vi "Mapper-main.vi"() -> ()   [LabVIEW 2022 SP3]
doc: "Demonstrates the fundamentals of the State Machine design pattern in LabVIEW. A state machine, in its simplest form, is a case structure within a while loop, with a state enum wired to a shift register on the loop to define the execution of different cases (or \"states\") of the case structure on different iterations of the loop."
uses:
  Subsystem modules/Messenger service/MessengerLib.lvlib
  Datatypes/TopStates.ctl
  Subsystem modules/Magnet module/ctl/Magnet Orders.ctl
  Subsystem modules/Magnet module/Magnet module.lvlib
  Subsystem modules/Magnet module/ctl/MSG to magnet.ctl
  Subsystem modules/Servo drive module/ctl/Axis names.ctl
  Subsystem modules/Servo drive module/Servo drive module.lvlib
  Subsystem modules/Servo drive module/ctl/Servo MSG.ctl
  Subsystem modules/Servo drive module/ctl/Servo commands.ctl
  Subsystem modules/Magnet module/ctl/SetField data.ctl
  Subsystem modules/Magnet module/ctl/RampingOutput.ctl
  Subsystem modules/Magnet module/ctl/Magnet mode.ctl
  Subsystem modules/Magnet module/ctl/Overall status.ctl
  Subsystem modules/Magnet module/ctl/TM Revision.ctl
  Subsystem modules/Servo drive module/ctl/Servo constants.ctl
  Subsystem modules/Servo drive module/ctl/Servo variables.ctl
  Subsystem modules/Servo drive module/ctl/Servo state.ctl
  Subsystem modules/Servo drive module/ctl/Status variable change.ctl
  Datatypes/Connected modules.ctl
  Subsystem modules/THz module/ctl/THz Message for module.ctl
  Subsystem modules/THz module/THz source modeule.lvlib
  Subsystem modules/Lock-in module/ctl/MFLI_command enum.ctl
  Subsystem modules/Lock-in module/Lock-in module.lvlib
  Subsystem modules/Lock-in module/ctl/MFLI_message for module.ctl
  Subsystem modules/Sample rotator/ctl/Rotator commands.ctl
  Subsystem modules/Sample rotator/SampleRotator.lvlib
  Subsystem modules/Magnet module/ctl/Magnet mode public.ctl
  Subsystem modules/Magnet module/ctl/Actual magnet state.ctl
  Subsystem modules/Sample rotator/ctl/Rotator controller info.ctl
  Subsystem modules/Sample rotator/ctl/Axis status.ctl
  Subsystem modules/Sample rotator/ctl/Positoin to set.ctl
  Subsystem modules/Sample rotator/ctl/Motion Properties.ctl
  Subsystem modules/Lock-in module/ctl/MFLI parameters.ctl
  <instrlib>/Zurich Instruments LabOne/Public/Data/ziTypeDemodSampleSingle.ctl
  <instrlib>/Zurich Instruments LabOne/Zurich Instruments LabOne.lvlib
  <instrlib>/Zurich Instruments LabOne/Public/ziTypeHandle.ctl
  Subsystem modules/THz module/ctl/THz sweep parameters.ctl
  Subsystem modules/THz module/ctl/Synth configs.ctl
  Subsystem modules/THz module/ctl/VDI config constants.ctl
  Subsystem modules/Sample rotator/ctl/MSG to Rotator.ctl
  Subsystem modules/Temperature control module/ctl/TC sensors.ctl
  Subsystem modules/Temperature control module/Temperature controller.lvlib
  Subsystem modules/Temperature control module/ctl/MSG for VTI.ctl
  Subsystem modules/Magnet module/ctl/Cryostat temperature sensors.ctl
  Datatypes/experiment state.ctl
  Subsystem modules/Temperature control module/ctl/TC commands.ctl
  Subsystem modules/Lock-in module/ctl/ACQ info.ctl
  Datatypes/SampleHolders.ctl
  <userlib>/_OpenG.lib/variantconfig/variantconfig.llb/openg_variant_configuration_file.lvlib
  <vilib>/Utility/config.llb/NI_LVConfig.lvlib
  Datatypes/Instr Info.ctl
  Subsystem modules/Lock-in module/ctl/MFLI_parameter and value.ctl
  Datatypes/Single servo status.ctl
  Datatypes/Measurement info.ctl
  Subsystem modules/Temperature control module/ctl/Set point.ctl
  Datatypes/THz parameters.ctl
  Subsystem modules/Lock-in module/ctl/MFLI_node.ctl
  <vilib>/Utility/sysdir.llb/System Directory Type.ctl
  Datatypes/Map parameters.ctl
  Datatypes/Map graph data.ctl
  Subsystem modules/THz module/ctl/THz commands enum.ctl
  Subsystem modules/Lock-in module/ctl/OSC sampling rate.ctl
  <vilib>/Analysis/NI_AALPro.lvlib
  <vilib>/Analysis/2dsp.llb/Decimate (single shot, DBL).vi
  Subsystem modules/Lock-in module/ctl/ADQ data.ctl
  Subsystem modules/Source meter/ctls/SMU status.ctl
  Subsystem modules/Source meter/Source meter.lvlib
  Subsystem modules/Source meter/ctls/SMU Commands.ctl
  Subsystem modules/Source meter/ctls/MSG to SMU.ctl
  Subsystem modules/Power monitor/PwrM status.ctl
  Subsystem modules/Power monitor/Power monitor.lvlib
  Datatypes/Magnet controls.ctl
  Datatypes/Servo controls.ctl
  Subsystem modules/Temperature control module/ctl/Set temperature.ctl
  Subsystem modules/Source meter/ctls/SMU settings.ctl
panel:
  in  "MW trig low [s]":dbl=0.5 format="%#_13g"
  out "data delay":dbl format="%.4g"
  out "Instr status":T1 caption="Connected \ninstuments"
  in  "Counter":u32
  out "rows":i32
  out "cols":i32
  out "tdms map file out":refnum<k34>
  in  "Line rate":dbl(ring)=1.118481 items=["1,1s"=1.118481, "2,2s"=2.236962, "4,5s"=4.473924, "9s"=8.947848]
  out "Controls referencies":T2
  out "Tmp [K]":T3
  out "Busy":bool
  in  "Stop":bool
  out "Review results":T4[](array[typedef])
  out "Magnetic\nfield state":bool
  out "data time":timestamp
  out "New data":bool
  out "Data":T5
  out "Instr control refs":refnum<vi>[](array[refnum])
  out "Tmp reched time":dbl format="%<%H:%M:%S>T"
  out "VTI tmp reached":bool
  out "Running experiment":bool
  out "Temperature log ref":refnum<file>
  out "1 round\ntime":u32
  out "loggersRef":refnum<file>
  in  "Tab Control":T6(tab)
  out "Drift[K/min]":dbl[](array[numeric])
  in  "Log folder":path=path "C:/HFEPR logs"
  in  "Disconnect":bool
  in  "Select module":T7(ring)
  out "Logger":string[](array[string])
  in  "Re-connect instruments":bool
  in  "System config file path":path=path "M:/Instrument/HFEPR spectrometer/Software developement/Multi-EPR plus ultra/SystemData/config.ini"
  out "Instr info":T8 {"PwrMonitor"."Last update" format="%<%H:%M:%S>T"; "VTI"."Last update" format="%<%H:%M:%S>T"; "PMD"."Last update" format="%<%H:%M:%S>T"; "SMU"."Last update" format="%<%H:%M:%S>T"; "Servo"."Last update" format="%<%H:%M:%S>T"; "Rotator"."Axes"."Actuator" items=["Linear", "Roatator", "Goniometer"]; "Rotator"."Name" items=["ANC350res", "ANC350num", "ANC350fps", "Unknown"]; "Rotator"."Last update" format="%<%H:%M:%S>T"; "THz"."Last update" format="%<%H:%M:%S>T"; "MFLI"."Last update" format="%<%H:%M:%S>T"; "Magnet"."Last update" format="%<%H:%M:%S>T"}
  in  "Use previous settings":bool=TRUE
  out "Temperature monitor":T12(graph)
  in  "Real instruments":bool=TRUE
  in  "Password is admin":string
  in  "Sample holder":T13
  in  "Acquisition controls":T15={"ACQ parameters"={"Filter order"=7.0, "Filter tau [ms]"=10.0, "F_Mod [kHz]"=1.0, "Amp_Mod [mV]"=10.0, "Enable output"=0, "Phase [°]"=0.0}, "ACQ shot btn"=FALSE, "Modulation [A]"=0.0, "In50"=FALSE, "Out50"=FALSE, "DemEn"=FALSE, "Mod_A [G]"=0.0} {"ACQ parameters"."Enable output" items=["Disable", "Enable"]; "ACQ parameters"."Amp_Mod [mV]" min=0.0 max=10000.0 format="%#_5f"; "ACQ parameters"."F_Mod [kHz]" min=0.1 max=500.0 format="%#_5f"; "ACQ parameters"."Filter order" min=1.0 max=10.0 step=1.0; "ACQ parameters"."Filter tau [ms]" min=0.0 max=1000.0 step=1.0 format="%#_4f"}
  in  "VID control":T16={"AMC"=9, "Multip"=1, "Base frequency [GHz]"=0.0, "End frequency [GHz]"=0.0, "Im frequency [MHz]"=1500.0, "Sweep up [ms]"=0.0, "Reset trigger?"=FALSE} {"Multip" items=["1"=1, "2"=2, "3"=3, "4"=4, "6"=6, "8"=8, "9"=9]; "AMC" items=["9"=9, "12"=12]; "End frequency [GHz]" min=0.00018 max=20000.0; "Base frequency [GHz]" min=162.0 max=252.0 format="%_5g"}
  in  "Servo controls":T17={"Y left"=FALSE, "Y right"=FALSE, "X backward"=FALSE, "X forward"=FALSE, "Zdown"=FALSE, "Zup"=FALSE, "Step\n[mm]"=5.0, "QO table"={"ZLdown"=FALSE, "ZLup"=FALSE, "ZRup"=FALSE, "ZRdown"=FALSE, "ZMdown"=FALSE, "ZMup"=FALSE}, "X"=0.0, "Y"=0.0, "ZL"=0.0, "ZR"=0.0, "ZM"=0.0, "Measure Position btn"=FALSE, "Eject position btn"=FALSE, "Stop servo btn"=FALSE, "Save position btn"=FALSE} {"Step\n[mm]" min=0.0 max=600.0 step=5.0}
  in  "Magnet controls":T18 {"Output\n[T]" scale=0.0..16.0; "Field\n[T]" scale=0.0..16.0; "Desired ramp\nrate [mT/s]" max=7.544966; "Set Field [T]" max=16.0}
  out "lookup":cluster{"X (Vrms)":dbl, "Y (Vrms)":dbl}(graph) caption="Waveform Chart - Dark"
  in  "SMU controls":T20={"Apply"=FALSE, "Measurement settings"={"Source Mode "=1, "Source Level"=0.001, "Source Limit"=0.3, "Measure Function"=0, "Remote sense"=TRUE, "Clear buffer?"=FALSE, "Beep"=TRUE, "High Capacity"=TRUE, "Terminals"=0, "PLCs"=1.0, "Fast measurement"=FALSE}, "Value"=0.1006, "Stop"=FALSE, "Record"=FALSE, "B[T]"=0.0, "Refresh"=FALSE} {"Value" format="%#_3e"; "Measurement settings"."Measure Function" items=["Volts", "Current", "Auto Resistance", "Manual Resistance", "Digitize Voltage", "Digitize Current"]; "Measurement settings"."Source Level" max=0.3; "Measurement settings"."Source Mode" items=["Voltage", "Current"]; "Measurement settings"."Terminals" items=["Front", "Rear"]}
  in  "VTI control":T21={"VTI space [K]"=1.0, "Sample [K]"=0.0, "Heater3 [K]"=1.8, "Heater4 [K]"=1.8, "Out 1 [%]"=0.0, "Out 2 [%]"=0.0, "Range out 1"=1} {"Range out 1" items=["Off", "Range 1 (On)", "Range 2", "Range 3", "Range 4", "Range 5"]; "Heater4 [K]" min=1.8 max=300.0; "Heater3 [K]" min=1.8 max=300.0}
  in  "Operator":string="Unknown"
  in  "Map parameters":T22={"B_start[T]"=0.0, "B_End[T]"=0.2, "B_rate [mT/s]"=1.0, "F_start[GHz]"=295.0, "F_end[GHz]"=0.0, "Sampling rate"=13, "Tmp [K]"=295.0, "Wait[min]"=0.0, "Points"=4096, "Display signal"=enum."X", "Signal treat"=enum."None", "Sweep [s]"=2.0} {"Points" min=4096 max=5000000; "Sampling rate" items=["117 ks/S"=9, "58.6 kS/s"=10, "29.3 kS/s"=11, "14.6 kS/s"=12, "7.32 kS/s"=13, "3.66 kS/s"=14, "1.83 kS/s"=15]}
  out "EPR map":sgl[][](graph)
  in  "Folder path":path
  in  "Description":string
  in  "Sample name":string="Unknown"
  in  "Run MAP btn":bool
  in  "Direct stop meas. btn":bool
  out "Infobar":T24 {"Started" format="%<%H:%M:%S>T"; "Remains" format="%<%H:%M:%S>t"}
  out "Spectrum":dbl[](graph)
  in  "File Path Control":path
  out "Cursor Amplitude":dbl
  out "Cursor [T]":dbl
  out "Cursor [GHz]":dbl
  out "Review Header":string[](array[string])
  out "EPR review graph":cluster{"X":dbl, "Y":dbl}[](graph)
  out "FDMR review graph":dbl[](graph)
  out "Map review graph":dbl[][](graph)
  in  "Open measurement":bool
  in  "Data file to show":u16(ring) items=["Empty", "Empty", "Empty"]
  # "Action part"
  # "Status part"
  # "Option 1:\nchoice primary and secondary sweep\n\nOption 2:\nChoice measurement mode, and appropriate cluster will apear. Other clusters wil be hidden.\n\n\nOption 3:\nChoice measurement mode.\nInternal parts of single cluster will (dis)apear if needed.\n\nNote:\nPosibility to do an orientation/temperature deppendency."
  # "Tmp [K]"
  # "Position [mm]"
  # "Z"
  # "X/Y"
  # "This software was developed for HFEPR spectrometer in 2019 (2020) at CEITEC BUT by members of MOTES research group.\n\nQuick guide:\n1) Re-connect to all instruments.\n2) Check if necessary instruments are ready. (At least VTI, VDI, Lock-In, and Magnet has to work)\n3) Go to Adjustment tab and set up Lock-in parameters as well as VDI multipiers.\n4) Go to EPR measurement tab, select folder path, fill the sample description.\n5) Fill at least 1 line of the script and press Run script button.\n\n6) In case of a bug please report this to software developer or make a note into developement diary loaceted at:\n    RG-1-12/Instriments/HFEPR spectrometer/Software developement.\n\nLast update: 07.02. 2020 - Script editor is working, measurement review not yet.\n\nSpecial thanks to: Luke Skywalker, my mom, Tonda's mom, Pilsner, God, Oleksi, Vinicius, Petr from parallel universe.\n\n \nTODO: Invisible controls: referencies for: adjustment controls, meas results, loggerRef,"
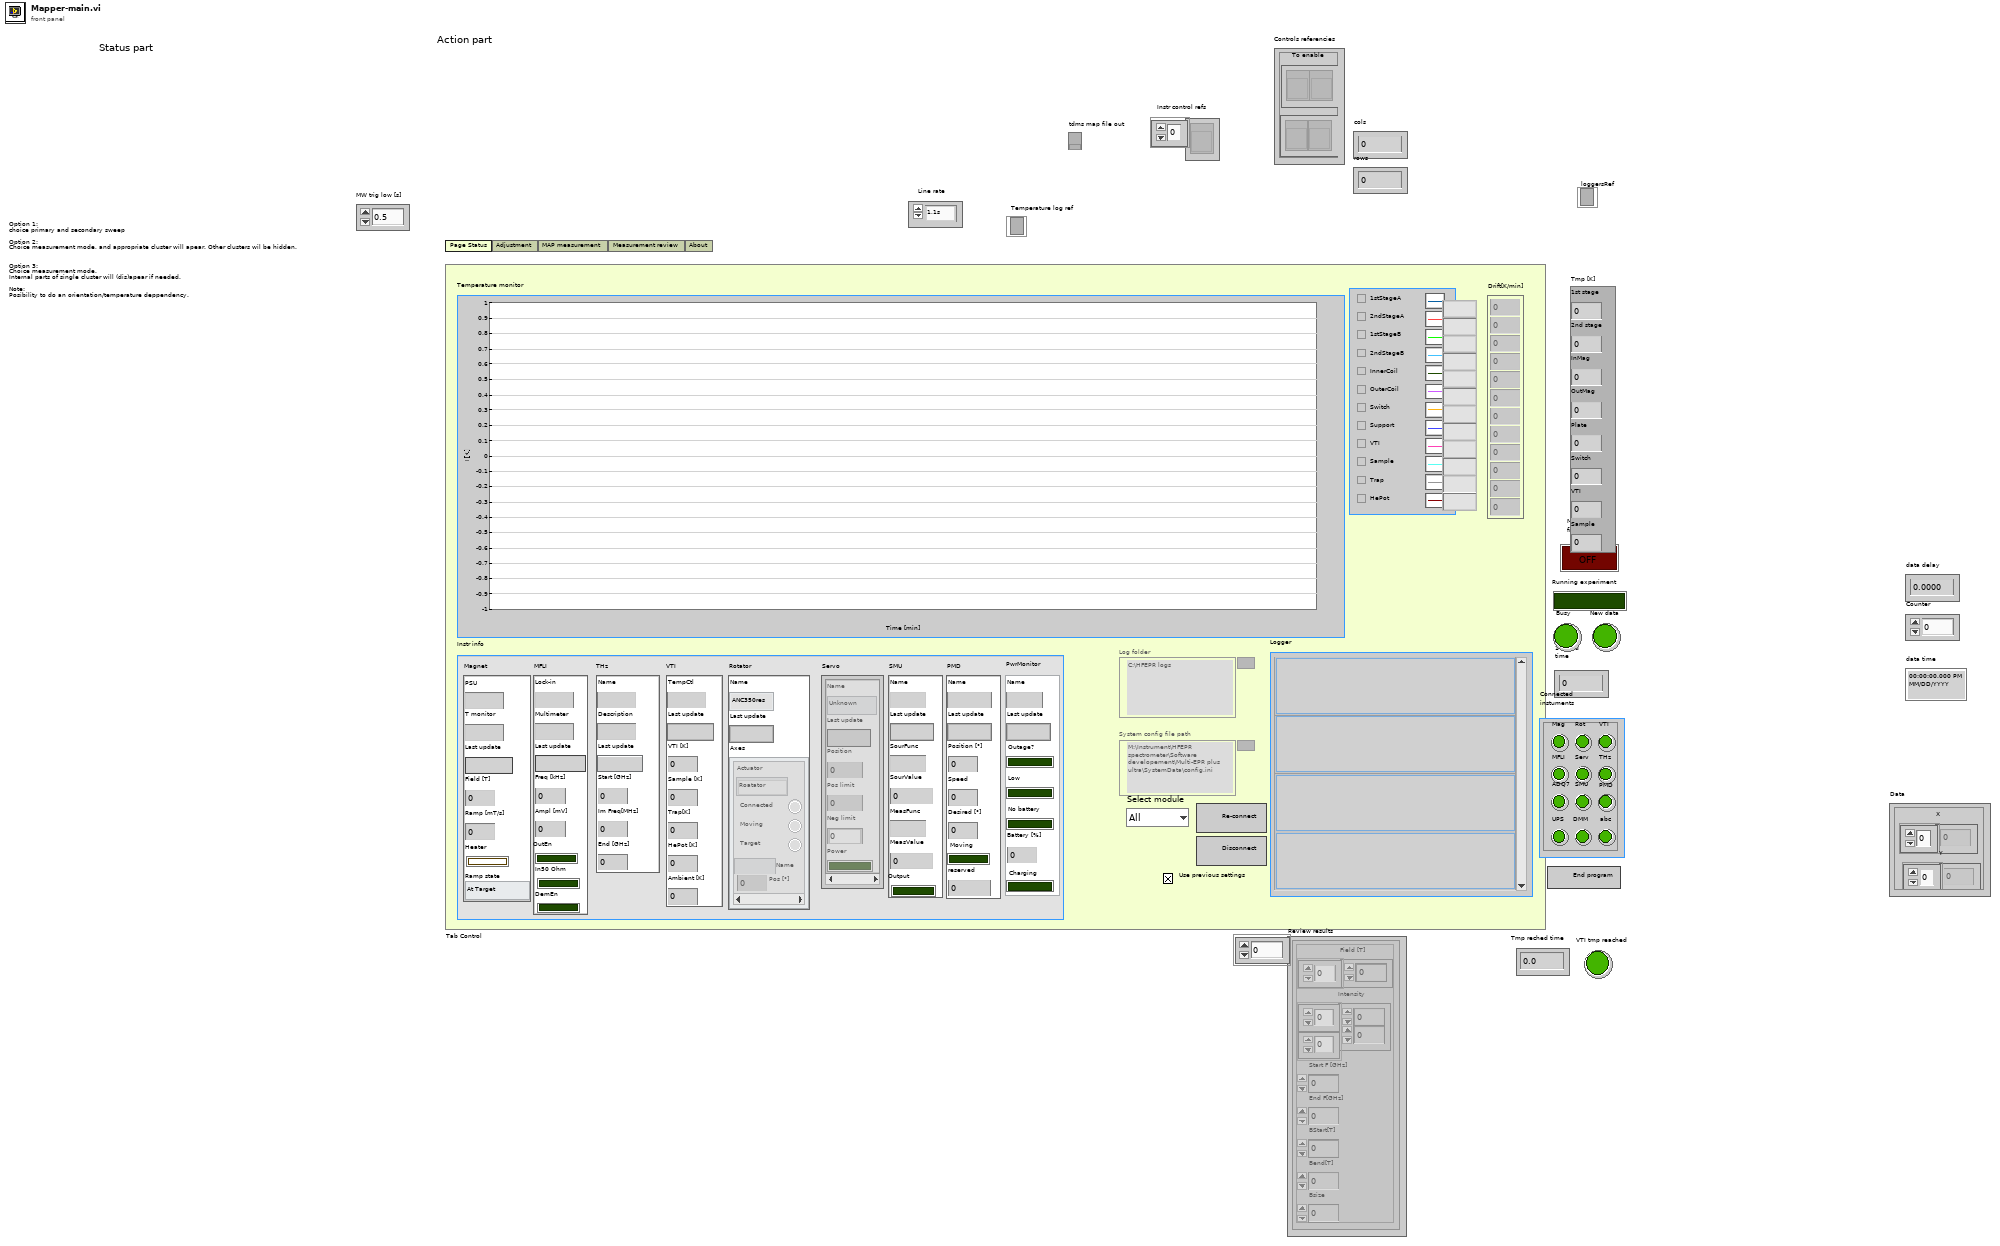
[diagram p1: front panel]
types:
  T1 = typedef "Connected modules.ctl" = cluster{"Mag":bool, "Rot":bool, "VTI":bool, "MFLI":bool, "Serv":bool, "THz":bool, "ADQ7":bool, "SMU":bool, "PMD":bool, "UPS":bool, "DMM":bool, "abc":bool}
  T2 = cluster{"To disable":refnum<vi>[], "To enable":refnum<vi>[]}
  T3 = cluster{"1st stage":dbl, "2nd stage":dbl, "InMag":dbl, "OutMag":dbl, "Plate":dbl, "Switch":dbl, "VTI":dbl, "Sample":dbl}
  T4 = typedef "Map graph data.ctl" = cluster{"Field [T]":dbl[], "Intensity":dbl[][], "Start F [GHz]":dbl, "End F[GHz]":dbl, "BStart[T]":dbl, "Bend[T]":dbl, "Bsize":i32}
  T5 = typedef "Lock-in module.lvlib/ADQ data.ctl" = cluster{"X":sgl[], "Y":sgl[]}
  T6 = enum32{"Page Status", "Adjustment", "MAP measurement", "Measurement review", "About"}
  T7 = enum16{"All", "None", "ACQ", "THz", "MAG", "SERV", "ROT", "VTI", "SMU"}
  T8 = typedef "Instr Info.ctl" = cluster{"Magnet":cluster{"PSU":string, "T monitor":string, "Last update":timestamp, "Field [T]":dbl, "Ramp [mT/s]":dbl, "Heater":bool, "Ramp state":T9}, "MFLI":cluster{"Lock-in":string, "Multimeter":string, "Last update":timestamp, "Freq [kHz]":dbl, "Ampl [mV]":dbl, "OutEn":bool, "In50 Ohm":bool, "DemEn":bool}, "THz":cluster{"Name":string, "Description":string, "Last update":timestamp, "Start [GHz]":dbl, "Im Freq[MHz]":dbl, "End [GHz]":dbl}, "VTI":cluster{"TempCtl":string, "Last update":timestamp, "VTI [K]":dbl, "Sample [K]":dbl, "Trap[K]":dbl, "HePot [K]":dbl, "Ambient [K]":dbl}, "Rotator":cluster{"Name":i32, "Last update":timestamp, "Axes":cluster{"Pos [°]":dbl, "Moving":bool, "Name":string, "Actuator":u16, "Target":bool, "Connected":bool}[]}, "Servo":T10[], "SMU":cluster{"Name":string, "Last update":timestamp, "SourFunc":string, "SourValue":dbl, "MeasFunc":string, "MeasValue":dbl, "Output":bool}, "PMD":cluster{"Name":string, "Last update":timestamp, "Position [°]":dbl, "Speed":dbl, "Desired [°]":dbl, "Moving":bool, "reserved":dbl}, "PwrMonitor":cluster{"Name":string, "Last update":timestamp, "Outage?":bool, "Low":bool, "No battery":bool, "Battery [%]":u8, "Charging":bool}}
  T9 = typedef "Magnet module.lvlib/RampingOutput.ctl" = enum16{"At Target", "Go up", "Go down"}
  T10 = typedef "Single servo status.ctl" = cluster{"Name":T11, "Last update":timestamp, "Position":dbl, "Pos limit":dbl, "Neg limit":dbl, "Power":bool}
  T11 = typedef "Servo drive module.lvlib/Axis names.ctl" = enum16{"Unknown", "AxisX", "AxisY", "AxisZ_left", "AxisZ_middle", "AxisZ_right"}
  T12 = cluster{"[0]":dbl, "[1]":dbl, "[2]":dbl, "[3]":dbl, "[4]":dbl, "[5]":dbl, "[6]":dbl, "[7]":dbl, "[8]":dbl, "[9]":dbl, "[10]":dbl, "[11]":dbl}
  T13 = typedef "SampleHolders.ctl" = enum16{"Simple", "Carousel", "Chip", "Rotator", "Liquid"}
  T14 = typedef "Lock-in module.lvlib/MFLI parameters.ctl" = cluster{"Filter order":dbl, "Filter tau [ms]":dbl, "F_Mod [kHz]":dbl, "Amp_Mod [mV]":dbl, "Enable output":u16, "Phase [°]":dbl}
  T15 = cluster{"ACQ parameters":T14, "ACQ shot btn":bool, "Modulation [A]":dbl, "In50":bool, "Out50":bool, "DemEn":bool, "Mod_A [G]":dbl}
  T16 = typedef "THz parameters.ctl" = cluster{"AMC":u16, "Multip":u16, "Base frequency [GHz]":dbl, "End frequency [GHz]":dbl, "Im frequency [MHz]":dbl, "Sweep up [ms]":dbl, "Reset trigger?":bool}
  T17 = typedef "Servo controls.ctl" = cluster{"Y left":bool, "Y right":bool, "X backward":bool, "X forward":bool, "Zdown":bool, "Zup":bool, "Step\n[mm]":dbl, "QO table":cluster{"ZLdown":bool, "ZLup":bool, "ZRup":bool, "ZRdown":bool, "ZMdown":bool, "ZMup":bool}, "X":dbl, "Y":dbl, "ZL":dbl, "ZR":dbl, "ZM":dbl, "Measure Position btn":bool, "Eject position btn":bool, "Stop servo btn":bool, "Save position btn":bool}
  T18 = typedef "Magnet controls.ctl" = cluster{"Set Field [T]":dbl, "Desired ramp\nrate [mT/s]":dbl, "Custom\nramp":bool, "Mode switch":bool, "Pause ramp":bool, "Field\n[T]":dbl, "Output\n[T]":dbl, "Equalize":bool, "Discharge":bool, "Switch \ntmp [K]":dbl, "Direction":bool}
  T19 = typedef "SMU settings.ctl" = cluster{"Source Mode ":u16, "Source Level":dbl, "Source Limit":dbl, "Measure Function":u16, "Remote sense":bool, "Clear buffer?":bool, "Beep":bool, "High Capacity":bool, "Terminals":u16, "PLCs":dbl, "Fast measurement":bool}
  T20 = cluster{"Apply":bool, "Measurement settings":T19, "Value":dbl, "Stop":bool, "Record":bool, "B[T]":dbl, "Refresh":bool}
  T21 = typedef "Temperature controller.lvlib/Set temperature.ctl" = cluster{"VTI space [K]":dbl, "Sample [K]":dbl, "Heater3 [K]":dbl, "Heater4 [K]":dbl, "Out 1 [%]":dbl, "Out 2 [%]":dbl, "Range out 1":u16}
  T22 = typedef "Map parameters.ctl" = cluster{"B_start[T]":dbl, "B_End[T]":dbl, "B_rate [mT/s]":dbl, "F_start[GHz]":dbl, "F_end[GHz]":dbl, "Sampling rate":T23, "Tmp [K]":dbl, "Wait[min]":dbl, "Points":u32, "Display signal":enum16{"X", "Y", "R", "Phi"}, "Signal treat":enum16{"None", "Unity norm", "Mean norm", "Standardization"}, "Sweep [s]":dbl}
  T23 = typedef "OSC sampling rate.ctl" = u16
  T24 = typedef "Measurement info.ctl" = cluster{"Remains":dbl, "T_sample [K]":dbl, "Last log":string, "Experiment state":T25, "Field [T]":dbl, "Sample holder":T13, "Started":timestamp}
  T25 = typedef "experiment state.ctl" = enum16{"Setup", "Preparation", "Stabilization", "Begin", "Acquisition", "Save"}
  T26 = typedef "Instr Info.ctl" = cluster{"Magnet":cluster{"PSU":string, "T monitor":string, "Last update":timestamp, "Field [T]":dbl, "Ramp [mT/s]":dbl, "Heater":bool, "Ramp state":T9}, "ACQ":cluster{"Lock-in":string, "Multimeter":string, "Last update":timestamp, "Freq [kHz]":dbl, "Ampl [mV]":dbl, "OutEn":bool, "In50 Ohm":bool, "DemEn":bool}, "THz":cluster{"Name":string, "Description":string, "Last update":timestamp, "Start [GHz]":dbl, "Im Freq[MHz]":dbl, "End [GHz]":dbl}, "VTI":cluster{"TC":string, "Last update":timestamp, "VTI [K]":dbl, "Sample [K]":dbl, "Trap[K]":dbl, "HePot [K]":dbl, "Ambient [K]":dbl}, "Rot":cluster{"Name":u16, "Last update":timestamp, "Actuator":u16, "Connected":bool, "Moving":bool, "Target":bool, "Cap [nF]":dbl, "Position [°]":dbl}, "Servo":T10[], "SMU":cluster{"Name":string, "Last update":timestamp, "Source F":string, "Source V":dbl, "Measure F":string, "Measure V":dbl, "Output":bool}, "PMD":cluster{"Name":string, "Last update":timestamp, "Position [°]":dbl, "Speed":dbl, "Desired [°]":dbl, "Moving":bool, "reserved":dbl}, "PwrM":T27}
  T27 = typedef "Power monitor.lvlib/PwrM status.ctl" = cluster{"Name":string, "Last update":timestamp, "Outage?":bool, "Low":bool, "No battery":bool, "Battery [%]":u8, "Charging":bool}
  T28 = typedef "TopStates.ctl" = enum16{"Initialize GUI", "Wait for Event", "Check message", "Check measurement", "Stop", "Restart"}
  T29 = typedef "MessengerLib.lvlib/Messenger referencies.ctl" = cluster{"TOP":refnum<queue>, "Instr_M":refnum<queue>, "Field_C":refnum<queue>, "Tmp_M":refnum<queue>, "Tmp_C":refnum<queue>, "Table_C":refnum<queue>, "MW_C":refnum<queue>, "Data_Aq":refnum<queue>, "Mod_M":refnum<queue>, "Field_M":refnum<queue>, "Pwr_M":refnum<queue>, "Angle_C":refnum<queue>, "Sample_C":refnum<queue>, "Reserved":refnum<queue>}
  T30 = enum16{"fire", "rainbow", "gray", "inverse gray", "ice", "original"}
  T31 = enum16{"All", "None", "ACQ", "THz", "MAG", "SERV", "ROT", "VTI"}
  T32 = enum8{"Enabled", "Disabled", "Disabled and Grayed Out"}
  T33 = typedef "Magnet module.lvlib/Magnet mode public.ctl" = enum16{"Persistant", "Ramping"}
  T34 = typedef "Magnet module.lvlib/SetField data.ctl" = cluster{"Field [T]":dbl, "Ramp [T/s]":dbl, "Custom Ramp?":bool, "Mode":T33}
  T35 = typedef "Magnet module.lvlib/Magnet Orders.ctl" = enum16{"Ignore", "Connect", "Update", "Switch mode", "Set field", "Stop ramping", "Equalize output", "Zero output", "Flip polarity", "Blackout", "Set timer", "Eval temperatures", "Disconnect"}
  T36 = typedef "Magnet module.lvlib/MSG to magnet.ctl" = cluster{"Command":T35, "Data":variant}
  T37 = typedef "Source meter.lvlib/MSG to SMU.ctl" = cluster{"Command":T38, "Data":variant}
  T38 = typedef "Source meter.lvlib/SMU Commands.ctl" = enum16{"Ignore", "Connect", "Update", "Set measurement", "Start measurement", "Get actual results", "Stop measurement", "Disconnect", "End"}
  T39 = typedef "Servo drive module.lvlib/Servo commands.ctl" = enum16{"Initialize", "Update", "Move by", "Move to", "Stop", "Ignore", "Disconnect", "End"}
  T40 = typedef "Servo drive module.lvlib/Servo MSG.ctl" = cluster{"Command":T39, "Data":variant}
  T41 = typedef "THz source modeule.lvlib/THz commands enum.ctl" = enum16{"Ignore", "Connect", "Update", "Set parameters", "Disconnect", "End"}
  T42 = typedef "THz source modeule.lvlib/THz sweep parameters.ctl" = cluster{"Start [GHz]":dbl, "End [GHz] ":dbl, "Sweep up\ntime [ms]":dbl, "Sweep down\ntime [ms]":dbl, "Intermidiate [MHz]":dbl, "Reset trigger":bool}
  T43 = typedef "THz source modeule.lvlib/THz Message for module.ctl" = cluster{"Command":T41, "Data":variant}
  T44 = typedef "Lock-in module.lvlib/MFLI_parameter and value.ctl" = cluster{"parameter":T45, "value":dbl}
  T45 = typedef "Lock-in module.lvlib/MFLI_node.ctl" = enum16{"None", "filter_order [-]", "filter_constant [ms]", "in_diff", "in_autorange", "in_imp50", "in_AC", "osc_freq [kHz]", "out_ampl [V]", "out_autorange", "out_imp50", "enable output", "enamble ampl", "scope_enable", "scope_rate", "scope_len", "scope_trigEn", "AuxOut_amplify", "Phase_deg", "AuxOut_select"}
  T46 = typedef "Lock-in module.lvlib/MFLI_command enum.ctl" = enum16{"Initialize", "Update", "Set parameters", "Set module", "Set individual parameters", "Get point", "Get array", "Disconnect", "End", "Ignore"}
  T47 = typedef "Lock-in module.lvlib/MFLI_message for module.ctl" = cluster{"Command":T46, "Data":variant}
  T48 = typedef "Temperature controller.lvlib/Set point.ctl" = cluster{"Heater":string, "Tmp [K]":dbl}
  T49 = typedef "Temperature controller.lvlib/TC commands.ctl" = enum16{"Initialize", "Update", "Stop tmp change", "Set temperature", "Set point", "Disconnect", "End", "Ignore"}
  T50 = typedef "Temperature controller.lvlib/MSG for VTI.ctl" = cluster{"Command":T49, "Data":variant}
  T51 = typedef "SampleRotator.lvlib/MSG to Rotator.ctl" = cluster{"Command":T52, "Data":variant}
  T52 = typedef "SampleRotator.lvlib/Rotator commands.ctl" = enum16{"Ignore", "Initialize", "Initialize axes", "Update", "Set parameters", "Stop movement", "Set position", "Disconnect", "End"}
  T53 = typedef "THz source modeule.lvlib/VDI config constants.ctl" = cluster{"Master":T54, "Follower":T54}
  T54 = typedef "THz source modeule.lvlib/Synth configs.ctl" = cluster{"Lower limit [GHz]":dbl, "Upper limit [GHz]":dbl, "Name":string, "Handle":string, "Description":string}
  T55 = typedef "THz source modeule.lvlib/THz Message for module.ctl" = cluster{"Command":T56, "Data":variant}
  T56 = typedef "THz source modeule.lvlib/THz commands enum.ctl" = enum16{"Ignore", "Initialize", "Update", "Set parameters", "Disconnect", "End"}
  T57 = typedef "Magnet module.lvlib/TM Revision.ctl" = cluster{"Instr Serial Number":string, "Instr Driver Revision":string, "Instr Firmware Revision":string, "Instr Model Number":string}
  T58 = typedef "Magnet module.lvlib/Overall status.ctl" = cluster{"Desired":T34, "Actual":T59}
  T59 = typedef "Magnet module.lvlib/Actual magnet state.ctl" = cluster{"Mode":T60, "Ramping output":T9, "Ready for change":bool, "Switch heater":bool, "Cooler Overheat":bool, "Coil overheat":bool, "Energized":bool, "Output [T]":dbl, "Field [T]":dbl, "Ramp[T/s]":dbl, "Switch\ntemperature [K]":dbl, "Voltage [V]":dbl, "Current direction":bool}
  T60 = typedef "Magnet module.lvlib/Magnet mode.ctl" = enum16{"Persistant", "Switching", "Ramping", "Quenched"}
  T61 = typedef "Magnet module.lvlib/Cryostat temperature sensors.ctl" = cluster{"First stage A [K]":dbl, "Second stage A [K]":dbl, "Firs stage B [K]":dbl, "Second stage B [K]":dbl, "Inner magnet [K]":dbl, "Outer Magnet [K]":dbl, "Switch [K]":dbl, "Support plate [K]":dbl, "Time stamp":dbl}
  T62 = typedef "Lock-in module.lvlib/ACQ info.ctl" = cluster{"In50":bool, "InAC":bool, "InDiff":bool, "Out50":bool, "OutEN":bool, "OutF[Hz]":dbl, "OutA[V]":dbl, "DemEN":bool, "Const[ms]":dbl, "Order[-]":i32, "Phase [°]":dbl}
  T63 = enum32{"Page Status", "Adjustment", "EPR measurement", "About"}
  T64 = typedef "Zurich Instruments LabOne.lvlib/ziTypeDemodSampleSingle.ctl" = cluster{"Timestamps (ticks)":u64, "X (Vrms)":dbl, "Y (Vrms)":dbl, "Osc Phase (deg)":dbl, "Freq (Hz)":dbl, "DIO":u32, "AuxIn0 (V)":dbl, "AuxIn1 (V)":dbl, "Trigger":u32}
  T65 = typedef "Zurich Instruments LabOne.lvlib/ziTypeHandle.ctl" = cluster{"handleValid":bool, "Conn":u64, "Path Prefix":string, "Handle":u64, "Connected":bool, "Clockbase(s)":dbl}
  T66 = typedef "Source meter.lvlib/SMU status.ctl" = cluster{"VISA name":refnum<visa-resource-name>, "Connected":bool, "Name":string, "Message":string, "Error message":string, "Min voltage":dbl, "Max voltage":dbl, "Min Current":dbl, "Max Current":dbl, "Measurement value":dbl, "Source Voltage":dbl, "Measurement":bool, "Source Current":dbl, "Source Mode":u16, "Measure Function":u16}
  T67 = typedef "Temperature controller.lvlib/TC sensors.ctl" = cluster{"VTI space":dbl, "Sample":dbl, "He pot":dbl, "Trap":dbl, "Ambient":dbl, "SetP_VTI":dbl, "SetP_Smp":dbl, "SetP_Pot":dbl, "SetP_Trap":dbl, "Range out 1":u16, "Out 1 [%]":dbl, "Out 2 [%]":dbl}
  T68 = typedef "Servo drive module.lvlib/Servo state.ctl" = cluster{"Servo variables":T69, "Servo constants":T70, "Connection":variant}
  T69 = typedef "Servo drive module.lvlib/Servo variables.ctl" = cluster{"Terget reached":bool, "Connected":bool, "Power ON":bool, "Operation mode":bool, "Actual position":dbl, "Target position":dbl}
  T70 = typedef "Servo drive module.lvlib/Servo constants.ctl" = cluster{"Name":T11, "Pos position limit [mm]":dbl, "Neg position limit [mm]":dbl, "Pos velocity limit":dbl, "Neg velocity limit":dbl, "Acceleration limit":dbl}
  T71 = typedef "Servo drive module.lvlib/Status variable change.ctl" = cluster{"Property":string, "Value":variant, "Name":T11}
  T72 = typedef "SampleRotator.lvlib/Rotator controller info.ctl" = cluster{"deviceNumber":i32, "DeviceType":i32, "ID":u32, "Serial":string, "Address":string, "connected":bool}
  T73 = typedef "SampleRotator.lvlib/Axis status.ctl" = cluster{"Axis status":cluster{"Connected":bool, "Enabled":bool, "Moving":bool, "Target":bool, "EndForward":bool, "EndBackarwd":bool, "Error":bool}, "Position [°]":dbl, "Frequency [Hz]":dbl, "Voltage [V]":dbl, "Capacitance[uF]":dbl, "Name":string, "ActuatorType":u16, "DC offset [V]":dbl, "Tolerance [m°]":dbl, "Index":u8}
  T74 = typedef "Motion Properties.ctl" = cluster{"Frequency [Hz]":dbl, "MaxErr [µm|m°]":dbl, "DC voltage [V]":dbl, "Amplitude [V]":dbl, "Position [mm|°]":dbl, "EoF":bool, "EoB":bool, "Error":bool, "Target [mm|°]":dbl}
  T75 = typedef "Positoin to set.ctl" = cluster{"Relative?":bool, "Position [°]":dbl, "Safe to move?":bool}
  T76 = typedef "NI_LVConfig.lvlib/Config Data RefNum.ctl" = refnum<k1>
  T77 = typedef "System Directory Type.ctl" = i32
  T78 = cluster{"Field [T]":dbl[], "Intensity":dbl[][], "Start F [GHz]":dbl, "End F[GHz]":dbl, "BStart[T]":dbl, "Bend[T]":dbl, "Bsize":i32}
  T79 = typedef "Mudules status.ctl" = cluster{"Mag":bool, "Rot":bool, "VTI":bool, "MFLI":bool, "Serv":bool, "THz":bool, "ADQ7":bool, "SMU":bool, "PMD":bool, "UPS":bool, "DMM":bool, "abc":bool}
  T80 = typedef "Magnet module.lvlib/Magnet config constants.ctl" = cluster{"Switch resistant [K]":dbl, "Switch superconducting [K]":dbl, "First stage critical temperature [K]":dbl, "Second stage critical temperature [K]":dbl, "Inner magnet critical temperature [K]":dbl, "Outer magnet critical temperature [K]":dbl, "Field Constant [T/A]":dbl, "Maximum Current [A]":dbl, "Maximum field [T]":dbl, "Maximum source ramp [A/s]":dbl, "Source precision [T]":dbl, "Ramp limits [A/s]":dbl[], "Field limits [T]":dbl[], "SMS":refnum<visa-resource-name>, "LSC218":refnum<visa-resource-name>}
  T81 = typedef "MessengerLib.lvlib/MSG to TOP.ctl" = cluster{"Module":T82, "Response":string, "Data":variant, "Time":timestamp}
  T82 = typedef "Module name.ctl" = enum16{"Emty", "Magnet", "VTI", "Excitation", "Servo", "Acquisition", "Rotator", "Digitizer", "SMU2450", "Carousel", "Multimeter", "Tmp monitor", "Power monitor"}
  T83 = cluster{"PSU":string, "T monitor":string, "Last update":timestamp, "Field [T]":dbl, "Ramp [mT/s]":dbl, "Heater":bool, "Ramp state":T9}
  T84 = cluster{"TC":string, "Last update":timestamp, "VTI [K]":dbl, "Sample [K]":dbl, "Trap[K]":dbl, "HePot [K]":dbl, "Ambient [K]":dbl}
  T85 = cluster{"Name":string, "Description":string, "Last update":timestamp, "Start [GHz]":dbl, "Im Freq[MHz]":dbl, "End [GHz]":dbl}
  T86 = cluster{"Lock-in":string, "Multimeter":string, "Last update":timestamp, "Freq [kHz]":dbl, "Ampl [mV]":dbl, "OutEn":bool, "In50 Ohm":bool, "DemEn":bool}
  T87 = cluster{"Name":string, "Last update":timestamp, "Source F":string, "Source V":dbl, "Measure F":string, "Measure V":dbl, "Output":bool}
  T88 = cluster{"Name":u16, "Last update":timestamp, "Actuator":u16, "Connected":bool, "Moving":bool, "Target":bool, "Cap [nF]":dbl, "Position [°]":dbl}
  T89 = enum16{"None", "Unity norm", "Mean norm", "Standardization"}
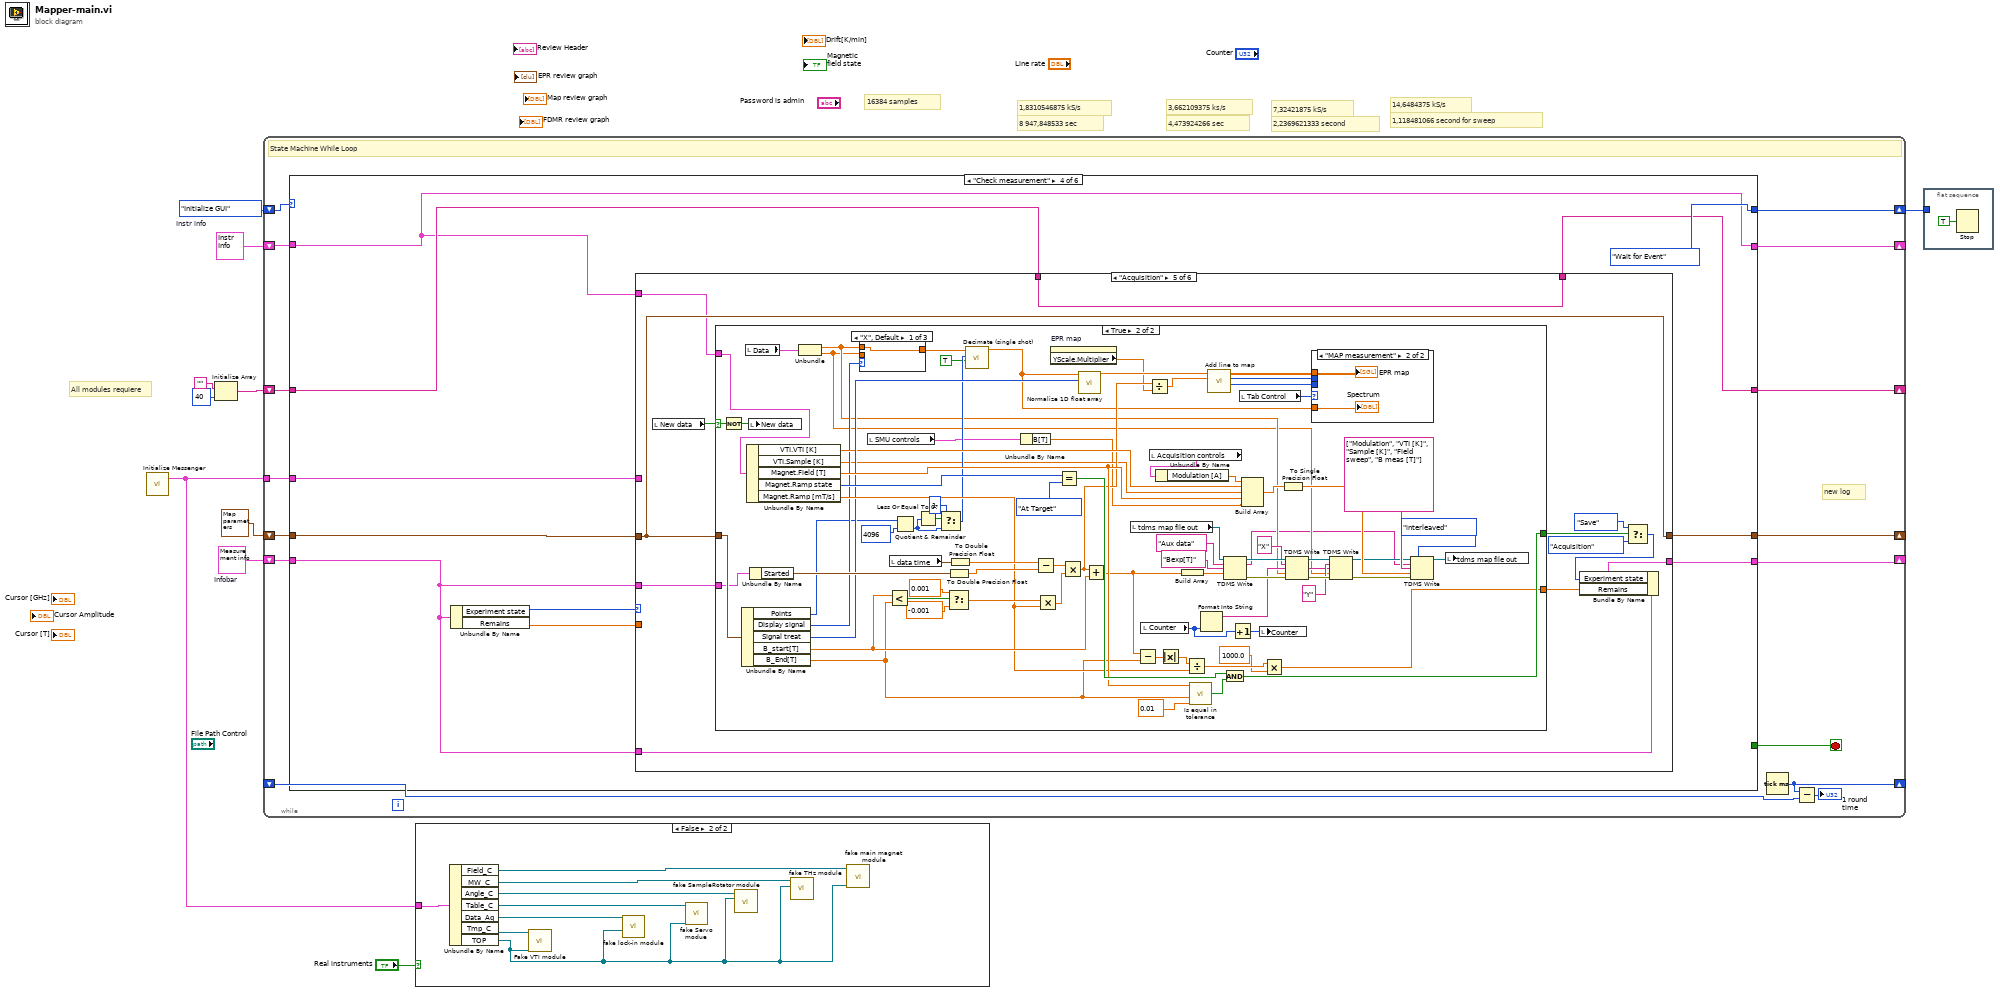
[diagram p0: block diagram]
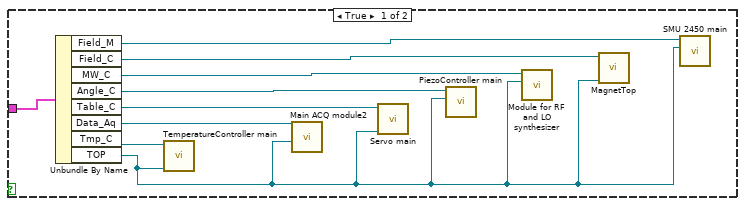
[diagram p2: hidden frame]
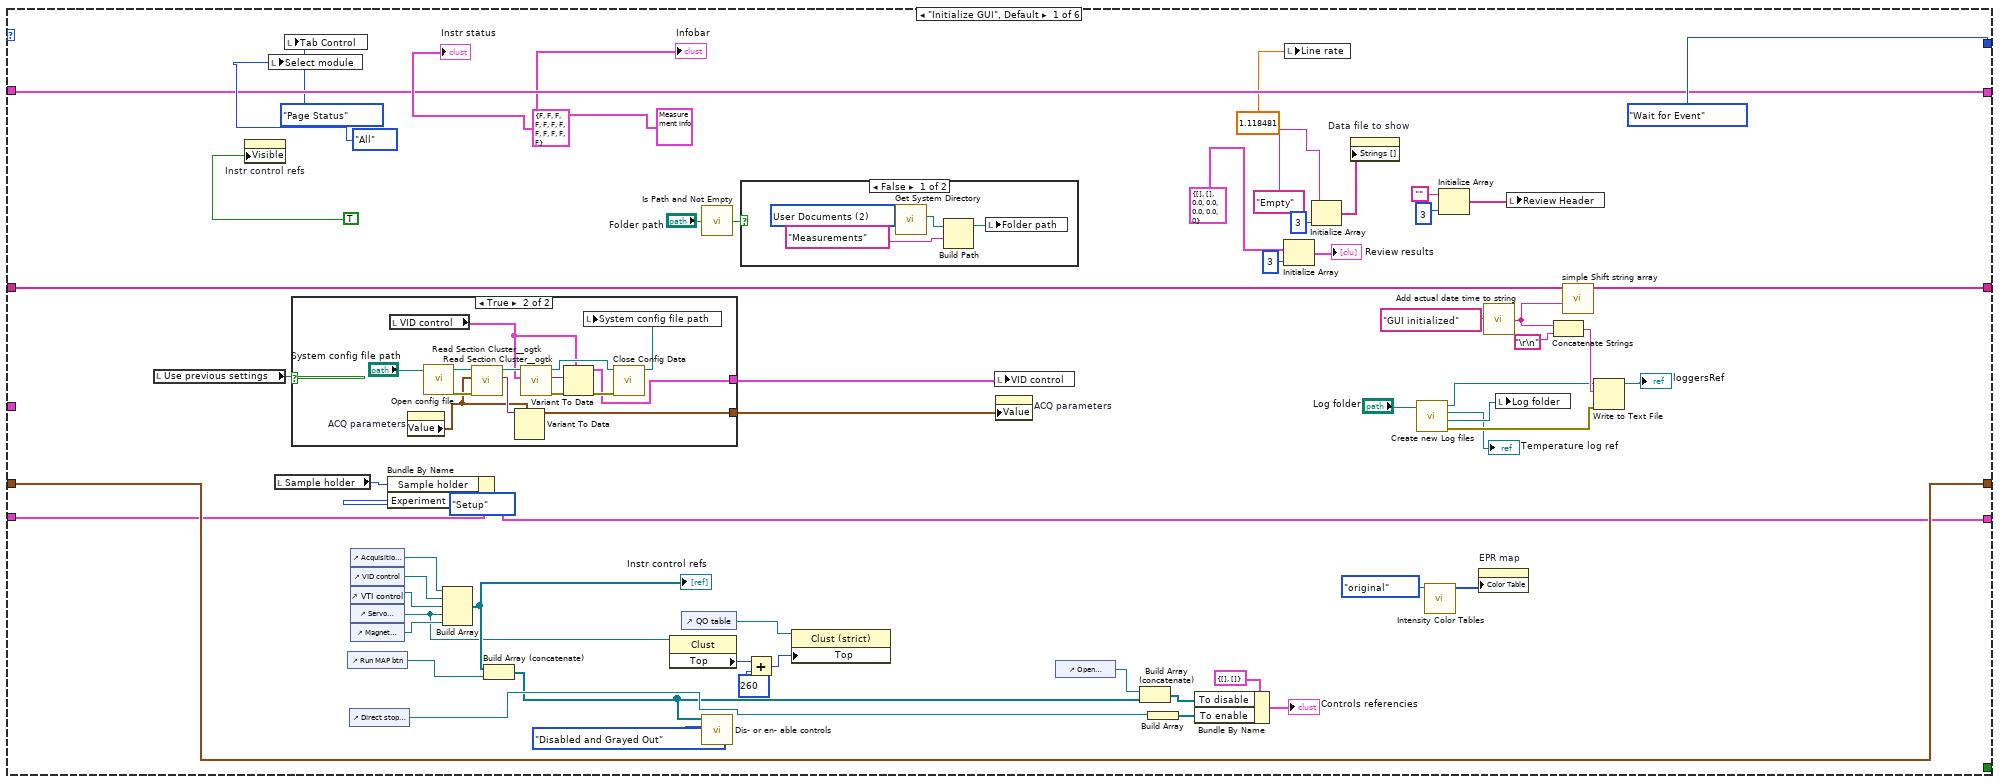
[diagram p3: hidden frame]
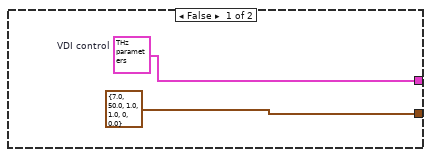
[diagram p5: hidden frame]
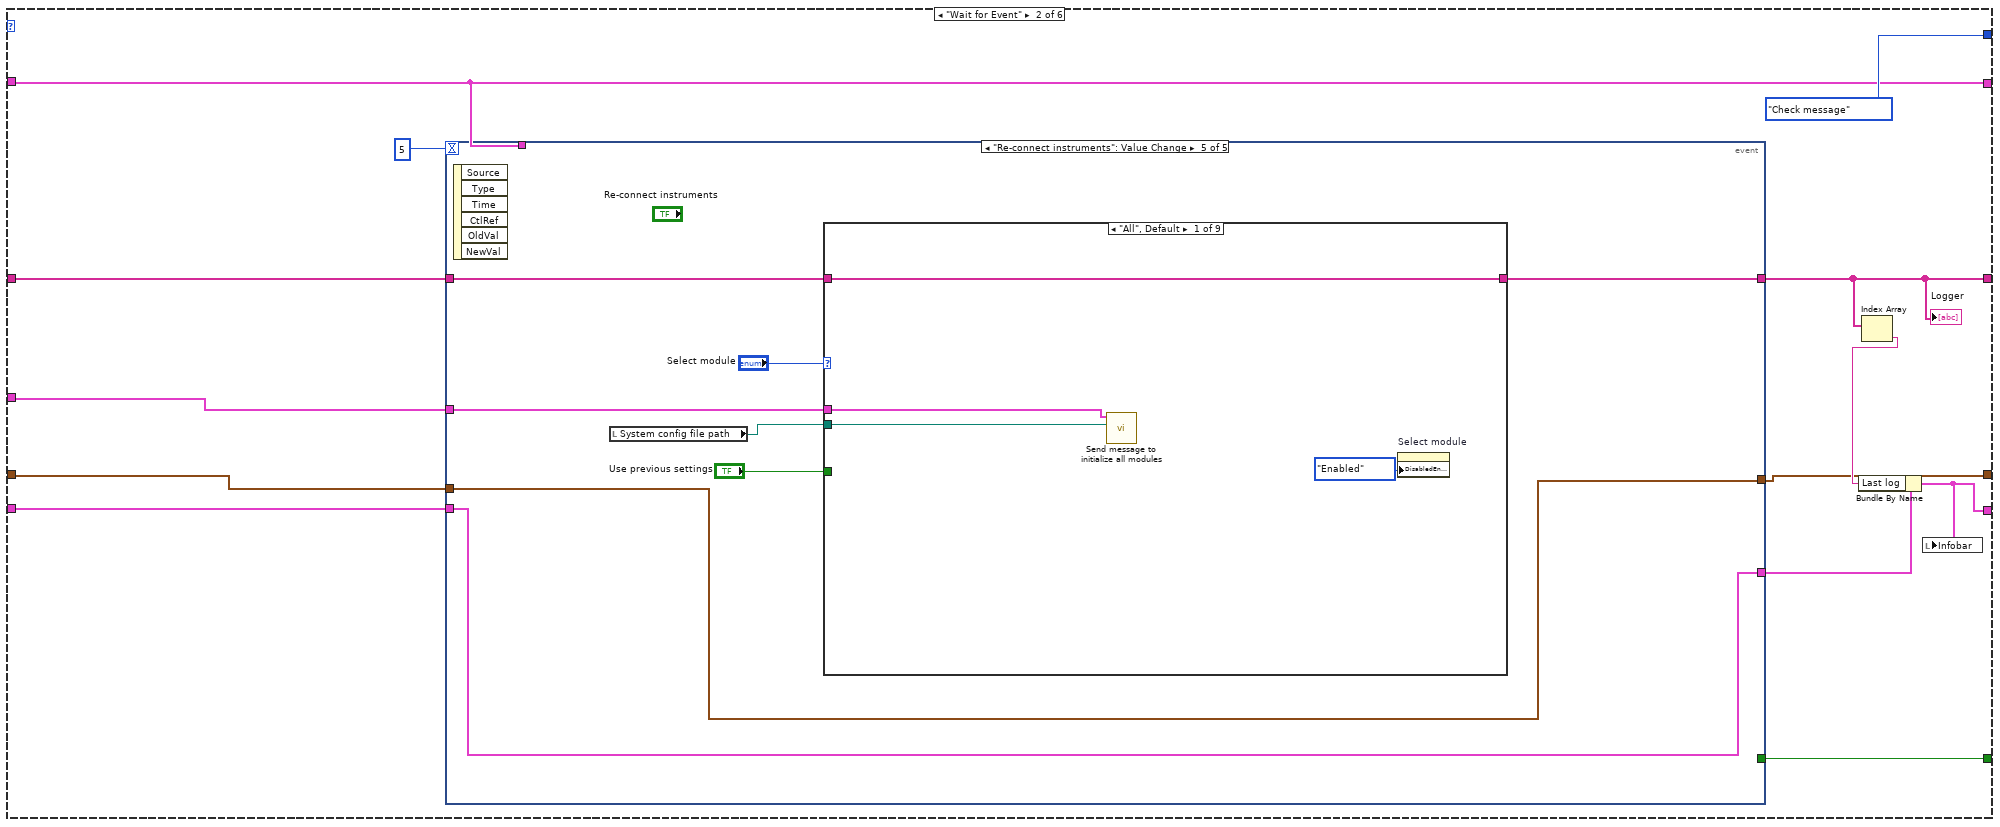
[diagram p6: hidden frame]
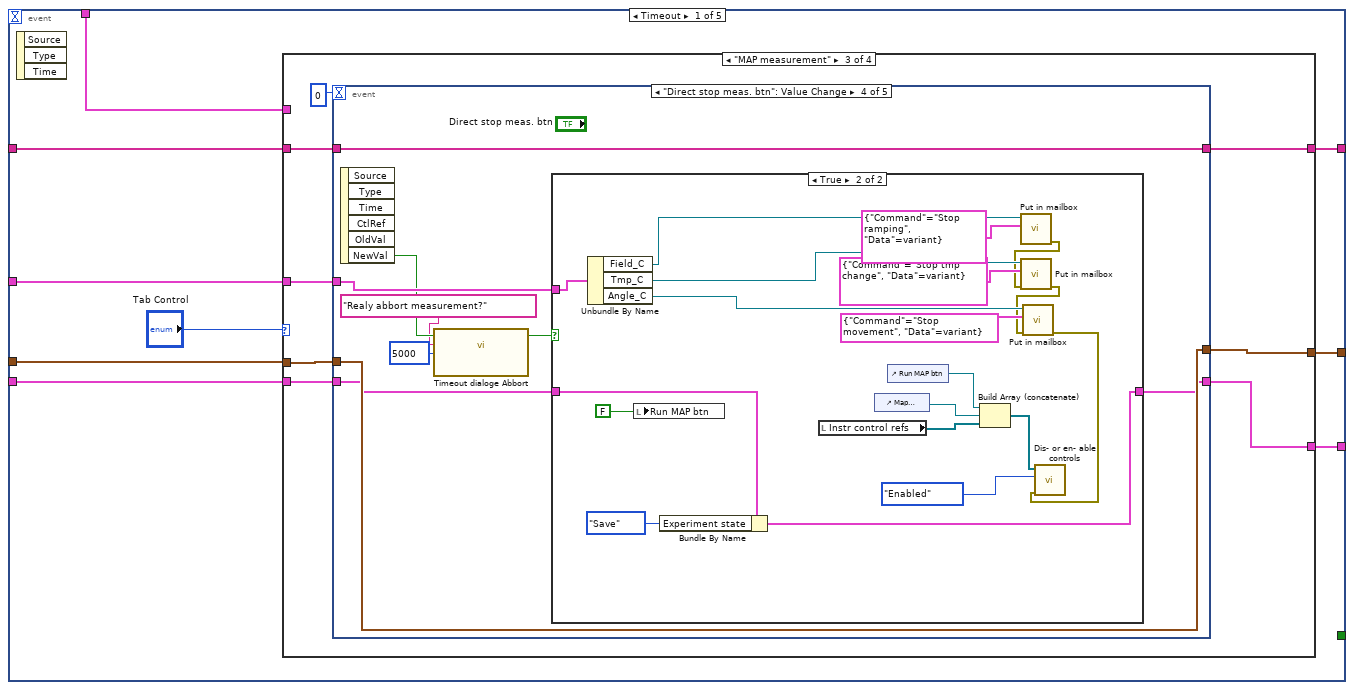
[diagram p7: hidden frame]
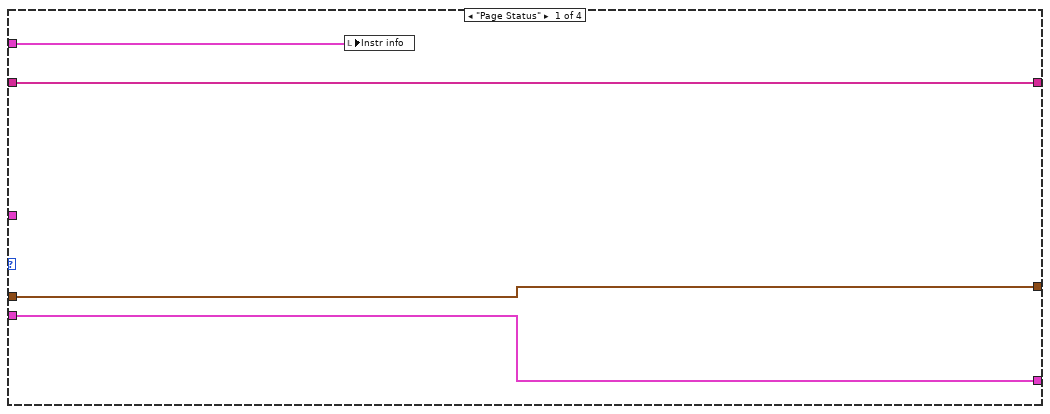
[diagram p8: hidden frame]
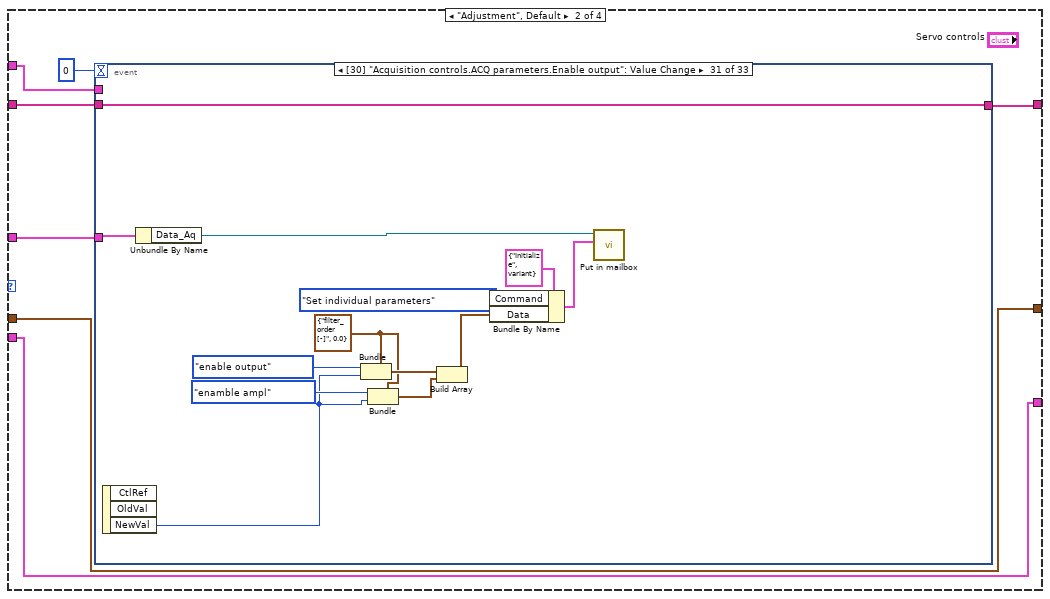
[diagram p9: hidden frame]
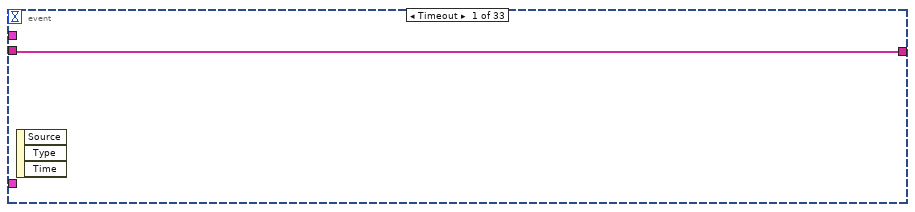
[diagram p10: hidden frame]
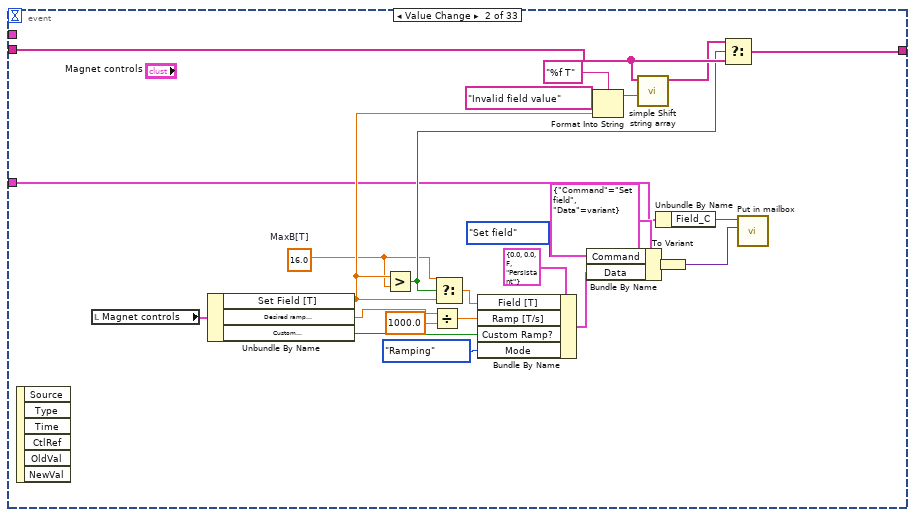
[diagram p11: hidden frame]
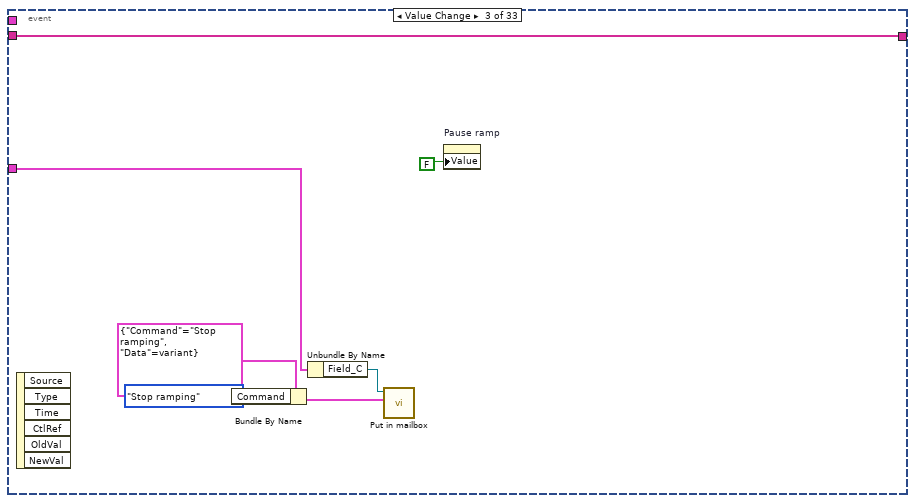
[diagram p12: hidden frame]
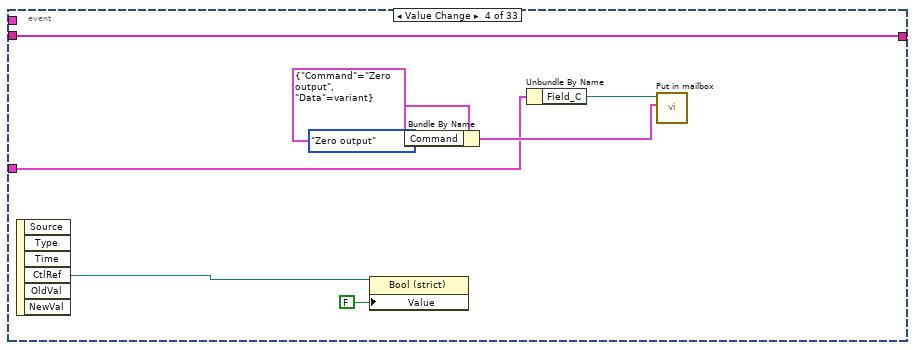
[diagram p13: hidden frame]
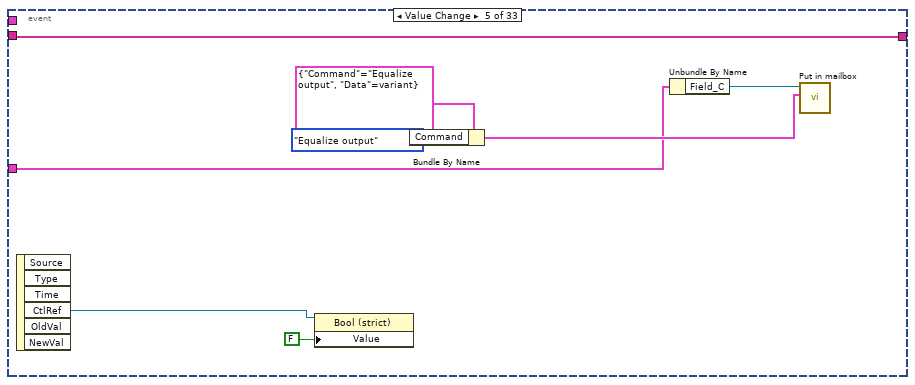
[diagram p14: hidden frame]
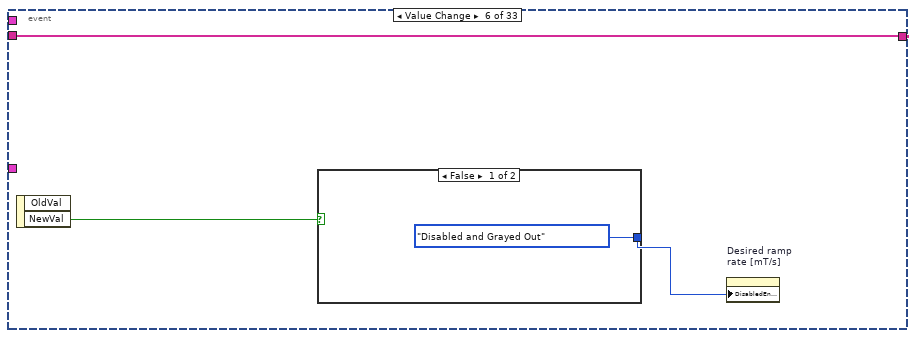
[diagram p15: hidden frame]
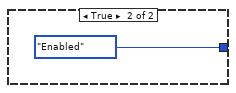
[diagram p16: hidden frame]
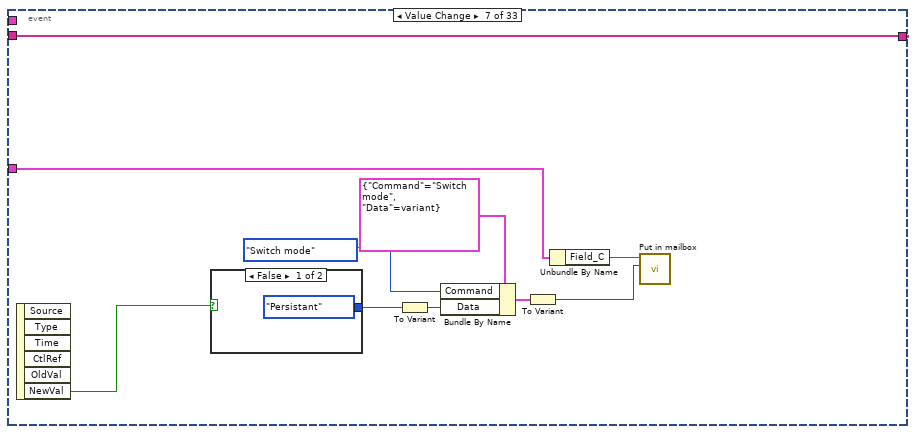
[diagram p17: hidden frame]
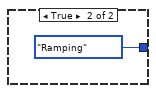
[diagram p18: hidden frame]
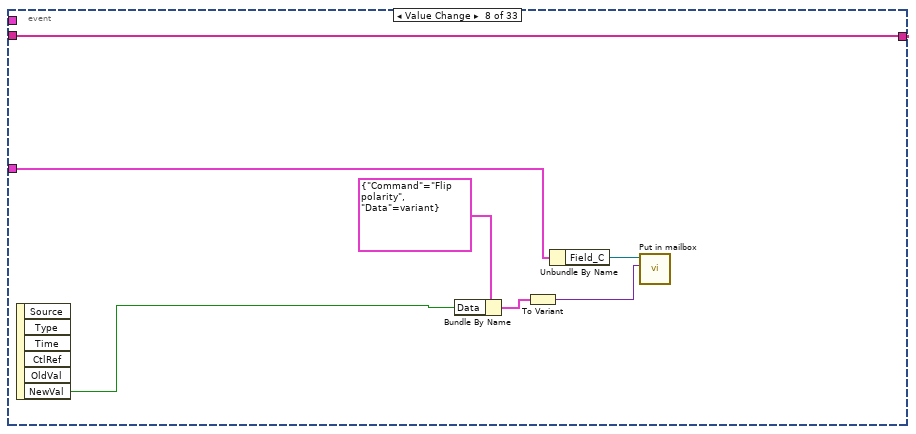
[diagram p19: hidden frame]
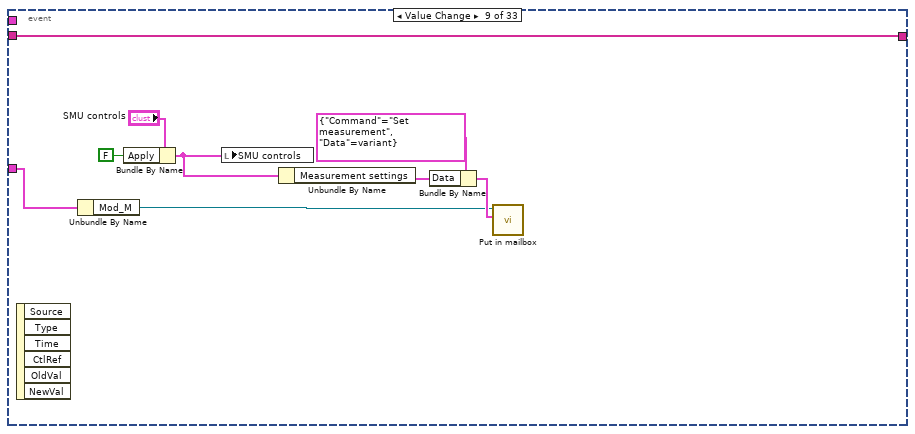
[diagram p20: hidden frame]
diagram:
  w3 = T26 {"Magnet"={"PSU"="None", "T monitor"="None", "Last update"=timestamp(0 s since 1904-01-01), "Field [T]"=0.0, "Ramp [mT/s]"=0.0, "Heater"=FALSE, "Ramp state"=enum."At Target"}, "ACQ"={"Lock-in"="None", "Multimeter"="None", "Last update"=timestamp(0 s since 1904-01-01), "Freq [kHz]"=0.0, "Ampl [mV]"=0.0, "OutEn"=FALSE, "In50 Ohm"=FALSE, "DemEn"=FALSE}, "THz"={"Name"="None", "Description"="None", "Last update"=timestamp(0 s since 1904-01-01), "Start [GHz]"=0.0, "Im Freq[MHz]"=0.0, "End [GHz]"=0.0}, "VTI"={"TC"="None", "Last update"=timestamp(0 s since 1904-01-01), "VTI [K]"=0.0, "Sample [K]"=0.0, "Trap[K]"=0.0, "HePot [K]"=0.0, "Ambient [K]"=0.0}, "Rot"={"Name"=3, "Last update"=timestamp(0 s since 1904-01-01), "Actuator"=1, "Connected"=FALSE, "Moving"=FALSE, "Target"=FALSE, "Cap [nF]"=0.0, "Position [°]"=0.0}, "Servo"=[{"Name"=enum."Unknown", "Last update"=timestamp(0 s since 1904-01-01), "Position"=0.0, "Pos limit"=0.0, "Neg limit"=0.0, "Power"=FALSE}], "SMU"={"Name"="", "Last update"=timestamp(0 s since 1904-01-01), "Source F"="", "Source V"=0.0, "Measure F"="", "Measure V"=0.0, "Output"=FALSE}, "PMD"={"Name"="", "Last update"=timestamp(0 s since 1904-01-01), "Position [°]"=0.0, "Speed"=0.0, "Desired [°]"=0.0, "Moving"=FALSE, "reserved"=0.0}, "PwrM"={"Name"="", "Last update"=timestamp(0 s since 1904-01-01), "Outage?"=FALSE, "Low"=FALSE, "No battery"=FALSE, "Battery [%]"=0, "Charging"=FALSE}}  # Instr info
  w4 = T24 {"Remains"=0.0, "T_sample [K]"=1.6, "Last log"="", "Experiment state"=enum."Setup", "Field [T]"=0.0, "Sample holder"=enum."Simple", "Started"=timestamp(0 s since 1904-01-01)}  # Infobar
  # "8 947,848533 sec"
  # "1,8310546875 kS/s"
  # "3,662109375 ks/s"
  # "4,473924266 sec"
  # "2,2369621333 second"
  # "7,32421875 kS/s"
  # "1,118481066 second for sweep"
  # "16384 samples"
  # "14,6484375 kS/s"
  # "All modules requiere"
  n1 = call "Initialize Messenger.vi"() -> ("Referencies out"=w10:T29)  [unwired: 2 in, 1 out]
  n2 = Initialize Array("", 40 ("dimension size")) -> (w7:string[])
  n3 = while {
    tunnel: w10 -> [w25]
    shift-right: [w14] -> _
    shift-left: w7 -> [w24]
    shift-right: [w22] -> w5
    shift-left: TopStates."Initialize GUI" ("State") -> [w23]
    shift-right: [w20] -> _
    shift-left: _ -> [w19]
    shift-right: [w11] -> _
    shift-left: T22 {"B_start[T]"=0.0, "B_End[T]"=0.2, "B_rate [mT/s]"=1.0, "F_start[GHz]"=295.0, "F_end[GHz]"=0.0, "Sampling rate"=1, "Tmp [K]"=295.0, "Wait[min]"=0.0, "Points"=0, "Display signal"=enum."Phi", "Signal treat"=enum."None", "Sweep [s]"=2.0} ("Map parameters") -> [w17]
    shift-right: [w15] -> _
    shift-left: w4 -> [w16]
    shift-right: [w12] -> _
    shift-left: w3 -> [w13]
    stop <- w21 stop-if-true
    # "new log"
    # "State Machine While Loop"
    n4 = case shown="\"Check measurement\"" w23 {
      tunnel: w25 -> [_ w118 w1173 w2222 _ _]
      tunnel: w24 -> [w84 w117 w1187 w2221 w2486 _]
      tunnel: [w83 w106 w1186 w2220 w2485 w2491] -> w14
      tunnel: [TopStates."Wait for Event" ("State") TopStates."Check message" ("State") w1176 TopStates."Wait for Event" ("State") TopStates."Stop" ("State") TopStates."Initialize GUI" ("State")] -> w22
      tunnel: [_ w115 _ _ _ _] -> w21
      tunnel: [w72 w107 w1174 w2217 w2483 w2490] -> w11
      tunnel: w17 -> [w72 w113 w1174 w2218 w2483 w2490]
      tunnel: [w70 w108 w1175 w2219 w2482 w2489] -> w15
      tunnel: w16 -> [w71 w112 w1170 w2214 w2482 w2489]
      tunnel: w13 -> [w62 w109 w1172 w2215 w2481 w2488]
      tunnel: [w62 w109 w1171 w2215 w2481 w2488] -> w12
      frame "Initialize GUI", Default {
        w32 = 1.118481 items=["1,1s"=1.118481, "2,2s"=2.236962, "4,5s"=4.473924, "9s"=8.947848] ("Line rate")
        n5 = local read "Use previous settings"() -> (w56:bool)
        n6 = property on="Instr control refs" class="Arr (strict)"("Visible"=TRUE) -> ()  [unwired: 2 in, 2 out]
        n7 = local write "Select module"(T31."All" ("Module")) -> ()
        n8 = local read "Sample holder"() -> (w55:T13)
        n9 = local write "Tab Control"(T6."Page Status" ("Tab Control")) -> ()
        n10 = case shown="True" w56 {
          tunnel: [w91 w93] -> w59
          tunnel: [T14 {"Filter order"=7.0, "Filter tau [ms]"=50.0, "F_Mod [kHz]"=1.0, "Amp_Mod [mV]"=1.0, "Enable output"=0, "Phase [°]"=0.0} ("ACQ parameters") w96] -> w54
          frame False {
            w91 = T16 {"AMC"=9, "Multip"=1, "Base frequency [GHz]"=90.0, "End frequency [GHz]"=90.0, "Im frequency [MHz]"=10.0, "Sweep up [ms]"=0.0, "Reset trigger?"=FALSE}  # VDI control
          }
          frame True {
            n11 = local read "VID control"() -> (w95:T16)
            n12 = property on="ACQ parameters" class="Clust (strict)"() -> ("Value"=w94:T14)  [unwired: 2 in, 2 out]
            n13 = call "Open config file.vi"("MAG config file path"="System config file path") -> ("error out"=w104:errorcluster, "Refnum out"=w105:T76)  [unwired: 7 in, 2 out]
            n14 = call <userlib>:"Read Section Cluster__ogtk.vi"("error in (no error)"=w104, "Section Formatted Cluster Type"=w94, "refnum"=w105) -> ("Section Formatted Cluster"=w103:variant, "dup refnum"=w100:T76)  [unwired: 4 in, 3 out]
            n15 = Variant To Data(type=w94, Variant=w103) -> (data=w96:T14)  [unwired: 1 in, 1 out]
            n16 = call <userlib>:"Read Section Cluster__ogtk.vi"("Section Formatted Cluster Type"=w95, "refnum"=w100) -> ("error out"=w102:errorcluster, "Section Formatted Cluster"=w101:variant, "dup refnum"=w99:T76)  [unwired: 5 in, 2 out]
            n17 = Variant To Data(error in=w102, type=w95, Variant=w101) -> (data=w93:T16, error out=w97:errorcluster)
            n18 = call <vilib>:"Close Config Data.vi"("error in (no error)"=w97, "refnum"=w99) -> ("file path"=w92:path)  [unwired: 8 in, 1 out]
            n19 = local write "System config file path"(w92) -> ()
          }
        }
        n20 = control-ref of="Run MAP btn"() -> (w53:refnum<vi>)
        n21 = control-ref of="Direct stop meas. btn"() -> (w42:refnum<vi>)
        n22 = control-ref of="Acquisition controls"() -> (w74:refnum<vi>)
        n23 = control-ref of="VID control"() -> (w57:refnum<vi>)
        n24 = control-ref of="VTI control"() -> (w58:refnum<vi>)
        n25 = control-ref of="Servo controls"() -> (w63:refnum<vi>)
        n26 = control-ref of="Magnet controls"() -> (w73:refnum<vi>)
        n27 = Bundle By Name(cluster=w71, "Sample holder"=w55, "Experiment state"=experiment_state."Setup" ("Value")) -> (w70:T24)
        n28 = Build Array(w74, w57, w58, w63, w73) -> (w64:refnum<vi>[])
        "Instr control refs" <- w64
        n29 = Build Array (concatenate)(w64, w53) -> (w38:refnum<vi>[])
        n30 = property class="Clust"(reference=w63) -> ("Top"=w67:i32)  [unwired: 1 in, 2 out]
        n31 = control-ref of="QO table"() -> (w66:refnum<vi>)
        n32 = call <vilib>:"Is Path and Not Empty.vi"("path"="Folder path") -> ("Is Path and Not Empty?"=w37:bool)  [unwired: 4 in]
        n33 = call "Dis- or en- able controls.vi"("Disabled"=T32."Disabled and Grayed Out", "Control referencies"=w38) -> ()  [unwired: 9 in, 1 out]
        n34 = case shown="False" w37 {
          frame False {
            w87 = T77 2 items=["User Home"=0, "User Desktop"=1, "User Documents"=2, "User Application Data"=3, "User Preferences"=4, "User Temporary"=5, "Public Documents"=6, "Public Application Data"=7, "Public Preferences"=8, "Public Cache"=13, "System Core Libraries"=9, "System Installed Libraries"=10, "Application Files"=11, "Boot Volume Root"=12] ("system directory type")
            n35 = call <vilib>:"Get System Directory.vi"("system directory type"=w87) -> ("system directory"=w89:path)  [unwired: 10 in]
            n36 = Build Path(base path=w89, name or relative path="Measurements") -> (appended path=w88:path)
            n37 = local write "Folder path"(w88) -> ()
          }
          frame True {
          }
        }
        n38 = Add(x=w67, y=260 ("Position:Top")) -> (x+y=w68:i32)
        n39 = property class="Clust (strict)"(reference=w66, "Top"=w68) -> ()  [unwired: 1 in, 2 out]
        n40 = local write "VID control"(w59) -> ()
        n41 = property on="ACQ parameters" class="Clust (strict)"("Value"=w54) -> ()  [unwired: 2 in, 2 out]
        n42 = control-ref of="Open measurement"() -> (w39:refnum<vi>)
        n43 = Build Array (concatenate)(w39, w38) -> (w40:refnum<vi>[])
        n44 = Build Array(w42) -> (w41:refnum<vi>[])
        n45 = Bundle By Name(cluster=T2 {"To disable"=[], "To enable"=[]} ("Controls referencies"), "To disable"=w40, "To enable"=w41) -> (→"Controls referencies":T2)
        n46 = Initialize Array(T4 {"Field [T]"=[], "Intensity"=[], "Start F [GHz]"=0.0, "End F[GHz]"=0.0, "BStart[T]"=0.0, "Bend[T]"=0.0, "Bsize"=0} ("Cluster 2"), 3 ("dimension size")) -> (→"Review results":T4[])
        n47 = local write "Line rate"(w32) -> ()
        n48 = Initialize Array("Empty", 3 ("dimension size")) -> (w46:string[])
        n49 = property on="Data file to show" class="Ring (strict)"("Strings []"=w46) -> ()  [unwired: 2 in, 2 out]
        n50 = call "Create new Log files.vi"("Log folder"="Log folder") -> ("error out"=w27:errorcluster, "dup path"=w30:path, "tmp logfile out"=→"Temperature log ref":refnum<file>, "event logfile out"=w28:refnum<file>)  [unwired: 7 in]
        n51 = call "Intensity Color Tables.vi"("Map Selector"=T30."original") -> ("Color Map Array"=w35:u32[])  [unwired: 10 in]
        n52 = Initialize Array("", 3 ("dimension size")) -> (w51:string[])
        n53 = property on="EPR map" class="IntGraph (strict)"("Color Table"=w35) -> ()  [unwired: 2 in, 2 out]
        n54 = call "Add actual date time to string.vi"("String in"="GUI initialized") -> ("String out"=w79:string)  [unwired: 4 in]
        n55 = local write "Log folder"(w30) -> ()
        n56 = local write "Review Header"(w51) -> ()
        n57 = Concatenate Strings(w79, "\r\n") -> (w78:string)
        n58 = call "simple Shift string array.vi"("Element in"=w79, "Array in"=w84) -> ("Array out"=w83:string[])  [unwired: 8 in, 1 out]
        n59 = Write to Text File(file (use dialog)=w28, text=w78, error in=w27) -> (refnum out=→"loggersRef":refnum<file>)  [unwired: 1 in, 2 out]
        "Instr status" <- T1 {"Mag"=FALSE, "Rot"=FALSE, "VTI"=FALSE, "MFLI"=FALSE, "Serv"=FALSE, "THz"=FALSE, "ADQ7"=FALSE, "SMU"=FALSE, "PMD"=FALSE, "UPS"=FALSE, "DMM"=FALSE, "abc"=FALSE} ("Instruments status 2")
        "Infobar" <- T24 {"Remains"=0.0, "T_sample [K]"=0.0, "Last log"="", "Experiment state"=enum."Setup", "Field [T]"=0.0, "Sample holder"=enum."Simple", "Started"=timestamp(0 s since 1904-01-01)} ("Infobar")
      }
      frame "Wait for Event" {
        n60 = event shown="[4] \"Re-connect instruments\": Value Change" {
          selector: _ -> [_ _ _ _ _]
          dyn-events: _ -> [_ _ _ _ _]
          timeout: 5 -> [_ _ _ _ _]
          tunnel: w117 -> [w126 w911 w921 w989 w1073]
          tunnel: [w127 w911 w921 w989 w1072] -> w106
          tunnel: w118 -> [w121 _ w915 w991 w1074]
          tunnel: [_ _ _ w990 _] -> w115
          tunnel: [w125 w914 w920 w988 w1071] -> w107
          tunnel: w113 -> [w124 w914 w920 w988 w1071]
          tunnel: [w123 w913 w919 w987 w1070] -> w110
          tunnel: w112 -> [w122 w913 w919 w987 w1070]
          tunnel: w109 -> [w120 _ _ _ _]
          event Timeout {
            n61 = event-data() -> ()  [unwired: 1 in, 3 out]
            n62 = case shown="\"MAP measurement\"" "Tab Control" {
              tunnel: [w131 w138 w782 w856] -> w127
              tunnel: w126 -> [w131 w136 w783 w856]
              tunnel: w121 -> [_ w135 w780 _]
              tunnel: [w130 w134 w779 w855] -> w125
              tunnel: w124 -> [w130 w134 w778 w855]
              tunnel: [w129 w133 w776 w854] -> w123
              tunnel: w122 -> [w129 w133 w777 w854]
              tunnel: w120 -> [w128 w132 _ _]
              frame "Page Status" {
                n63 = local write "Instr info"(w128) -> ()
              }
              frame "Adjustment", Default {
                n64 = event shown="[30] \"Acquisition controls.ACQ parameters.Enable output\": Value Change" {
                  selector: _ -> [_ _ _ _ _ _ _ _ _ _ _ _ _ _ _ _ _ _ _ _ _ _ _ _ _ _ _ _ _ _ _ _ _]
                  dyn-events: _ -> [_ _ _ _ _ _ _ _ _ _ _ _ _ _ _ _ _ _ _ _ _ _ _ _ _ _ _ _ _ _ _ _ _]
                  timeout: 0 -> [_ _ _ _ _ _ _ _ _ _ _ _ _ _ _ _ _ _ _ _ _ _ _ _ _ _ _ _ _ _ _ _ _]
                  tunnel: w136 -> [w139 w155 w170 w178 w186 w187 w196 w208 w219 w225 w231 w234 w278 w288 w317 w331 w356 w382 w412 w447 w492 w521 w546 w572 w597 w623 w648 w682 w691 w707 w756 w767 w773]
                  tunnel: [w139 w159 w170 w178 w186 w187 w196 w208 w219 w225 w231 w234 w278 w288 w317 w331 w356 w382 w412 w447 w492 w521 w546 w572 w597 w623 w648 w682 w691 w707 w756 w767 w773] -> w138
                  tunnel: w135 -> [_ w145 w164 w173 w181 _ w192 w205 w211 w220 w228 _ w268 w285 w314 w322 w347 w373 w398 w423 w467 w512 w537 w563 w588 w614 w639 w673 _ w706 w755 w766 _]
                  tunnel: w132 -> [_ _ _ _ _ _ _ _ _ _ _ w233 w255 w280 _ w319 w343 w369 w394 w420 w463 w509 w533 w559 w584 w610 w635 _ _ _ _ _ _]
                  event Timeout {
                    (unwired) TopStates."Check message" ("State")
                    n65 = event-data() -> ()  [unwired: 1 in, 3 out]
                  }
                  event Value Change {
                    w140 = 16.0  # MaxB[T]
                    n66 = event-data() -> ()  [unwired: 1 in, 6 out]
                    n67 = local read "Magnet controls"() -> (w161:T18)
                    n68 = Unbundle By Name(w161) -> ("Set Field [T]"=w152:dbl, "Desired ramp\nrate [mT/s]"=w142:dbl, "Custom\nramp"=w148:bool)
                    n69 = Greater?(x=w152, y=w140) -> (0:w153:bool)
                    n70 = Divide(x=w142, y=1000.0) -> (x/y=w143:dbl)
                    n71 = Select(t=w140, s=w153, f=w152) -> (s? t:f=w150:dbl)
                    n72 = Bundle By Name(cluster=T34 {"Field [T]"=0.0, "Ramp [T/s]"=0.0, "Custom Ramp?"=FALSE, "Mode"=enum."Persistant"} ("Set Field"), "Field [T]"=w150, "Ramp [T/s]"=w143, "Custom Ramp?"=w148, "Mode"=Magnet_mode_public."Ramping") -> (w149:T34)
                    n73 = Bundle By Name(cluster=T36 {"Command"=enum."Set field", "Data"=variant(enum16{"Ramping", "Perzistant"} enum."Ramping")} ("MSG to magnet"), "Command"=Magnet_Orders."Set field" ("Order"), "Data"=w149) -> (w163:T36)
                    n74 = Format Into String(format string="%f T", initial string="Invalid field value" ("Element in"), w152) -> (resulting string=w156:string)  [unwired: 1 in, 1 out]
                    n75 = call "simple Shift string array.vi"("Element in"=w156, "Array in"=w155) -> ("Array out"=w154:string[])  [unwired: 8 in, 1 out]
                    n76 = Unbundle By Name(w145) -> ("Field_C"=w147:refnum<queue>)
                    n77 = To Variant(anything=w163) -> (Variant=w146:variant)
                    n78 = Select(t=w154, s=w153, f=w155) -> (s? t:f=w159:string[])
                    n79 = call "Put in mailbox.vi"("Message"=w146, "Queue in"=w147) -> ()  [unwired: 7 in, 3 out]
                  }
                  event Value Change {
                    n80 = event-data() -> ()  [unwired: 1 in, 6 out]
                    n81 = Bundle By Name(cluster=T36 {"Command"=enum."Stop ramping", "Data"=variant(enum16{"Ramping", "Perzistant"} enum."Ramping")} ("MSG to magnet"), "Command"=Magnet_Orders."Stop ramping" ("Order")) -> (w167:T36)
                    n82 = Unbundle By Name(w164) -> ("Field_C"=w168:refnum<queue>)
                    n83 = call "Put in mailbox.vi"("Message"=w167, "Queue in"=w168) -> ()  [unwired: 7 in, 3 out]
                    n84 = property on="Pause ramp" class="Bool (strict)"("Value"=FALSE) -> ()  [unwired: 2 in, 2 out]
                  }
                  event Value Change {
                    n85 = event-data() -> ("CtlRef"=w172:refnum<vi>)  [unwired: 1 in, 5 out]
                    n86 = property class="Bool (strict)"(reference=w172, "Value"=FALSE) -> ()  [unwired: 1 in, 2 out]
                    n87 = Bundle By Name(cluster=T36 {"Command"=enum."Zero output", "Data"=variant(enum16{"Ramping", "Perzistant"} enum."Ramping")} ("MSG to magnet"), "Command"=Magnet_Orders."Zero output" ("Order")) -> (w174:T36)
                    n88 = Unbundle By Name(w173) -> ("Field_C"=w175:refnum<queue>)
                    n89 = call "Put in mailbox.vi"("Message"=w174, "Queue in"=w175) -> ()  [unwired: 7 in, 3 out]
                  }
                  event Value Change {
                    n90 = event-data() -> ("CtlRef"=w179:refnum<vi>)  [unwired: 1 in, 5 out]
                    n91 = property class="Bool (strict)"(reference=w179, "Value"=FALSE) -> ()  [unwired: 1 in, 2 out]
                    n92 = Bundle By Name(cluster=T36 {"Command"=enum."Equalize output", "Data"=variant(enum16{"Ramping", "Perzistant"} enum."Ramping")} ("MSG to magnet"), "Command"=Magnet_Orders."Equalize output" ("Order")) -> (w182:T36)
                    n93 = Unbundle By Name(w181) -> ("Field_C"=w183:refnum<queue>)
                    n94 = call "Put in mailbox.vi"("Message"=w182, "Queue in"=w183) -> ()  [unwired: 7 in, 3 out]
                  }
                  event Value Change {
                    n95 = event-data() -> ("NewVal"=w189:bool)  [unwired: 1 in, 1 out]
                    n96 = case shown="False" w189 {
                      tunnel: [T32."Disabled and Grayed Out" ("Disabled") T32."Enabled" ("Disabled")] -> w188
                      frame False {
                      }
                      frame True {
                      }
                    }
                    n97 = property on="Desired ramp\nrate [mT/s]" class="DigNum (strict)"("DisabledEnum"=w188) -> ()  [unwired: 2 in, 2 out]
                  }
                  event Value Change {
                    n98 = event-data() -> ("NewVal"=w197:bool)  [unwired: 1 in, 5 out]
                    n99 = case shown="False" w197 {
                      tunnel: [Magnet_mode_public."Persistant" ("Operation mode") Magnet_mode_public."Ramping" ("Operation mode")] -> w198
                      frame False {
                      }
                      frame True {
                      }
                    }
                    n100 = To Variant(anything=w198) -> (Variant=w195:variant)
                    n101 = Bundle By Name(cluster=T36 {"Command"=enum."Switch mode", "Data"=variant(enum16{"Ramping", "Perzistant"} enum."Ramping")} ("MSG to magnet"), "Command"=Magnet_Orders."Switch mode" ("Order"), "Data"=w195) -> (w201:T36)
                    n102 = To Variant(anything=w201) -> (Variant=w193:variant)
                    n103 = Unbundle By Name(w192) -> ("Field_C"=w194:refnum<queue>)
                    n104 = call "Put in mailbox.vi"("Message"=w193, "Queue in"=w194) -> ()  [unwired: 7 in, 3 out]
                  }
                  event Value Change {
                    n105 = event-data() -> ("NewVal"=w204:bool)  [unwired: 1 in, 5 out]
                    n106 = Bundle By Name(cluster=T36 {"Command"=enum."Flip polarity", "Data"=variant(enum16{"Ramping", "Perzistant"} enum."Ramping")} ("MSG to magnet"), "Data"=w204) -> (w210:T36)
                    n107 = To Variant(anything=w210) -> (Variant=w206:variant)
                    n108 = Unbundle By Name(w205) -> ("Field_C"=w207:refnum<queue>)
                    n109 = call "Put in mailbox.vi"("Message"=w206, "Queue in"=w207) -> ()  [unwired: 7 in, 3 out]
                  }
                  event "SMU controls.Apply": Value Change {
                    n110 = event-data() -> ()  [unwired: 1 in, 6 out]
                    n111 = Unbundle By Name(w211) -> ("Mod_M"=w215:refnum<queue>)
                    n112 = Bundle By Name(cluster="SMU controls", "Apply"=FALSE) -> (w212:T20)
                    n113 = local write "SMU controls"(w212) -> ()
                    n114 = Unbundle By Name(w212) -> ("Measurement settings"=w218:T19)
                    n115 = Bundle By Name(cluster=T37 {"Command"=enum."Set measurement", "Data"=variant} ("MSG to Source meter"), "Data"=w218) -> (w217:T37)
                    n116 = call "Put in mailbox.vi"("Message"=w217, "Queue in"=w215) -> ()  [unwired: 7 in, 3 out]
                  }
                  event "SMU controls.Stop": Value Change {
                    n117 = event-data() -> ("CtlRef"=w224:refnum<vi>)  [unwired: 1 in, 5 out]
                    n118 = Unbundle By Name(w220) -> ("Mod_M"=w221:refnum<queue>)
                    n119 = property class="Bool (strict)"(reference=w224, "Value"=FALSE) -> ()  [unwired: 1 in, 2 out]
                    n120 = call "Put in mailbox.vi"("Message"=T37 {"Command"=enum."Stop measurement", "Data"=variant} ("MSG to Source meter"), "Queue in"=w221) -> ()  [unwired: 7 in, 3 out]
                  }
                  event "SMU controls.Record": Value Change {
                    n121 = event-data() -> ("CtlRef"=w227:refnum<vi>)  [unwired: 1 in, 5 out]
                    n122 = property class="Bool (strict)"(reference=w227, "Value"=FALSE) -> ()  [unwired: 1 in, 2 out]
                    n123 = Unbundle By Name(w228) -> ("Mod_M"=w229:refnum<queue>)
                    n124 = call "Put in mailbox.vi"("Message"=T37 {"Command"=enum."Start measurement", "Data"=variant} ("MSG to Source meter"), "Queue in"=w229) -> ()  [unwired: 7 in, 3 out]
                  }
                  event Value Change {
                    # "top+260"
                    # "top+130"
                    n125 = event-data() -> ("NewVal"=w245:dbl)  [unwired: 1 in, 5 out]
                    n126 = Unbundle By Name(w233) -> ("Servo"=w232:T10[])
                    n127 = control-ref of="Servo controls"() -> (w253:refnum<vi>)
                    n128 = property class="Clust"(reference=w253) -> (error out=w244:errorcluster, "Top"=w239:i32)  [unwired: 1 in, 1 out]
                    n129 = call "Extract axis properties.vi"("Name"=Axis_names."AxisX", "All servo status"=w232) -> ("Servo"=w250:T10)  [unwired: 6 in, 2 out]
                    n130 = Unbundle By Name(w250) -> ("Pos limit"=w248:dbl, "Neg limit"=w247:dbl)
                    n131 = control-ref of="QO table"() -> (w249:refnum<vi>)
                    n132 = Add(x=w239, y=130) -> (x+y=w241:i32)
                    n133 = Add(x=w239, y=260) -> (x+y=w238:i32)
                    n134 = Subtract(x=w248, y=w247) -> (x-y=w235:dbl)
                    n135 = Divide(x=130.0 ("y"), y=w235) -> (x/y=w246:dbl)
                    n136 = Multiply(x=w245, y=w246) -> (x*y=w242:dbl)
                    n137 = Subtract(x=w238, y=w242) -> (x-y=w237:dbl)
                    n138 = In Range and Coerce(upper limit=w238, x=w237, lower limit=w241) -> (coerced(x)=w252:dbl)  [unwired: 1 out]
                    n139 = property class="Clust (strict)"(reference=w249, error in=w244, "Top"=w252) -> ()  [unwired: 2 out]
                  }
                  event Value Change {
                    w260 = 300.0 ("x")
                    n140 = event-data() -> ("CtlRef"=w277:refnum<vi>)  [unwired: 1 in, 5 out]
                    n141 = Unbundle By Name(w255) -> ("Servo"=w254:T10[])
                    n142 = property class="Bool (strict)"(reference=w277, "Value"=FALSE) -> ()  [unwired: 1 in, 2 out]
                    n143 = call "Extract axis properties.vi"("Name"=Axis_names."AxisX", "All servo status"=w254) -> ("Servo"=w275:T10, "Index"=w266:i32)  [unwired: 6 in, 1 out]
                    n144 = Unbundle By Name(w275) -> ("Pos limit"=w262:dbl, "Neg limit"=w261:dbl, "Position"=w263:dbl)
                    n145 = Subtract(x=w260, y=w263) -> (x-y=w257:dbl)
                    n146 = In Range and Coerce(upper limit=w262, x=w260, lower limit=w261) -> (In Range?=w259:bool)  [unwired: 1 out]
                    n147 = Select(t=w257, s=w259, f=0.0) -> (s? t:f=w256:dbl)
                    n148 = Initialize Array(0.0 ("element"), 5 ("dimension size")) -> (w264:dbl[])
                    n149 = Replace Array Subset(array=w264, new element=w256, index=w266) -> (w265:dbl[])
                    n150 = Bundle By Name(cluster=T40 {"Command"=enum."Move by", "Data"=variant(dbl[] [])} ("MSG to Servo"), "Command"=Servo_commands."Move by", "Data"=w265) -> (w267:T40)
                    n151 = Unbundle By Name(w268) -> ("Table_C"=w269:refnum<queue>)
                    n152 = call "Put in mailbox.vi"("Message"=w267, "Queue in"=w269) -> ()  [unwired: 7 in, 3 out]
                  }
                  event Value Change {
                    n153 = event-data() -> ("CtlRef"=w287:refnum<vi>, "NewVal"=w284:bool)  [unwired: 1 in, 4 out]
                    n154 = Unbundle By Name(w280) -> ("Servo"=w279:T10[])
                    n155 = property class="Bool (strict)"(reference=w287, "Value"=FALSE) -> ()  [unwired: 1 in, 2 out]
                    n156 = call "Timeout dialoge Abbort.vi"("Enable"=w284, "Message to Display"="Really go to measurement position?", "timeout[ms]"=u32 3000) -> ("Yes"=w281:bool)  [unwired: 15 in, 1 out]
                    n157 = case shown="True" w281 {
                      tunnel: w285 -> [_ w302]
                      tunnel: w279 -> [_ w289]
                      frame False {
                      }
                      frame True {
                        (unwired) 890.58 ("x")
                        w294 = 895.866 ("x")
                        n158 = call "Extract axis properties.vi"("Name"=Axis_names."AxisX", "All servo status"=w289) -> ("Servo"=w309:T10, "Index"=w300:i32)  [unwired: 6 in, 1 out]
                        n159 = Unbundle By Name(w309) -> ("Pos limit"=w296:dbl, "Neg limit"=w295:dbl, "Position"=w297:dbl)
                        n160 = Subtract(x=w294, y=w297) -> (x-y=w291:dbl)
                        n161 = In Range and Coerce(upper limit=w296, x=w294, lower limit=w295) -> (In Range?=w293:bool)  [unwired: 1 out]
                        n162 = Unbundle By Name(w302) -> ("Table_C"=w303:refnum<queue>)
                        n163 = Select(t=w291, s=w293, f=0.0) -> (s? t:f=w290:dbl)
                        n164 = Initialize Array(0.0 ("element"), 5 ("dimension size")) -> (w298:dbl[])
                        n165 = Replace Array Subset(array=w298, new element=w290, index=w300) -> (w299:dbl[])
                        n166 = Bundle By Name(cluster=T40 {"Command"=enum."Move by", "Data"=variant(dbl[] [])} ("MSG to Servo"), "Command"=Servo_commands."Move by", "Data"=w299) -> (w301:T40)
                        n167 = call "Put in mailbox.vi"("Message"=w301, "Queue in"=w303) -> ()  [unwired: 7 in, 3 out]
                      }
                    }
                  }
                  event Value Change {
                    n168 = event-data() -> ("CtlRef"=w316:refnum<vi>)  [unwired: 1 in, 5 out]
                    n169 = property class="Bool"(reference=w316, "Value"=FALSE) -> ()  [unwired: 1 in, 2 out]
                    n170 = Unbundle By Name(w314) -> ("Table_C"=w311:refnum<queue>)
                    n171 = Bundle By Name(cluster=T40 {"Command"=enum."Stop", "Data"=variant(dbl[] [])} ("MSG to Servo"), "Command"=Servo_commands."Stop") -> (w310:T40)
                    n172 = call "Put in mailbox.vi"("Message"=w310, "Queue in"=w311) -> ()  [unwired: 7 in, 3 out]
                  }
                  event Value Change {
                    # "X position limit"
                    n173 = event-data() -> ("CtlRef"=w320:refnum<vi>)  [unwired: 1 in, 5 out]
                    n174 = Unbundle By Name(w319) -> ("Servo"=w318:T10[])
                    n175 = call "Extract axis properties.vi"("Name"=Axis_names."AxisX", "All servo status"=w318) -> ("Servo"=w328:T10, "Index"=w325:i32)  [unwired: 6 in, 1 out]
                    n176 = Unbundle By Name(w328) -> ("Position"=w323:dbl, "Pos limit"=w326:dbl)
                    n177 = property on="Step\n[mm]" class="DigNum (strict)"() -> ("Value"=w324:dbl)  [unwired: 2 in, 2 out]
                    n178 = Subtract(x=w326, y=w324) -> (x-y=w330:dbl)
                    n179 = Less?(x=w323, y=w330) -> (x < y?=w329:bool)
                    n180 = case shown="True" w329 {
                      tunnel: w324 -> [_ w340]
                      tunnel: w325 -> [_ w336]
                      tunnel: w322 -> [_ w333]
                      frame False {
                      }
                      frame True {
                        n181 = Initialize Array(0.0 ("element"), 5 ("dimension size")) -> (w341:dbl[])
                        n182 = Replace Array Subset(array=w341, new element=w340, index=w336) -> (w337:dbl[])
                        n183 = Bundle By Name(cluster=T40 {"Command"=enum."Move by", "Data"=variant(dbl[] [])} ("MSG to Servo"), "Command"=Servo_commands."Move by", "Data"=w337) -> (w334:T40)
                        n184 = Unbundle By Name(w333) -> ("Table_C"=w335:refnum<queue>)
                        n185 = call "Put in mailbox.vi"("Message"=w334, "Queue in"=w335) -> ()  [unwired: 7 in, 3 out]
                      }
                    }
                    n186 = property class="Bool (strict)"(reference=w320, "Value"=FALSE) -> ()  [unwired: 1 in, 2 out]
                  }
                  event Value Change {
                    n187 = event-data() -> ("CtlRef"=w345:refnum<vi>)  [unwired: 1 in, 5 out]
                    n188 = Unbundle By Name(w343) -> ("Servo"=w344:T10[])
                    n189 = call "Extract axis properties.vi"("Name"=Axis_names."AxisX", "All servo status"=w344) -> ("Servo"=w353:T10, "Index"=w350:i32)  [unwired: 6 in, 1 out]
                    n190 = Unbundle By Name(w353) -> ("Position"=w348:dbl, "Neg limit"=w351:dbl)
                    n191 = property class="Bool (strict)"(reference=w345, "Value"=FALSE) -> ()  [unwired: 1 in, 2 out]
                    n192 = property on="Step\n[mm]" class="DigNum (strict)"() -> ("Value"=w349:dbl)  [unwired: 2 in, 2 out]
                    n193 = Add(x=w351, y=w349) -> (x+y=w354:dbl)
                    n194 = Greater?(x=w348, y=w354) -> (0:w355:bool)
                    n195 = case shown="True" w355 {
                      tunnel: w349 -> [_ w365]
                      tunnel: w350 -> [_ w361]
                      tunnel: w347 -> [_ w358]
                      frame False {
                      }
                      frame True {
                        n196 = Negate(x=w365) -> (-x=w367:dbl)
                        n197 = Initialize Array(0.0 ("element"), 5 ("dimension size")) -> (w366:dbl[])
                        n198 = Replace Array Subset(array=w366, new element=w367, index=w361) -> (w362:dbl[])
                        n199 = Unbundle By Name(w358) -> ("Table_C"=w359:refnum<queue>)
                        n200 = Bundle By Name(cluster=T40 {"Command"=enum."Move by", "Data"=variant(dbl[] [])} ("MSG to Servo"), "Command"=Servo_commands."Move by", "Data"=w362) -> (w357:T40)
                        n201 = call "Put in mailbox.vi"("Message"=w357, "Queue in"=w359) -> ()  [unwired: 7 in, 3 out]
                      }
                    }
                  }
                  event Value Change {
                    w379 = 0.5 ("y")
                    n202 = event-data() -> ("CtlRef"=w371:refnum<vi>)  [unwired: 1 in, 5 out]
                    n203 = Unbundle By Name(w369) -> ("Servo"=w370:T10[])
                    n204 = call "Extract axis properties.vi"("Name"=Axis_names."AxisY", "All servo status"=w370) -> ("Servo"=w378:T10, "Index"=w375:i32)  [unwired: 6 in, 1 out]
                    n205 = Unbundle By Name(w378) -> ("Position"=w374:dbl, "Pos limit"=w376:dbl)
                    n206 = Subtract(x=w376, y=w379) -> (x-y=w380:dbl)
                    n207 = Less?(x=w374, y=w380) -> (x < y?=w381:bool)
                    n208 = case shown="True" w381 {
                      tunnel: w379 -> [_ w391]
                      tunnel: w375 -> [_ w387]
                      tunnel: w373 -> [_ w383]
                      frame False {
                      }
                      frame True {
                        n209 = Initialize Array(0.0 ("element"), 5 ("dimension size")) -> (w392:dbl[])
                        n210 = Replace Array Subset(array=w392, new element=w391, index=w387) -> (w388:dbl[])
                        n211 = Bundle By Name(cluster=T40 {"Command"=enum."Move by", "Data"=variant(dbl[] [])} ("MSG to Servo"), "Command"=Servo_commands."Move by", "Data"=w388) -> (w384:T40)
                        n212 = Unbundle By Name(w383) -> ("Table_C"=w385:refnum<queue>)
                        n213 = call "Put in mailbox.vi"("Message"=w384, "Queue in"=w385) -> ()  [unwired: 7 in, 3 out]
                      }
                    }
                    n214 = property class="Bool (strict)"(reference=w371, "Value"=FALSE) -> ()  [unwired: 1 in, 2 out]
                  }
                  event Value Change {
                    w405 = 0.5 ("y")
                    n215 = event-data() -> ("CtlRef"=w396:refnum<vi>)  [unwired: 1 in, 5 out]
                    n216 = Unbundle By Name(w394) -> ("Servo"=w395:T10[])
                    n217 = call "Extract axis properties.vi"("Name"=Axis_names."AxisY", "All servo status"=w395) -> ("Servo"=w403:T10, "Index"=w400:i32)  [unwired: 6 in, 1 out]
                    n218 = Unbundle By Name(w403) -> ("Position"=w399:dbl, "Neg limit"=w402:dbl)
                    n219 = property class="Bool (strict)"(reference=w396, "Value"=FALSE) -> ()  [unwired: 1 in, 2 out]
                    n220 = Add(x=w402, y=w405) -> (x+y=w404:dbl)
                    n221 = Negate(x=w405) -> (-x=w406:dbl)
                    n222 = Initialize Array(0.0 ("element"), 5 ("dimension size")) -> (w410:dbl[])
                    n223 = Greater?(x=w399, y=w404) -> (0:w411:bool)
                    n224 = Replace Array Subset(array=w410, new element=w406, index=w400) -> (w407:dbl[])
                    n225 = case shown="True" w411 {
                      tunnel: w407 -> [_ w417]
                      tunnel: w398 -> [_ w414]
                      frame False {
                      }
                      frame True {
                        n226 = Unbundle By Name(w414) -> ("Table_C"=w415:refnum<queue>)
                        n227 = Bundle By Name(cluster=T40 {"Command"=enum."Move by", "Data"=variant(dbl[] [])} ("MSG to Servo"), "Command"=Servo_commands."Move by", "Data"=w417) -> (w413:T40)
                        n228 = call "Put in mailbox.vi"("Message"=w413, "Queue in"=w415) -> ()  [unwired: 7 in, 3 out]
                      }
                    }
                  }
                  event Value Change {
                    w442 = 0.5 ("y")
                    n229 = event-data() -> ("CtlRef"=w421:refnum<vi>)  [unwired: 1 in, 5 out]
                    n230 = Unbundle By Name(w420) -> ("Servo"=w419:T10[])
                    n231 = call "Extract axis properties.vi"("Name"=Axis_names."AxisZ_right", "All servo status"=w419) -> ("Servo"=w440:T10, "Index"=w431:i32)  [unwired: 6 in, 1 out]
                    n232 = call "Extract axis properties.vi"("Name"=Axis_names."AxisZ_middle", "All servo status"=w419) -> ("Servo"=w439:T10, "Index"=w430:i32)  [unwired: 6 in, 1 out]
                    n233 = call "Extract axis properties.vi"("Name"=Axis_names."AxisZ_left", "All servo status"=w419) -> ("Servo"=w441:T10, "Index"=w432:i32)  [unwired: 6 in, 1 out]
                    n234 = Unbundle By Name(w440) -> ("Position"=w426:dbl, "Pos limit"=w434:dbl)
                    n235 = Unbundle By Name(w439) -> ("Position"=w425:dbl, "Pos limit"=w433:dbl)
                    n236 = Unbundle By Name(w441) -> ("Position"=w424:dbl, "Pos limit"=w435:dbl)
                    n237 = Subtract(x=w434, y=w442) -> (x-y=w445:dbl)
                    n238 = Subtract(x=w433, y=w442) -> (x-y=w444:dbl)
                    n239 = Subtract(x=w435, y=w442) -> (x-y=w446:dbl)
                    n240 = property class="Bool (strict)"(reference=w421, "Value"=FALSE) -> ()  [unwired: 1 in, 2 out]
                    n241 = Less?(x=w425, y=w444) -> (x < y?=w429:bool)
                    n242 = Less?(x=w424, y=w446) -> (x < y?=w427:bool)
                    n243 = Less?(x=w426, y=w445) -> (x < y?=w428:bool)
                    n244 = Compound Arithmetic op=AND(w428, w429, w427) -> (w443:bool)
                    n245 = case shown="True" w443 {
                      tunnel: w442 -> [_ w454]
                      tunnel: w432 -> [_ w455]
                      tunnel: w431 -> [_ w453]
                      tunnel: w430 -> [_ w452]
                      tunnel: w423 -> [_ w449]
                      frame False {
                      }
                      frame True {
                        n246 = Initialize Array(0.0 ("element"), 5 ("dimension size")) -> (w461:dbl[])
                        n247 = Replace Array Subset(array=w461, new element=w454, index=w453) -> (w458:dbl[])
                        n248 = Replace Array Subset(array=w458, new element=w454, index=w452) -> (w457:dbl[])
                        n249 = Replace Array Subset(array=w457, new element=w454, index=w455) -> (w456:dbl[])
                        n250 = Bundle By Name(cluster=T40 {"Command"=enum."Move by", "Data"=variant(dbl[] [])} ("MSG to Servo"), "Command"=Servo_commands."Move by", "Data"=w456) -> (w450:T40)
                        n251 = Unbundle By Name(w449) -> ("Tmp_C"=w451:refnum<queue>)
                        n252 = call "Put in mailbox.vi"("Message"=w450, "Queue in"=w451) -> ()  [unwired: 7 in, 3 out]
                      }
                    }
                  }
                  event Value Change {
                    w484 = 0.5 ("y")
                    n253 = event-data() -> ("CtlRef"=w465:refnum<vi>)  [unwired: 1 in, 5 out]
                    n254 = Unbundle By Name(w463) -> ("Servo"=w464:T10[])
                    n255 = call "Extract axis properties.vi"("Name"=Axis_names."AxisZ_middle", "All servo status"=w464) -> ("Servo"=w480:T10, "Index"=w473:i32)  [unwired: 6 in, 1 out]
                    n256 = call "Extract axis properties.vi"("Name"=Axis_names."AxisZ_left", "All servo status"=w464) -> ("Servo"=w483:T10, "Index"=w472:i32)  [unwired: 6 in, 1 out]
                    n257 = call "Extract axis properties.vi"("Name"=Axis_names."AxisZ_right", "All servo status"=w464) -> ("Servo"=w481:T10, "Index"=w471:i32)  [unwired: 6 in, 1 out]
                    n258 = Unbundle By Name(w481) -> ("Position"=w469:dbl, "Neg limit"=w476:dbl)
                    n259 = Unbundle By Name(w483) -> ("Position"=w470:dbl, "Neg limit"=w477:dbl)
                    n260 = Unbundle By Name(w480) -> ("Position"=w468:dbl, "Neg limit"=w475:dbl)
                    n261 = property class="Bool (strict)"(reference=w465, "Value"=FALSE) -> ()  [unwired: 1 in, 2 out]
                    n262 = Add(x=w477, y=w484) -> (x+y=w491:dbl)
                    n263 = Add(x=w476, y=w484) -> (x+y=w490:dbl)
                    n264 = Add(x=w475, y=w484) -> (x+y=w489:dbl)
                    n265 = Greater?(x=w470, y=w491) -> (0:w488:bool)
                    n266 = Greater?(x=w469, y=w490) -> (0:w487:bool)
                    n267 = Greater?(x=w468, y=w489) -> (0:w485:bool)
                    n268 = Negate(x=w484) -> (-x=w474:dbl)
                    n269 = Compound Arithmetic op=AND(w488, w487, w485) -> (w486:bool)
                    n270 = case shown="True" w486 {
                      tunnel: w474 -> [_ w500]
                      tunnel: w473 -> [_ w499]
                      tunnel: w472 -> [_ w498]
                      tunnel: w471 -> [_ w497]
                      tunnel: w467 -> [_ w493]
                      frame False {
                      }
                      frame True {
                        n271 = Initialize Array(0.0 ("element"), 5 ("dimension size")) -> (w506:dbl[])
                        n272 = Replace Array Subset(array=w506, new element=w500, index=w499) -> (w503:dbl[])
                        n273 = Replace Array Subset(array=w503, new element=w500, index=w498) -> (w502:dbl[])
                        n274 = Replace Array Subset(array=w502, new element=w500, index=w497) -> (w501:dbl[])
                        n275 = Bundle By Name(cluster=T40 {"Command"=enum."Move by", "Data"=variant(dbl[] [])} ("MSG to Servo"), "Command"=Servo_commands."Move by", "Data"=w501) -> (w494:T40)
                        n276 = Unbundle By Name(w493) -> ("Table_C"=w495:refnum<queue>)
                        n277 = call "Put in mailbox.vi"("Message"=w494, "Queue in"=w495) -> ()  [unwired: 7 in, 3 out]
                      }
                    }
                  }
                  event Value Change {
                    w518 = 0.5 ("y")
                    n278 = event-data() -> ("CtlRef"=w510:refnum<vi>)  [unwired: 1 in, 5 out]
                    n279 = Unbundle By Name(w509) -> ("Servo"=w508:T10[])
                    n280 = call "Extract axis properties.vi"("Name"=Axis_names."AxisZ_left", "All servo status"=w508) -> ("Servo"=w517:T10, "Index"=w514:i32)  [unwired: 6 in, 1 out]
                    n281 = Unbundle By Name(w517) -> ("Position"=w513:dbl, "Pos limit"=w515:dbl)
                    n282 = Subtract(x=w515, y=w518) -> (x-y=w519:dbl)
                    n283 = property class="Bool (strict)"(reference=w510, "Value"=FALSE) -> ()  [unwired: 1 in, 2 out]
                    n284 = Less?(x=w513, y=w519) -> (x < y?=w520:bool)
                    n285 = case shown="True" w520 {
                      tunnel: w518 -> [_ w531]
                      tunnel: w514 -> [_ w526]
                      tunnel: w512 -> [_ w522]
                      frame False {
                      }
                      frame True {
                        n286 = Initialize Array(0.0 ("element"), 5 ("dimension size")) -> (w530:dbl[])
                        n287 = Replace Array Subset(array=w530, new element=w531, index=w526) -> (w527:dbl[])
                        n288 = Bundle By Name(cluster=T40 {"Command"=enum."Move by", "Data"=variant(dbl[] [])} ("MSG to Servo"), "Command"=Servo_commands."Move by", "Data"=w527) -> (w523:T40)
                        n289 = Unbundle By Name(w522) -> ("Table_C"=w524:refnum<queue>)
                        n290 = call "Put in mailbox.vi"("Message"=w523, "Queue in"=w524) -> ()  [unwired: 7 in, 3 out]
                      }
                    }
                  }
                  event Value Change {
                    w543 = 0.5 ("y")
                    n291 = event-data() -> ("CtlRef"=w535:refnum<vi>)  [unwired: 1 in, 5 out]
                    n292 = Unbundle By Name(w533) -> ("Servo"=w534:T10[])
                    n293 = call "Extract axis properties.vi"("Name"=Axis_names."AxisZ_left", "All servo status"=w534) -> ("Servo"=w542:T10, "Index"=w539:i32)  [unwired: 6 in, 1 out]
                    n294 = Unbundle By Name(w542) -> ("Position"=w538:dbl, "Neg limit"=w540:dbl)
                    n295 = property class="Bool (strict)"(reference=w535, "Value"=FALSE) -> ()  [unwired: 1 in, 2 out]
                    n296 = Add(x=w540, y=w543) -> (x+y=w544:dbl)
                    n297 = Greater?(x=w538, y=w544) -> (0:w545:bool)
                    n298 = case shown="True" w545 {
                      tunnel: w543 -> [_ w555]
                      tunnel: w539 -> [_ w551]
                      tunnel: w537 -> [_ w548]
                      frame False {
                      }
                      frame True {
                        n299 = Negate(x=w555) -> (-x=w557:dbl)
                        n300 = Initialize Array(0.0 ("element"), 5 ("dimension size")) -> (w556:dbl[])
                        n301 = Replace Array Subset(array=w556, new element=w557, index=w551) -> (w552:dbl[])
                        n302 = Bundle By Name(cluster=T40 {"Command"=enum."Move by", "Data"=variant(dbl[] [])} ("MSG to Servo"), "Command"=Servo_commands."Move by", "Data"=w552) -> (w547:T40)
                        n303 = Unbundle By Name(w548) -> ("Table_C"=w549:refnum<queue>)
                        n304 = call "Put in mailbox.vi"("Message"=w547, "Queue in"=w549) -> ()  [unwired: 7 in, 3 out]
                      }
                    }
                  }
                  event Value Change {
                    w569 = 0.5 ("y")
                    n305 = event-data() -> ("CtlRef"=w561:refnum<vi>)  [unwired: 1 in, 5 out]
                    n306 = Unbundle By Name(w559) -> ("Servo"=w560:T10[])
                    n307 = call "Extract axis properties.vi"("Name"=Axis_names."AxisZ_right", "All servo status"=w560) -> ("Servo"=w568:T10, "Index"=w565:i32)  [unwired: 6 in, 1 out]
                    n308 = property class="Bool (strict)"(reference=w561, "Value"=FALSE) -> ()  [unwired: 1 in, 2 out]
                    n309 = Unbundle By Name(w568) -> ("Position"=w564:dbl, "Pos limit"=w566:dbl)
                    n310 = Subtract(x=w566, y=w569) -> (x-y=w571:dbl)
                    n311 = Less?(x=w564, y=w571) -> (x < y?=w570:bool)
                    n312 = case shown="True" w570 {
                      tunnel: w569 -> [_ w581]
                      tunnel: w565 -> [_ w577]
                      tunnel: w563 -> [_ w573]
                      frame False {
                      }
                      frame True {
                        n313 = Initialize Array(0.0 ("element"), 5 ("dimension size")) -> (w582:dbl[])
                        n314 = Replace Array Subset(array=w582, new element=w581, index=w577) -> (w578:dbl[])
                        n315 = Bundle By Name(cluster=T40 {"Command"=enum."Move by", "Data"=variant(dbl[] [])} ("MSG to Servo"), "Command"=Servo_commands."Move by", "Data"=w578) -> (w574:T40)
                        n316 = Unbundle By Name(w573) -> ("Table_C"=w575:refnum<queue>)
                        n317 = call "Put in mailbox.vi"("Message"=w574, "Queue in"=w575) -> ()  [unwired: 7 in, 3 out]
                      }
                    }
                  }
                  event Value Change {
                    w593 = 0.5 ("y")
                    n318 = event-data() -> ("CtlRef"=w586:refnum<vi>)  [unwired: 1 in, 5 out]
                    n319 = Unbundle By Name(w584) -> ("Servo"=w585:T10[])
                    n320 = call "Extract axis properties.vi"("Name"=Axis_names."AxisZ_right", "All servo status"=w585) -> ("Servo"=w592:T10, "Index"=w590:i32)  [unwired: 6 in, 1 out]
                    n321 = property class="Bool (strict)"(reference=w586, "Value"=FALSE) -> ()  [unwired: 1 in, 2 out]
                    n322 = Unbundle By Name(w592) -> ("Position"=w589:dbl, "Neg limit"=w595:dbl)
                    n323 = Add(x=w595, y=w593) -> (x+y=w594:dbl)
                    n324 = Greater?(x=w589, y=w594) -> (0:w596:bool)
                    n325 = case shown="True" w596 {
                      tunnel: w593 -> [_ w606]
                      tunnel: w590 -> [_ w602]
                      tunnel: w588 -> [_ w598]
                      frame False {
                      }
                      frame True {
                        n326 = Negate(x=w606) -> (-x=w608:dbl)
                        n327 = Initialize Array(0.0 ("element"), 5 ("dimension size")) -> (w607:dbl[])
                        n328 = Replace Array Subset(array=w607, new element=w608, index=w602) -> (w603:dbl[])
                        n329 = Bundle By Name(cluster=T40 {"Command"=enum."Move by", "Data"=variant(dbl[] [])} ("MSG to Servo"), "Command"=Servo_commands."Move by", "Data"=w603) -> (w599:T40)
                        n330 = Unbundle By Name(w598) -> ("Table_C"=w600:refnum<queue>)
                        n331 = call "Put in mailbox.vi"("Message"=w599, "Queue in"=w600) -> ()  [unwired: 7 in, 3 out]
                      }
                    }
                  }
                  event Value Change {
                    w620 = 0.5 ("y")
                    n332 = event-data() -> ("CtlRef"=w612:refnum<vi>)  [unwired: 1 in, 5 out]
                    n333 = Unbundle By Name(w610) -> ("Servo"=w611:T10[])
                    n334 = call "Extract axis properties.vi"("Name"=Axis_names."AxisZ_middle", "All servo status"=w611) -> ("Servo"=w619:T10, "Index"=w616:i32)  [unwired: 6 in, 1 out]
                    n335 = Unbundle By Name(w619) -> ("Position"=w615:dbl, "Pos limit"=w617:dbl)
                    n336 = property class="Bool (strict)"(reference=w612, "Value"=FALSE) -> ()  [unwired: 1 in, 2 out]
                    n337 = Subtract(x=w617, y=w620) -> (x-y=w621:dbl)
                    n338 = Less?(x=w615, y=w621) -> (x < y?=w622:bool)
                    n339 = case shown="True" w622 {
                      tunnel: w620 -> [_ w632]
                      tunnel: w616 -> [_ w628]
                      tunnel: w614 -> [_ w624]
                      frame False {
                      }
                      frame True {
                        n340 = Initialize Array(0.0 ("element"), 5 ("dimension size")) -> (w633:dbl[])
                        n341 = Replace Array Subset(array=w633, new element=w632, index=w628) -> (w629:dbl[])
                        n342 = Bundle By Name(cluster=T40 {"Command"=enum."Move by", "Data"=variant(dbl[] [])} ("MSG to Servo"), "Command"=Servo_commands."Move by", "Data"=w629) -> (w625:T40)
                        n343 = Unbundle By Name(w624) -> ("Table_C"=w626:refnum<queue>)
                        n344 = call "Put in mailbox.vi"("Message"=w625, "Queue in"=w626) -> ()  [unwired: 7 in, 3 out]
                      }
                    }
                  }
                  event Value Change {
                    w645 = 0.5 ("y")
                    n345 = event-data() -> ("CtlRef"=w637:refnum<vi>)  [unwired: 1 in, 5 out]
                    n346 = Unbundle By Name(w635) -> ("Servo"=w636:T10[])
                    n347 = call "Extract axis properties.vi"("Name"=Axis_names."AxisZ_middle", "All servo status"=w636) -> ("Servo"=w643:T10, "Index"=w641:i32)  [unwired: 6 in, 1 out]
                    n348 = property class="Bool (strict)"(reference=w637, "Value"=FALSE) -> ()  [unwired: 1 in, 2 out]
                    n349 = Unbundle By Name(w643) -> ("Position"=w640:dbl, "Neg limit"=w642:dbl)
                    n350 = Add(x=w642, y=w645) -> (x+y=w646:dbl)
                    n351 = Greater?(x=w640, y=w646) -> (0:w647:bool)
                    n352 = case shown="True" w647 {
                      tunnel: w645 -> [_ w657]
                      tunnel: w641 -> [_ w653]
                      tunnel: w639 -> [_ w650]
                      frame False {
                      }
                      frame True {
                        n353 = Negate(x=w657) -> (-x=w659:dbl)
                        n354 = Initialize Array(0.0 ("element"), 5 ("dimension size")) -> (w658:dbl[])
                        n355 = Replace Array Subset(array=w658, new element=w659, index=w653) -> (w654:dbl[])
                        n356 = Bundle By Name(cluster=T40 {"Command"=enum."Move by", "Data"=variant(dbl[] [])} ("MSG to Servo"), "Command"=Servo_commands."Move by", "Data"=w654) -> (w649:T40)
                        n357 = Unbundle By Name(w650) -> ("Table_C"=w651:refnum<queue>)
                        n358 = call "Put in mailbox.vi"("Message"=w649, "Queue in"=w651) -> ()  [unwired: 7 in, 3 out]
                      }
                    }
                  }
                  event Value Change {
                    n359 = event-data() -> ()  [unwired: 1 in, 6 out]
                    n360 = Unbundle By Name(w673) -> ("MW_C"=w672:refnum<queue>)
                    n361 = Unbundle By Name("VID control") -> ("AMC"=w671:u16, "Multip"=w670:u16, "Base frequency [GHz]"=w678:dbl, "End frequency [GHz]"=w679:dbl, "Im frequency [MHz]"=w680:dbl, "Sweep up [ms]"=w661:dbl, "Reset trigger?"=w663:bool)
                    n362 = Multiply(x=w671, y=w670) -> (x*y=w665:u16)
                    n363 = Divide(x=w678, y=w665) -> (x/y=w669:dbl)
                    n364 = Divide(x=w661, y=2.0) -> (x/y=w666:dbl)
                    n365 = Divide(x=w679, y=w665) -> (x/y=w668:dbl)
                    n366 = Divide(x=w680, y=w665) -> (x/y=w667:dbl)
                    n367 = Bundle By Name(cluster=T42 {"Start [GHz]"=8.0, "End [GHz] "=8.0, "Sweep up\ntime [ms]"=0.0, "Sweep down\ntime [ms]"=0.0, "Intermidiate [MHz]"=0.0, "Reset trigger"=FALSE} ("Sweep parameters"), "Start [GHz]"=w669, "End [GHz]"=w668, "Intermidiate [MHz]"=w667, "Sweep down\ntime [ms]"=w666, "Sweep up\ntime [ms]"=w661, "Reset trigger"=w663) -> (w675:T42)
                    n368 = Bundle By Name(cluster=T43 {"Command"=enum."Set parameters", "Data"=variant} ("Incoming msg"), "Command"=THz_commands_enum."Set parameters", "Data"=w675) -> (w676:T43)
                    n369 = call "Put in mailbox.vi"("Message"=w676, "Queue in"=w672) -> ()  [unwired: 7 in, 3 out]
                  }
                  event Value Change {
                    n370 = event-data() -> ()  [unwired: 1 in, 6 out]
                    n371 = local read "VID control"() -> (w690:T16)
                    n372 = Unbundle By Name(w690) -> ("AMC"=w687:u16, "Multip"=w686:u16)
                    n373 = Multiply(x=w687, y=w686) -> (x*y=w685:u16)
                    n374 = Multiply(x=14.0, y=w685) -> (x*y=w684:dbl)
                    n375 = Multiply(x=9.0, y=w685) -> (x*y=w683:dbl)
                    n376 = property on="AMC" class="Ring (strict)"("Minimum"=w683, "Maximum"=w684) -> ()  [unwired: 2 in, 2 out]
                    n377 = property on="Base frequency [GHz]" class="DigNum (strict)"("Minimum"=w683, "Maximum"=w684) -> ()  [unwired: 2 in, 2 out]
                  }
                  event Value Change {
                    n378 = event-data() -> ("CtlRef"=w699:refnum<vi>, "NewVal"=w696:dbl)  [unwired: 1 in]
                    n379 = property class="DigNum (strict)"(reference=w699) -> ("Label.Text"=w698:string)  [unwired: 1 in, 2 out]
                    n380 = Unbundle By Name(w706) -> ("Data_Aq"=w705:refnum<queue>)
                    n381 = local read "Sample holder"() -> (w693:T13)
                    n382 = case shown="\"Time constant [ms]\"" w698 {
                      tunnel: [MFLI_node."None" ("parameter") MFLI_node."filter_constant [ms]" ("parameter") MFLI_node."filter_order [-]" ("parameter") MFLI_node."osc_freq [kHz]" ("parameter") MFLI_node."out_ampl [V]" ("parameter")] -> w694
                      tunnel: w696 -> [_ w710 w712 w714 w717]
                      tunnel: [_ w710 w712 w714 w730] -> w697
                      tunnel: w693 -> [_ _ _ _ w728]
                      tunnel: "Acquisition controls" -> [_ _ _ _ w727]
                      tunnel: [_ _ _ _ w715] -> _
                      frame "Unknown", Default {
                      }
                      frame "Time constant [ms]" {
                      }
                      frame "Filter order" {
                      }
                      frame "F_Mod [kHz]" {
                      }
                      frame "Amp_Mod [mV]" {
                        n383 = case shown="\"Rotator\"" w728 {
                          tunnel: [w734 w737 w740 w743] -> w726
                          tunnel: [w733 w736 w739 w742] -> w722
                          tunnel: [w732 w735 w738 w741] -> w716
                          frame "Simple", Default {
                            w732 = 0.0  # G/A
                            w733 = 8.9  # R
                            w734 = 0.0017  # L
                          }
                          frame "Carousel" {
                            w735 = 0.0  # G/A
                            w736 = 8.9  # R
                            w737 = 0.0017  # L
                          }
                          frame "Chip" {
                            w738 = 0.0  # G/A
                            w739 = 8.9  # R
                            w740 = 0.0017  # L
                          }
                          frame "Rotator" {
                            w741 = 0.0  # G/A
                            w742 = 8.9  # R
                            w743 = 0.0017  # L
                          }
                        }
                        n384 = Unbundle By Name(w727) -> ("ACQ parameters.F_Mod [kHz]"=w724:dbl)
                        n385 = Square(x=w722) -> (x^2=w720:dbl)
                        n386 = Divide(x=w717, y=1000.0) -> (x/y=w730:dbl)
                        n387 = Compound Arithmetic op=MULTIPLY(w724, 6.283185307179586, w726) -> (w723:dbl)
                        n388 = Square(x=w723) -> (x^2=w721:dbl)
                        n389 = Add(x=w721, y=w720) -> (x+y=w719:dbl)
                        n390 = Square Root(x=w719) -> (sqrt(x)=w718:dbl)
                        n391 = Compound Arithmetic op=MULTIPLY(w716, w718) -> (w715:dbl)
                      }
                    }
                    n392 = Bundle(cluster=T44 {"parameter"=enum."filter_order [-]", "value"=0.0} ("Parameter to set"), "parameter"=w694, "value"=w697) -> (w700:T44)
                    n393 = Build Array(w700) -> (w695:T44[])
                    n394 = Bundle By Name(cluster=T47 {"Command"=enum."Initialize", "Data"=variant} ("MSG for  ACQ"), "Command"=MFLI_command_enum."Set individual parameters", "Data"=w695) -> (w702:T47)
                    n395 = call "Put in mailbox.vi"("Message"=w702, "Queue in"=w705) -> ()  [unwired: 7 in, 3 out]
                  }
                  event Value Change {
                    w747 = T44 {"parameter"=enum."filter_order [-]", "value"=0.0} ("Parameter to set")
                    n396 = event-data() -> ("NewVal"=w745:u16)  [unwired: 1 in, 2 out]
                    n397 = Unbundle By Name(w755) -> ("Data_Aq"=w754:refnum<queue>)
                    n398 = Bundle(cluster=w747, "parameter"=MFLI_node."enable output", "value"=w745) -> (w750:T44)
                    n399 = Bundle(cluster=w747, "parameter"=MFLI_node."enamble ampl", "value"=w745) -> (w744:T44)
                    n400 = Build Array(w750, w744) -> (w749:T44[])
                    n401 = Bundle By Name(cluster=T47 {"Command"=enum."Initialize", "Data"=variant} ("MSG for  ACQ"), "Command"=MFLI_command_enum."Set individual parameters", "Data"=w749) -> (w751:T47)
                    n402 = call "Put in mailbox.vi"("Message"=w751, "Queue in"=w754) -> ()  [unwired: 7 in, 3 out]
                  }
                  event Value Change {
                    n403 = event-data() -> ("CtlRef"=w762:refnum<vi>, "NewVal"=w760:dbl)  [unwired: 1 in]
                    n404 = property class="DigNum (strict)"(reference=w762) -> ("Label.Text"=w761:string)  [unwired: 1 in, 2 out]
                    n405 = Unbundle By Name(w766) -> ("Tmp_C"=w763:refnum<queue>)
                    n406 = Bundle(cluster=T48 {"Heater"="None", "Tmp [K]"=0.0} ("Set point"), "Heater"=w761, "Tmp [K]"=w760) -> (w757:T48)
                    n407 = Bundle By Name(cluster=T50 {"Command"=enum."Initialize", "Data"=variant}, "Command"=TC_commands."Set point", "Data"=w757) -> (w764:T50)
                    n408 = call "Put in mailbox.vi"("Message"=w764, "Queue in"=w763) -> ()  [unwired: 7 in, 3 out]
                  }
                  event "Password is admin": Value Change {
                    n409 = event-data() -> ("NewVal"=w772:string)  [unwired: 1 in, 1 out]
                    n410 = Equal?(x="admin", y=w772) -> (x = y?=w768:bool)
                    n411 = case shown="True" w768 {
                      tunnel: [T32."Disabled and Grayed Out" ("Disabled") T32."Enabled" ("Disabled")] -> w769
                      frame False {
                      }
                      frame True {
                      }
                    }
                    n412 = local read "Instr control refs"() -> (w770:refnum<vi>[])
                    n413 = call "Dis- or en- able controls.vi"("Disabled"=w769, "Control referencies"=w770) -> ()  [unwired: 9 in, 1 out]
                  }
                }
              }
              frame "MAP measurement" {
                n414 = event shown="[3] \"Direct stop meas. btn\": Value Change" {
                  selector: _ -> [_ _ _ _ _]
                  dyn-events: _ -> [_ _ _ _ _]
                  timeout: 0 -> [_ _ _ _ _]
                  tunnel: w783 -> [w786 w802 w814 w823 w850]
                  tunnel: [w786 w801 w814 w823 w850] -> w782
                  tunnel: w780 -> [_ _ _ w822 _]
                  tunnel: [w784 "Map parameters" w813 w819 w847] -> w779
                  tunnel: w778 -> [w784 _ w813 w819 w847]
                  tunnel: [w785 w799 w812 w818 w846] -> w776
                  tunnel: w777 -> [w785 w800 w812 w817 w846]
                  event Timeout {
                    n415 = event-data() -> ()  [unwired: 1 in, 3 out]
                  }
                  event "Run MAP btn": Value Change {
                    n416 = event-data() -> ()  [unwired: 1 in, 6 out]
                    n417 = control-ref of="Run MAP btn"() -> (w792:refnum<vi>)
                    n418 = control-ref of="Open measurement"() -> (w794:refnum<vi>)
                    n419 = control-ref of="Map parameters"() -> (w793:refnum<vi>)
                    n420 = local read "Instr control refs"() -> (w797:refnum<vi>[])
                    n421 = Build Array (concatenate)(w797, w792, w794, w793) -> (w796:refnum<vi>[])
                    n422 = call "Dis- or en- able controls.vi"("Disabled"=T32."Disabled and Grayed Out", "Control referencies"=w796) -> ()  [unwired: 9 in, 1 out]
                    n423 = control-ref of="Direct stop meas. btn"() -> (w788:refnum<vi>)
                    n424 = Build Array(w788) -> (w790:refnum<vi>[])
                    n425 = call "Dis- or en- able controls.vi"("Disabled"=T32."Enabled", "Control referencies"=w790) -> ()  [unwired: 9 in, 1 out]
                    n426 = Bundle By Name(cluster=w800, "Experiment state"=experiment_state."Preparation" ("Value")) -> (w799:T24)
                    n427 = call "simple Shift string array.vi"("Element in"="Preparing for measurement.", "Array in"=w802) -> ("Array out"=w801:string[])  [unwired: 8 in, 1 out]
                  }
                  event Value Change {
                    n428 = event-data() -> ()  [unwired: 1 in, 6 out]
                    n429 = local read "Map parameters"() -> (w810:T22)
                    n430 = Unbundle By Name(w810) -> ("Points"=w811:u32, "Sampling rate"=w808:T23)
                    n431 = Scale By Power Of 2(n=w808, x=ext 1.0) -> (x*2^n=w807:ext)
                    n432 = Divide(x=ext 60000000.0, y=w807) -> (x/y=w806:ext)
                    n433 = Divide(x=w811, y=w806) -> (x/y=w809:ext)
                    n434 = Bundle By Name(cluster=w810, "Sweep [s]"=w809) -> (w803:T22)
                    n435 = local write "Map parameters"(w803) -> ()
                  }
                  event "Direct stop meas. btn": Value Change {
                    n436 = event-data() -> ("NewVal"=w821:bool)  [unwired: 1 in, 5 out]
                    n437 = call "Timeout dialoge Abbort.vi"("Enable"=w821, "Message to Display"="Realy abbort measurement?", "timeout[ms]"=u32 5000) -> ("Yes"=w820:bool)  [unwired: 15 in, 1 out]
                    n438 = case shown="True" w820 {
                      tunnel: w822 -> [_ w843]
                      tunnel: w817 -> [w824 w829]
                      tunnel: [w824 w828] -> w818
                      frame False {
                      }
                      frame True {
                        n439 = Unbundle By Name(w843) -> ("Field_C"=w837:refnum<queue>, "Tmp_C"=w838:refnum<queue>, "Angle_C"=w839:refnum<queue>)
                        n440 = local write "Run MAP btn"(FALSE ("Direct stop meas. btn")) -> ()
                        n441 = Bundle By Name(cluster=w829, "Experiment state"=experiment_state."Save" ("Value")) -> (w828:T24)
                        n442 = local read "Instr control refs"() -> (w832:refnum<vi>[])
                        n443 = control-ref of="Map parameters"() -> (w825:refnum<vi>)
                        n444 = control-ref of="Run MAP btn"() -> (w830:refnum<vi>)
                        n445 = Build Array (concatenate)(w830, w825, w832) -> (w833:refnum<vi>[])
                        n446 = call "Put in mailbox.vi"("Message"=T36 {"Command"=enum."Stop ramping", "Data"=variant} ("MSG to magnet"), "Queue in"=w837) -> ("error out"=w836:errorcluster)  [unwired: 7 in, 2 out]
                        n447 = call "Put in mailbox.vi"("error in (no error)"=w836, "Message"=T50 {"Command"=enum."Stop tmp change", "Data"=variant} ("MSG for VTI"), "Queue in"=w838) -> ("error out"=w835:errorcluster)  [unwired: 6 in, 2 out]
                        n448 = call "Put in mailbox.vi"("error in (no error)"=w835, "Message"=T51 {"Command"=enum."Stop movement", "Data"=variant} ("MSG to rotator"), "Queue in"=w839) -> ("error out"=w826:errorcluster)  [unwired: 6 in, 2 out]
                        n449 = call "Dis- or en- able controls.vi"("error in"=w826, "Disabled"=T32."Enabled", "Control referencies"=w833) -> ()  [unwired: 8 in, 1 out]
                      }
                    }
                  }
                  event "Sample name", "Description": Value Change {
                    n450 = event-data() -> ("CtlRef"=w845:refnum<vi>, "NewVal"=w849:string)  [unwired: 1 in, 4 out]
                    n451 = Search and Replace String(replace all?=TRUE ("replace all? (F)"), input string=w849, search string="[<>:\"/\\|?*%]" ("regular expression"), replace string="-" ("replace string (\"\")")) -> (result string=w844:string)  [unwired: 4 in, 3 out]
                    n452 = property class="Str"(reference=w845, "Value"=w844) -> ()  [unwired: 1 in, 2 out]
                  }
                }
              }
              frame "Measurement review" {
                n453 = event shown="[2] \"Open measurement\": Value Change" {
                  selector: _ -> [_ _ _]
                  dyn-events: _ -> [_ _ _]
                  timeout: 0 -> [_ _ _]
                  event Timeout {
                    n454 = event-data() -> ()  [unwired: 1 in, 3 out]
                  }
                  event "Data file to show": Value Change {
                    n455 = event-data() -> ()  [unwired: 1 in, 6 out]
                    n456 = local read "Review results"() -> (w877:T4[])
                    n457 = Index Array(array=w877, index="Data file to show") -> (element=w875:T4)
                    n458 = Build Array("Data file to show") -> ()  [unwired: 1 out]
                    n459 = Unbundle By Name(w875) -> ("Start F [GHz]"=w860:dbl, "End F[GHz]"=w863:dbl, "BStart[T]"=w857:dbl, "Bend[T]"=w861:dbl, "Intensity"=w864:dbl[][])
                    n460 = Index Array(array=w864, index (row) #1=0 ("index (row)"), index (col) #2=0 ("disabled index (col)")) -> (element #1=w872:dbl[], element #2=w871:dbl[])  [unwired: 2 in]
                    n461 = Array Size(array=w872) -> (size(s)=w869:i32)
                    n462 = Array Size(array=w871) -> (size(s)=w866:i32)
                    n463 = Subtract(x=w861, y=w857) -> (x-y=w867:dbl)
                    n464 = Subtract(x=w863, y=w860) -> (x-y=w870:dbl)
                    n465 = Divide(x=w867, y=w866) -> (x/y=w858:dbl)
                    n466 = Divide(x=w870, y=w869) -> (x/y=w868:dbl)
                    n467 = Transpose 2D Array(2D array=w864) -> (transposed array=w862:dbl[][])
                    n468 = control-ref of="Map review graph"() -> (w859:refnum<vi>)
                    n469 = property on="Property Node" class="IntGraph (strict)"(reference=w859, "Value"=w862, "XScale.Multiplier"=w868, "XScale.Offset"=w860, "YScale.Multiplier"=w858, "YScale.Offset"=w857, "YScale.ScaleFit"=u8 1 ("Y Scale.Scale Fit")) -> ()  [unwired: 1 in, 2 out]
                  }
                  event "Open measurement": Value Change {
                    n470 = event-data() -> ()  [unwired: 1 in, 1 out]
                    n471 = local read "Folder path"() -> (w880:path)
                    n472 = call "Read MAP data file.vi"("Data folder"=w880) -> ("File name"=w878:string, "Map data ref"=w879:refnum<data-value>, "Error Out"=w881:errorcluster)  [unwired: 8 in]
                    n473 = case shown="No Error" w881 {
                      selector: w881 -> [w901 w908]
                      tunnel: w879 -> [w902 w910]
                      tunnel: w878 -> [w900 _]
                      frame No Error {
                        n474 = local read "Data file to show"() -> (w903:u16)
                        n475 = Delete Data Value Reference(data value reference=w902, error in=w901) -> (data value=w899:T78)  [unwired: 1 out]
                        n476 = local read "Review results"() -> (w905:T4[])
                        n477 = Replace Array Subset(array=w905, new element=w899, index=w903) -> (w904:T4[])
                        n478 = property on="Data file to show" class="Ring (strict)"() -> ("Strings []"=w907:string[])  [unwired: 2 in, 2 out]
                        n479 = local write "Review results"(w904) -> ()
                        n480 = Replace Array Subset(array=w907, new element=w900, index=w903) -> (w906:string[])
                        n481 = property on="Data file to show" class="Ring (strict)"("Strings []"=w906) -> ()  [unwired: 2 in, 2 out]
                        n482 = Unbundle By Name(w899) -> ("Start F [GHz]"=w889:dbl, "End F[GHz]"=w890:dbl, "BStart[T]"=w883:dbl, "Bend[T]"=w885:dbl, "Intensity"=w897:dbl[][])
                        n483 = Index Array(array=w897, index (row) #1=0 ("index (row)"), index (col) #2=0 ("disabled index (col)")) -> (element #1=w894:dbl[], element #2=w893:dbl[])  [unwired: 2 in]
                        n484 = Array Size(array=w894) -> (size(s)=w891:i32)
                        n485 = Array Size(array=w893) -> (size(s)=w886:i32)
                        n486 = Transpose 2D Array(2D array=w897) -> (transposed array=w898:dbl[][])
                        n487 = Subtract(x=w885, y=w883) -> (x-y=w887:dbl)
                        n488 = Subtract(x=w890, y=w889) -> (x-y=w892:dbl)
                        n489 = Divide(x=w887, y=w886) -> (x/y=w884:dbl)
                        n490 = Divide(x=w892, y=w891) -> (x/y=w888:dbl)
                        n491 = property on="Map review graph" class="IntGraph (strict)"("Value"=w898, "XScale.Multiplier"=w888, "XScale.Offset"=w889, "YScale.Multiplier"=w884, "YScale.Offset"=w883, "YScale.ScaleFit"=u8 1 ("Y Scale.Scale Fit")) -> ()  [unwired: 2 in, 2 out]
                      }
                      frame Error {
                        n492 = Delete Data Value Reference(data value reference=w910, error in=w908) -> (error out=w909:errorcluster)  [unwired: 1 out]
                        n493 = call <vilib>:"Clear Errors.vi"("error in (no error)"=w909) -> ()  [unwired: 5 in, 2 out]
                      }
                    }
                  }
                }
              }
            }
          }
          event "Tab Control": Value Change {
            n494 = event-data() -> ("NewVal"=w912:T6)  [unwired: 1 in, 5 out]
            n495 = case shown="\"Adjustment\"" w912 {
              frame "Page Status", Default {
              }
              frame "Adjustment" {
              }
            }
          }
          event "Disconnect": Value Change {
            n496 = event-data() -> ()  [unwired: 1 in, 6 out]
            n497 = local read "Select module"() -> (w916:T7)
            n498 = Equal?(x=w916, y=T31."All") -> (x = y?=w917:bool)
            n499 = case shown="True" w917 {
              tunnel: w915 -> [w922 w948]
              tunnel: w916 -> [w923 _]
              frame False {
                n500 = case shown="\"MAG\"" w923 {
                  tunnel: w922 -> [w927 w931 w935 w936 w943 w947 _]
                  frame "MAG" {
                    n501 = Unbundle By Name(w927) -> ("Field_C"=w925:refnum<queue>)
                    n502 = call "Put in mailbox.vi"("Priority? (F)"=TRUE ("Priority?"), "Message"=T36 {"Command"=enum."Eval temperatures", "Data"=variant} ("MSG to magnet"), "Queue in"=w925) -> ()  [unwired: 6 in, 3 out]
                  }
                  frame "VTI" {
                    n503 = Unbundle By Name(w931) -> ("Tmp_C"=w929:refnum<queue>)
                    n504 = call "Put in mailbox.vi"("Priority? (F)"=TRUE ("Priority?"), "Message"=T50 {"Command"=enum."End", "Data"=variant} ("MSG for VTI"), "Queue in"=w929) -> ()  [unwired: 6 in, 3 out]
                  }
                  frame "THz" {
                    n505 = Unbundle By Name(w935) -> ("MW_C"=w933:refnum<queue>)
                    n506 = call "Put in mailbox.vi"("Priority? (F)"=TRUE ("Priority?"), "Message"=T43 {"Command"=enum."End", "Data"=variant} ("Incoming msg"), "Queue in"=w933) -> ()  [unwired: 6 in, 3 out]
                  }
                  frame "ACQ" {
                    n507 = Unbundle By Name(w936) -> ("Data_Aq"=w938:refnum<queue>)
                    n508 = call "Put in mailbox.vi"("Priority? (F)"=TRUE ("Priority?"), "Message"=T47 {"Command"=enum."End", "Data"=variant} ("MSG for  ACQ"), "Queue in"=w938) -> ()  [unwired: 6 in, 3 out]
                  }
                  frame "SERV" {
                    n509 = Unbundle By Name(w943) -> ("Table_C"=w941:refnum<queue>)
                    n510 = call "Put in mailbox.vi"("Priority? (F)"=TRUE ("Priority?"), "Message"=T40 {"Command"=enum."End", "Data"=variant(dbl[] [])} ("MSG to Servo"), "Queue in"=w941) -> ()  [unwired: 6 in, 3 out]
                  }
                  frame "ROT" {
                    n511 = Unbundle By Name(w947) -> ("Angle_C"=w945:refnum<queue>)
                    n512 = call "Put in mailbox.vi"("Priority? (F)"=TRUE ("Priority?"), "Message"=cluster{"Command":T52, "Data":variant} {"Command"=enum."End", "Data"=variant} ("MSG to rotator"), "Queue in"=w945) -> ()  [unwired: 6 in, 3 out]
                  }
                  frame "None", Default {
                  }
                }
              }
              frame True {
                n513 = control-ref of="Instr status"() -> (w949:refnum<vi>)
                n514 = property class="Clust (strict)"(reference=w949) -> ("Controls[]"=w950:refnum<vi>[])  [unwired: 1 in, 2 out]
                n515 = for {
                  tunnel: w950 -> [w956] mode=indexing
                  tunnel: w948 -> [w954]
                  n516 = property class="Ctl"(reference=w956) -> ("Label.Text"=w955:string, "Value"=w953:variant)  [unwired: 1 in, 2 out]
                  n517 = Variant To Data(type=FALSE, Variant=w953) -> (data=w951:bool)  [unwired: 1 in, 1 out]
                  n518 = case shown="True" w951 {
                    tunnel: w955 -> [_ w958]
                    tunnel: w954 -> [_ w957]
                    frame False {
                    }
                    frame True {
                      n519 = case shown="\"Mag\"" w958 {
                        tunnel: w957 -> [w962 w963 w970 w974 w978 w982 w986 _]
                        frame "Mag" {
                          n520 = Unbundle By Name(w962) -> ("Field_C"=w960:refnum<queue>)
                          n521 = call "Put in mailbox.vi"("Priority? (F)"=TRUE ("Priority?"), "Message"=T36 {"Command"=enum."Eval temperatures", "Data"=variant} ("MSG to magnet"), "Queue in"=w960) -> ()  [unwired: 6 in, 3 out]
                        }
                        frame "SMU" {
                          n522 = Unbundle By Name(w963) -> ("Mod_M"=w965:refnum<queue>)
                          n523 = call "Put in mailbox.vi"("Priority? (F)"=TRUE ("Priority?"), "Message"=T37 {"Command"=enum."Disconnect", "Data"=variant} ("MSG to Source meter"), "Queue in"=w965) -> ()  [unwired: 6 in, 3 out]
                        }
                        frame "VTI" {
                          n524 = Unbundle By Name(w970) -> ("Tmp_C"=w968:refnum<queue>)
                          n525 = call "Put in mailbox.vi"("Priority? (F)"=TRUE ("Priority?"), "Message"=T50 {"Command"=enum."End", "Data"=variant} ("MSG for VTI"), "Queue in"=w968) -> ()  [unwired: 6 in, 3 out]
                        }
                        frame "THz" {
                          n526 = Unbundle By Name(w974) -> ("MW_C"=w972:refnum<queue>)
                          n527 = call "Put in mailbox.vi"("Priority? (F)"=TRUE ("Priority?"), "Message"=T43 {"Command"=enum."End", "Data"=variant} ("Incoming msg"), "Queue in"=w972) -> ()  [unwired: 6 in, 3 out]
                        }
                        frame "ACQ" {
                          n528 = Unbundle By Name(w978) -> ("Data_Aq"=w976:refnum<queue>)
                          n529 = call "Put in mailbox.vi"("Priority? (F)"=TRUE ("Priority?"), "Message"=T47 {"Command"=enum."End", "Data"=variant} ("MSG for  ACQ"), "Queue in"=w976) -> ()  [unwired: 6 in, 3 out]
                        }
                        frame "Serv" {
                          n530 = Unbundle By Name(w982) -> ("Table_C"=w980:refnum<queue>)
                          n531 = call "Put in mailbox.vi"("Priority? (F)"=TRUE ("Priority?"), "Message"=T40 {"Command"=enum."End", "Data"=variant(dbl[] [])} ("MSG to Servo"), "Queue in"=w980) -> ()  [unwired: 6 in, 3 out]
                        }
                        frame "Rot" {
                          n532 = Unbundle By Name(w986) -> ("Angle_C"=w984:refnum<queue>)
                          n533 = call "Put in mailbox.vi"("Priority? (F)"=TRUE ("Priority?"), "Message"=cluster{"Command":T52, "Data":variant} {"Command"=enum."End", "Data"=variant} ("MSG to rotator"), "Queue in"=w984) -> ()  [unwired: 6 in, 3 out]
                        }
                        frame "Ignore", Default {
                        }
                      }
                    }
                  }
                }
              }
            }
          }
          event "Stop": Value Change {
            n534 = event-data() -> ("NewVal"=w992:bool)  [unwired: 1 in, 5 out]
            n535 = case shown="True" w992 {
              tunnel: w991 -> [_ w996]
              tunnel: [_ w995] -> w990
              frame False {
              }
              frame True {
                # "Can not stop application just like that,\nAll modules must respond first, that they are done."
                n536 = control-ref of="Instr status"() -> (w998:refnum<vi>)
                n537 = property class="Clust (strict)"(reference=w998) -> ("Value"=w993:T79)  [unwired: 1 in, 2 out]
                n538 = property class="Clust (strict)"(reference=w998) -> ("Controls[]"=w999:refnum<vi>[])  [unwired: 1 in, 2 out]
                n539 = Cluster To Array(cluster=w993) -> (array=w997:bool[])
                n540 = Or Array Elements(Boolean array=w997) -> (logical OR=w994:bool)
                n541 = case shown="False" w994 {
                  tunnel: w993 -> [_ _]
                  tunnel: w996 -> [w1058 _]
                  tunnel: [TRUE _] -> w995
                  frame False {
                    n542 = Cluster To Array(cluster=w1058) -> (array=w1059:refnum<queue>[])
                    n543 = local read "loggersRef"() -> (w1050:refnum<file>)
                    n544 = for {
                      tunnel: w1059 -> [w1067] mode=indexing
                      tunnel: [w1060] -> w1055
                      n545 = Wait (ms)(milliseconds to wait=u32 100) -> ()  [unwired: 1 out]
                      n546 = Get Queue Status(queue=w1067) -> (queue out=w1066:refnum<queue>, error out=w1061:errorcluster, # elements in queue=w1064:i32)  [unwired: 2 in, 5 out]
                      n547 = Less Or Equal?(x=w1064, y=0) -> (x <= y?=w1062:bool)
                      n548 = Release Queue(queue=w1066, force destroy? (F)=w1062, error in (no error)=w1061) -> (error out=w1060:errorcluster)  [unwired: 2 out]
                    }
                    n549 = Wait (ms)(milliseconds to wait=u32 2000) -> ()  [unwired: 1 out]
                    n550 = local read "Temperature log ref"() -> (w1054:refnum<file>)
                    n551 = call "Add actual date time to string.vi"("String in"="Program ended") -> ("String out"=w1051:string)  [unwired: 4 in]
                    n552 = call "Write in logger.vi"("String in"=w1051, "logger refnum"=w1050) -> ("refnum out"=w1049:refnum<file>)  [unwired: 2 in, 1 out]
                    n553 = local read "System config file path"() -> (w1048:path)
                    n554 = local read "Acquisition controls"() -> (w1045:T15)
                    n555 = local read "VID control"() -> (w1044:T16)
                    n556 = Close File(refnum=w1049, error in=w1055) -> (error out=w1053:errorcluster)  [unwired: 1 out]
                    n557 = Close File(refnum=w1054, error in=w1053) -> ()  [unwired: 2 out]
                    n558 = call "Open config file.vi"("MAG config file path"=w1048) -> ("error out"=w1046:errorcluster, "Refnum out"=w1047:T76)  [unwired: 7 in, 2 out]
                    n559 = Unbundle By Name(w1045) -> ("ACQ parameters"=w1041:T14)
                    n560 = call <userlib>:"Write Section Cluster__ogtk.vi"("error in (no error)"=w1046, "Section Formatted Cluster"=w1044, "refnum"=w1047) -> ("error out"=w1043:errorcluster, "dup refnum"=w1042:T76)  [unwired: 7 in]
                    n561 = local read "Instr info"() -> (w1036:T8)
                    n562 = call <userlib>:"Write Section Cluster__ogtk.vi"("error in (no error)"=w1043, "Section Formatted Cluster"=w1041, "refnum"=w1042) -> ("error out"=w1038:errorcluster, "dup refnum"=w1040:T76)  [unwired: 7 in]
                    n563 = call <userlib>:"Write Section Cluster__ogtk.vi"("error in (no error)"=w1038, "Section Formatted Cluster"=w1036, "refnum"=w1040) -> ("error out"=w1037:errorcluster, "dup refnum"=w1039:T76)  [unwired: 7 in]
                    n564 = call <vilib>:"Close Config Data.vi"("error in (no error)"=w1037, "refnum"=w1039) -> ()  [unwired: 8 in, 2 out]
                  }
                  frame True {
                  }
                }
                n565 = for {
                  tunnel: w999 -> [w1005] mode=indexing
                  tunnel: w996 -> [w1003]
                  n566 = property class="Ctl"(reference=w1005) -> ("Label.Text"=w1004:string, "Value"=w1002:variant)  [unwired: 1 in, 2 out]
                  n567 = Variant To Data(type=FALSE, Variant=w1002) -> (data=w1000:bool)  [unwired: 1 in, 1 out]
                  n568 = case shown="True" w1000 {
                    tunnel: w1004 -> [_ w1007]
                    tunnel: w1003 -> [_ w1006]
                    frame False {
                    }
                    frame True {
                      n569 = case shown="\"Mag\"" w1007 {
                        tunnel: w1006 -> [w1011 w1012 w1019 w1023 w1027 w1031 w1035 _]
                        frame "Mag" {
                          n570 = Unbundle By Name(w1011) -> ("Field_C"=w1009:refnum<queue>)
                          n571 = call "Put in mailbox.vi"("Priority? (F)"=TRUE ("Priority?"), "Message"=T36 {"Command"=enum."Eval temperatures", "Data"=variant} ("MSG to magnet"), "Queue in"=w1009) -> ()  [unwired: 6 in, 3 out]
                        }
                        frame "SMU" {
                          n572 = Unbundle By Name(w1012) -> ("Mod_M"=w1014:refnum<queue>)
                          n573 = call "Put in mailbox.vi"("Priority? (F)"=TRUE ("Priority?"), "Message"=T37 {"Command"=enum."End", "Data"=variant} ("MSG to Source meter"), "Queue in"=w1014) -> ()  [unwired: 6 in, 3 out]
                        }
                        frame "VTI" {
                          n574 = Unbundle By Name(w1019) -> ("Tmp_C"=w1017:refnum<queue>)
                          n575 = call "Put in mailbox.vi"("Priority? (F)"=TRUE ("Priority?"), "Message"=T50 {"Command"=enum."End", "Data"=variant} ("MSG for VTI"), "Queue in"=w1017) -> ()  [unwired: 6 in, 3 out]
                        }
                        frame "THz" {
                          n576 = Unbundle By Name(w1023) -> ("MW_C"=w1021:refnum<queue>)
                          n577 = call "Put in mailbox.vi"("Priority? (F)"=TRUE ("Priority?"), "Message"=T43 {"Command"=enum."End", "Data"=variant} ("Incoming msg"), "Queue in"=w1021) -> ()  [unwired: 6 in, 3 out]
                        }
                        frame "ACQ" {
                          n578 = Unbundle By Name(w1027) -> ("Data_Aq"=w1025:refnum<queue>)
                          n579 = call "Put in mailbox.vi"("Priority? (F)"=TRUE ("Priority?"), "Message"=T47 {"Command"=enum."End", "Data"=variant} ("MSG for  ACQ"), "Queue in"=w1025) -> ()  [unwired: 6 in, 3 out]
                        }
                        frame "Serv" {
                          n580 = Unbundle By Name(w1031) -> ("Table_C"=w1029:refnum<queue>)
                          n581 = call "Put in mailbox.vi"("Priority? (F)"=TRUE ("Priority?"), "Message"=T40 {"Command"=enum."End", "Data"=variant(dbl[] [])} ("MSG to Servo"), "Queue in"=w1029) -> ()  [unwired: 6 in, 3 out]
                        }
                        frame "Rot" {
                          n582 = Unbundle By Name(w1035) -> ("Angle_C"=w1033:refnum<queue>)
                          n583 = call "Put in mailbox.vi"("Priority? (F)"=TRUE ("Priority?"), "Message"=cluster{"Command":T52, "Data":variant} {"Command"=enum."End", "Data"=variant} ("MSG to rotator"), "Queue in"=w1033) -> ()  [unwired: 6 in, 3 out]
                        }
                        frame "Ignore", Default {
                        }
                      }
                    }
                  }
                }
              }
            }
          }
          event "Re-connect instruments": Value Change {
            n584 = event-data() -> ()  [unwired: 1 in, 6 out]
            n585 = local read "System config file path"() -> (w1069:path)
            n586 = case shown="\"All\", Default" "Select module" {
              tunnel: w1074 -> [w1079 _ w1089 w1118 w1126 w1135 w1137 w1157 w1167]
              tunnel: w1069 -> [w1078 _ _ _ _ _ _ w1151 w1159]
              tunnel: w1073 -> [w1077 w1080 w1090 w1119 w1123 w1136 w1142 w1158 w1168]
              tunnel: [w1077 w1080 w1090 w1119 w1123 w1136 w1142 w1158 w1168] -> w1072
              tunnel: "Use previous settings" -> [_ _ w1081 _ _ _ _ _ _]
              frame "All", Default {
                n587 = call "Send message to initialize all modules.vi"("System config file path"=w1078, "Messenger referencies"=w1079) -> ()  [unwired: 10 in]
                n588 = property on="Select module" class="Enum (strict)"("DisabledEnum"=T32."Enabled" ("Disabled")) -> ()  [unwired: 2 in, 2 out]
              }
              frame "None" {
              }
              frame "ACQ" {
                w1082 = T47 {"Command"=enum."Initialize", "Data"=variant} ("MSG for  ACQ")
                n589 = Unbundle By Name(w1089) -> ("Data_Aq"=w1086:refnum<queue>)
                n590 = Bundle By Name(cluster=w1082, "Command"=MFLI_command_enum."Initialize", "Data"="MF-DEV4029") -> (w1087:T47)
                n591 = call "Put in mailbox.vi"("Priority? (F)"=TRUE, "Message"=w1087, "Queue in"=w1086) -> ("Queue out"=w1083:refnum<queue>)  [unwired: 6 in, 2 out]
                n592 = case shown="True" w1081 {
                  tunnel: w1083 -> [_ w1112]
                  tunnel: w1082 -> [_ w1110]
                  frame False {
                  }
                  frame True {
                    w1099 = T44 {"parameter"=enum."filter_order [-]", "value"=0.0} ("Parameter to set")
                    n593 = local read "Acquisition controls"() -> (w1108:T15)
                    n594 = Unbundle By Name(w1108) -> ("ACQ parameters"=w1095:T14)
                    n595 = Unbundle By Name(w1095) -> ("Filter order"=w1107:dbl, "Filter tau [ms]"=w1106:dbl, "F_Mod [kHz]"=w1105:dbl, "Amp_Mod [mV]"=w1104:dbl)
                    n596 = Divide(x=w1104, y=1000.0) -> (x/y=w1103:dbl)
                    n597 = Bundle(cluster=w1099, "parameter"=MFLI_node."osc_freq [kHz]", "value"=w1105) -> (w1097:T44)
                    n598 = Bundle(cluster=w1099, "parameter"=MFLI_node."filter_constant [ms]", "value"=w1106) -> (w1098:T44)
                    n599 = Bundle(cluster=w1099, "parameter"=MFLI_node."out_ampl [V]", "value"=w1103) -> (w1101:T44)
                    n600 = Bundle(cluster=w1099, "parameter"=MFLI_node."filter_order [-]", "value"=w1107) -> (w1100:T44)
                    n601 = Build Array(w1100, w1098, w1097, w1101) -> (w1096:T44[])
                    n602 = Bundle By Name(cluster=w1110, "Command"=MFLI_command_enum."Set individual parameters", "Data"=w1096) -> (w1111:T47)
                    n603 = call "Put in mailbox.vi"("Message"=w1111, "Queue in"=w1112) -> ()  [unwired: 7 in, 3 out]
                  }
                }
              }
              frame "ROT" {
                n604 = Unbundle By Name(w1118) -> ("Angle_C"=w1114:refnum<queue>)
                n605 = Bundle By Name(cluster=T51 {"Command"=enum."Initialize", "Data"=variant} ("MSG to rotator"), "Command"=Rotator_commands."Initialize", "Data"=path "M:/Instrument/HFEPR spectrometer/Software developement/Separate libraries/Sampe rotator/ANC350/Win64/anc350v4.dll" ("File Path Control")) -> (w1116:T51)
                n606 = disable-structure shown="Disabled" {
                  disable-tunnel: w1116 -> [w1121 _]
                  disable-tunnel: w1114 -> [w1120 _]
                  frame Disabled {
                    n607 = call "Put in mailbox.vi"("Message"=w1121, "Queue in"=w1120) -> ()  [unwired: 7 in, 3 out]
                  }
                  frame Enabled {
                  }
                }
              }
              frame "VTI" {
                n608 = Unbundle By Name(w1126) -> ("Tmp_M"=w1125:refnum<queue>)
                n609 = Bundle By Name(cluster=T50 {"Command"=enum."Initialize", "Data"=variant} ("MSG for VTI"), "Command"=TC_commands."Initialize", "Data"="COM4") -> (w1124:T50)
                n610 = call "Put in mailbox.vi"("Message"=w1124, "Queue in"=w1125) -> ()  [unwired: 7 in, 3 out]
              }
              frame "THz" {
                n611 = Unbundle By Name(w1135) -> ("MW_C"=w1130:refnum<queue>)
                n612 = Bundle By Name(cluster=T55 {"Command"=enum."Initialize", "Data"=variant} ("Incoming msg"), "Command"=THz_commands_enum."Connect", "Data"=T53 {"Master"={"Lower limit [GHz]"=8.0, "Upper limit [GHz]"=20.0, "Name"="VDIS0122", "Handle"="", "Description"="VDI Synth"}, "Follower"={"Lower limit [GHz]"=8.0, "Upper limit [GHz]"=20.0, "Name"="VDIYT7", "Handle"="", "Description"="VDI Tracking"}} ("VDI config constants")) -> (w1133:T55)
                n613 = call "Put in mailbox.vi"("Priority? (F)"=TRUE, "Message"=w1133, "Queue in"=w1130) -> ()  [unwired: 6 in, 3 out]
              }
              frame "SMU" {
                n614 = Unbundle By Name(w1137) -> ("Field_M"=w1138:refnum<queue>)
                n615 = Bundle By Name(cluster=T37 {"Command"=enum."Connect", "Data"=variant} ("MSG to Source meter"), "Data"="USB0::0x05E6::0x2450::04405250::INSTR") -> (w1140:T37)
                n616 = call "Put in mailbox.vi"("Message"=w1140, "Queue in"=w1138) -> ()  [unwired: 7 in, 3 out]
              }
              frame "MAG" {
                n617 = call "Read magnet system configuration.vi"("MAG config file path"=w1151) -> ("error out"=w1153:errorcluster, "Magnet Constantsout"=w1149:T80)  [unwired: 8 in, 1 out]
                n618 = Unbundle By Name(w1157) -> ("Field_C"=w1152:refnum<queue>)
                n619 = Unbundle By Name(w1149) -> ("Maximum field [T]"=w1148:dbl, "Field Constant [T/A]"=w1146:dbl, "Ramp limits [A/s]"=w1147:dbl[])
                n620 = Bundle By Name(cluster=T36 {"Command"=enum."Connect", "Data"=variant(enum16{"Ramping", "Perzistant"} enum."Ramping")} ("MSG to magnet"), "Command"=Magnet_Orders."Connect" ("Order"), "Data"=w1149) -> (w1155:T36)
                n621 = Index Array(array=w1147) -> (element=w1145:dbl)  [unwired: 1 in]
                n622 = call "Put in mailbox.vi"("Priority? (F)"=TRUE, "error in (no error)"=w1153, "Message"=w1155, "Queue in"=w1152) -> ()  [unwired: 5 in, 3 out]
                n623 = Compound Arithmetic op=MULTIPLY(w1146, w1145, 1000.0 ("value")) -> (w1143:dbl)
                n624 = property on="Set Field [T]" class="DigNum (strict)"("Maximum"=w1148) -> ()  [unwired: 2 in, 2 out]
                n625 = property on="Desired ramp\nrate [mT/s]" class="DigNum (strict)"("Maximum"=w1143) -> ()  [unwired: 2 in, 2 out]
              }
              frame "SERV" {
                n626 = Unbundle By Name(w1167) -> ("Table_C"=w1160:refnum<queue>)
                n627 = call "Servo Read system configuration.vi"("MAG config file path"=w1159) -> ("error out"=w1164:errorcluster, "IP addresses"=w1165:string[])  [unwired: 8 in, 1 out]
                n628 = Bundle By Name(cluster=T40 {"Command"=enum."Initialize", "Data"=variant(dbl[] [])} ("MSG to Servo"), "Command"=Servo_commands."Initialize", "Data"=w1165) -> (w1166:T40)
                n629 = call "Put in mailbox.vi"("Priority? (F)"=TRUE, "error in (no error)"=w1164, "Message"=w1166, "Queue in"=w1160) -> ()  [unwired: 5 in, 3 out]
              }
            }
          }
        }
        "Logger" <- w106
        n630 = Index Array(array=w106) -> (element=w111:string)  [unwired: 1 in]
        n631 = Bundle By Name(cluster=w110, "Last log"=w111) -> (w108:T24)
        n632 = local write "Infobar"(w108) -> ()
      }
      frame "Check message" {
        # "actual measurement"
        n633 = Unbundle By Name(w1173) -> ("TOP"=w1190:refnum<queue>)
        n634 = call "Receive message by TOP.vi"("timeout (100)"=10 ("timeout in ms (-1)"), "Mailbox in"=w1190) -> ("error out"=w1183:errorcluster, "timed out?"=w1185:bool, "Unread"=w1182:i32, "MSG packet"=w1189:T81)  [unwired: 6 in]
        n635 = Or(x=w1185, y=w1183) -> (x .or. y?=w1184:bool)
        n636 = case shown="False" w1184 {
          tunnel: w1189 -> [w1212 _]
          tunnel: w1187 -> [w1209 w2212]
          tunnel: [w1208 w2212] -> w1186
          tunnel: w1170 -> [w1203 w2211]
          tunnel: [w1202 w2211] -> w1175
          tunnel: w1174 -> [w1205 _]
          tunnel: w1173 -> [w1204 _]
          tunnel: w1172 -> [w1201 w2210]
          tunnel: [w1200 w2210] -> w1171
          frame False {
            n637 = Unbundle By Name(w1212) -> ("Time"=w1207:timestamp, "Module"=w1211:T82, "Response"=w1210:string, "Data"=w1206:variant)
            n638 = case "Message from module:" shown="\"Magnet\"" w1211 {
              selector: w1211 -> [_ _ _ _ _ _ w2136 w2206]
              tunnel: w1210 -> [w1224 w1480 w1571 w1688 w1832 w1931 w2140 w2204]
              tunnel: w1206 -> [w1223 w1477 w1570 w1689 w1831 w1934 w2139 _]
              tunnel: w1209 -> [w1222 w1479 w1567 w1693 w1830 w1933 w2138 w2209]
              tunnel: [w1221 w1478 w1566 w1692 w1829 w1932 w2137 w2208] -> w1208
              tunnel: w1207 -> [w1220 w1476 w1569 w1694 w1824 w1925 w2129 _]
              tunnel: w1203 -> [w1219 w1474 w1568 w1690 w1822 w1930 w2135 w2202]
              tunnel: [w1218 w1475 w1568 w1691 w1828 w1930 w2135 w2202] -> w1202
              tunnel: w1205 -> [_ w1473 _ _ _ _ _ _]
              tunnel: w1204 -> [w1213 _ _ _ _ _ _ _]
              tunnel: w1201 -> [w1217 w1472 w1562 w1698 w1827 w1929 w2133 w2201]
              tunnel: [w1215 w1470 w1563 w1697 w1826 w1928 w2131 w2201] -> w1200
              frame "Magnet" {
                # "list of responses:"
                n639 = Unbundle By Name(w1217) -> ("Magnet"=w1216:T83)
                n640 = case shown="\"Set field\"" w1224 {
                  selector: w1224 -> [w1231 _ _ _ _ _ _ _ w1385 _ _ _]
                  tunnel: w1223 -> [w1227 w1274 w1288 w1299 w1309 w1331 w1360 w1370 w1389 w1424 w1455 _]
                  tunnel: w1222 -> [w1229 w1271 w1281 w1295 w1306 w1315 w1352 w1365 w1382 w1407 w1456 w1459]
                  tunnel: [w1230 w1254 w1282 w1294 w1305 w1314 w1351 w1366 w1381 w1408 w1456 w1458] -> w1221
                  tunnel: w1220 -> [_ _ _ _ _ w1318 _ _ _ w1399 w1451 _]
                  tunnel: w1219 -> [w1226 w1259 w1280 w1291 w1302 w1321 w1348 w1364 w1380 w1393 w1452 w1461]
                  tunnel: [w1226 w1259 w1280 w1291 w1302 w1320 w1348 w1364 w1380 w1405 w1452 w1461] -> w1218
                  tunnel: w1216 -> [w1225 w1258 w1279 w1289 w1300 w1319 w1347 w1363 w1379 w1403 w1440 w1457]
                  tunnel: [w1225 w1253 w1278 w1289 w1300 w1317 w1347 w1363 w1378 w1398 w1440 w1457] -> w1214
                  tunnel: w1213 -> [_ _ _ _ _ _ _ _ _ w1391 _ _]
                  frame "ignore", Default {
                    n641 = Match Pattern(string=w1231, regular expression="Error") -> (after substring=w1228:string, offset past match=w1233:i32)  [unwired: 1 in, 2 out]
                    n642 = Greater Or Equal To 0?(x=w1233) -> (x >= 0?=w1232:bool)
                    n643 = case shown="True" w1232 {
                      tunnel: w1229 -> [w1237 w1246]
                      tunnel: w1231 -> [w1236 w1245]
                      tunnel: [w1235 w1247] -> w1230
                      tunnel: w1228 -> [_ _]
                      tunnel: w1227 -> [_ w1243]
                      frame False {
                        n644 = call "simple Shift string array.vi"("Element in"=w1236, "Array in"=w1237) -> ("Array out"=w1235:string[])  [unwired: 8 in, 1 out]
                      }
                      frame True {
                        n645 = Variant To Data(type=errorcluster {"status"=FALSE, "code"=0, "source"=""} ("error constant"), Variant=w1243) -> (data=w1241:errorcluster)  [unwired: 1 in, 1 out]
                        n646 = Unbundle By Name(w1241) -> ("source"=w1240:string)
                        n647 = call <vilib>:"Space Constant.vi"() -> ("String"=w1244:string)
                        n648 = Concatenate Strings(w1245, w1244, w1240) -> (w1238:string)
                        n649 = local read "loggersRef"() -> (w1239:refnum<file>)
                        n650 = call "Write in logger.vi"("String in"=w1238, "logger refnum"=w1239) -> ()  [unwired: 2 in, 2 out]
                        n651 = call "simple Shift string array.vi"("Element in"=w1238, "Array in"=w1246) -> ("Array out"=w1247:string[])  [unwired: 8 in, 1 out]
                      }
                    }
                  }
                  frame "Initialize" {
                    w1266 = TRUE ("PSU")
                    w1265 = T32."Enabled" ("Disabled")
                    n652 = Variant To Data(type="", Variant=w1274) -> (data=w1248:string)  [unwired: 1 in, 1 out]
                    n653 = local read "Instr status"() -> (w1269:T1)
                    n654 = Bundle By Name(cluster=w1269, "Mag"=w1266) -> (w1273:T1)
                    n655 = Match Pattern(string=w1248, regular expression="SMS120") -> (match substring=w1251:string)  [unwired: 1 in, 3 out]
                    n656 = Unbundle By Name(w1269) -> ("THz"=w1268:bool, "MFLI"=w1267:bool)
                    n657 = local write "Instr status"(w1273) -> ()
                    n658 = control-ref of="Magnet controls"() -> (w1270:refnum<vi>)
                    n659 = Compound Arithmetic op=AND(w1268, w1267, w1266) -> (w1264:bool)
                    n660 = call "Add actual date time to string.vi"("String in"="Magnet module initialized") -> ("String out"=w1262:string)  [unwired: 4 in]
                    n661 = Select(t=w1265, s=w1264, f=T32."Disabled and Grayed Out" ("Disabled")) -> (s? t:f=w1260:T32)
                    n662 = local read "loggersRef"() -> (w1261:refnum<file>)
                    n663 = property class="Clust (strict)"(reference=w1270, "DisabledEnum"=w1265) -> ()  [unwired: 1 in, 2 out]
                    n664 = Concatenate Strings(w1262, "\r\n", w1248) -> (w1250:string)
                    n665 = call "simple Shift string array.vi"("Element in"=w1262, "Array in"=w1271) -> ("Array out"=w1255:string[])  [unwired: 8 in, 1 out]
                    n666 = call "Write in logger.vi"("String in"=w1250, "logger refnum"=w1261) -> ()  [unwired: 2 in, 2 out]
                    n667 = call "Add actual date time to string.vi"("String in"=w1248) -> ("String out"=w1256:string)  [unwired: 4 in]
                    n668 = call "simple Shift string array.vi"("Element in"=w1256, "Array in"=w1255) -> ("Array out"=w1254:string[])  [unwired: 8 in, 1 out]
                    n669 = property on="Run MAP btn" class="Bool (strict)"("DisabledEnum"=w1260) -> ()  [unwired: 2 in, 2 out]
                    n670 = Bundle By Name(cluster=w1258, "PSU"=w1251) -> (w1253:T83)
                  }
                  frame "TM revision" {
                    n671 = Variant To Data(type=T57 {"Instr Serial Number"="", "Instr Driver Revision"="", "Instr Firmware Revision"="", "Instr Model Number"=""} ("TM Revision"), Variant=w1288) -> (data=w1286:T57)  [unwired: 1 in, 1 out]
                    n672 = Unbundle By Name(w1286) -> ("Instr Model Number"=w1277:string)
                    n673 = call <vilib>:"Space Constant.vi"() -> ("String"=w1284:string)
                    n674 = Concatenate Strings("Temperature monitor:" ("string"), w1284, w1277) -> (w1283:string)
                    n675 = Bundle By Name(cluster=w1279, "T monitor"=w1277) -> (w1278:T83)
                    n676 = call "Add actual date time to string.vi"("String in"=w1283) -> ("String out"=w1275:string)  [unwired: 4 in]
                    n677 = local read "loggersRef"() -> (w1276:refnum<file>)
                    n678 = call "simple Shift string array.vi"("Element in"=w1275, "Array in"=w1281) -> ("Array out"=w1282:string[])  [unwired: 8 in, 1 out]
                    n679 = call "Write in logger.vi"("String in"=w1275, "logger refnum"=w1276) -> ()  [unwired: 2 in, 2 out]
                  }
                  frame "Initialization error" {
                    n680 = Variant To Data(type=errorcluster {"status"=FALSE, "code"=0, "source"=""} ("error constant"), Variant=w1299) -> (data=w1297:errorcluster, error out=w1290:errorcluster)  [unwired: 1 in]
                    n681 = Unbundle By Name(w1297) -> ("source"=w1296:string)
                    n682 = call "Add actual date time to string.vi"("String in"=w1296) -> ("String out"=w1293:string)  [unwired: 4 in]
                    n683 = call "simple Shift string array.vi"("Element in"=w1293, "Array in"=w1295) -> ("Array out"=w1294:string[])  [unwired: 8 in, 1 out]
                    n684 = local read "loggersRef"() -> (w1292:refnum<file>)
                    n685 = call "Write in logger.vi"("error in"=w1290, "String in"=w1293, "logger refnum"=w1292) -> ()  [unwired: 1 in, 2 out]
                  }
                  frame "Flip polarity" {
                    n686 = Variant To Data(type="" ("error constant"), Variant=w1309) -> (data=w1307:string, error out=w1301:errorcluster)  [unwired: 1 in]
                    n687 = call "Add actual date time to string.vi"("String in"=w1307) -> ("String out"=w1304:string)  [unwired: 4 in]
                    n688 = call "simple Shift string array.vi"("Element in"=w1304, "Array in"=w1306) -> ("Array out"=w1305:string[])  [unwired: 8 in, 1 out]
                    n689 = local read "loggersRef"() -> (w1303:refnum<file>)
                    n690 = call "Write in logger.vi"("error in"=w1301, "String in"=w1304, "logger refnum"=w1303) -> ()  [unwired: 1 in, 2 out]
                  }
                  frame "Update" {
                    n691 = Variant To Data(type=T58 {"Desired"={"Field [T]"=0.0, "Ramp [T/s]"=0.0, "Custom Ramp?"=TRUE, "Mode"=enum."Persistant"}, "Actual"={"Mode"=enum."Persistant", "Ramping output"=enum."At Target", "Ready for change"=FALSE, "Switch heater"=FALSE, "Cooler Overheat"=FALSE, "Coil overheat"=FALSE, "Energized"=FALSE, "Output [T]"=0.0, "Field [T]"=0.0, "Ramp[T/s]"=0.0, "Switch\ntemperature [K]"=1.0, "Voltage [V]"=0.0, "Current direction"=FALSE}} ("output cluster"), Variant=w1331) -> (data=w1313:T58)  [unwired: 1 in, 1 out]
                    n692 = Unbundle By Name(w1313) -> ("Actual.Ready for change"=w1310:bool, "Actual.Mode"=w1311:T60, "Actual.Field [T]"=w1312:dbl)
                    n693 = local read "Instr status"() -> (w1329:T1)
                    n694 = local read "Magnet controls"() -> (w1324:T18)
                    n695 = Bundle By Name(cluster=w1329, "Mag"=TRUE ("PSU")) -> (w1328:T1)
                    n696 = Bundle By Name(cluster=w1321, "Field [T]"=w1312) -> (w1320:T24)
                    n697 = local write "Instr status"(w1328) -> ()
                    n698 = call "Magnet update rewiring.vi"("output cluster"=w1313, "Time"=w1318, "Magnet in"=w1319, "Magnet controls in"=w1324) -> ("Magnet out"=w1317:T83, "Magnet controls out"=w1323:T18)  [unwired: 6 in]
                    n699 = local write "Magnet controls"(w1323) -> ()
                    n700 = case shown="\"Quenched\"" w1311 {
                      selector: w1311 -> [_ _ _ w1340]
                      tunnel: [w1333 w1334 w1337 w1342] -> w1314
                      tunnel: w1315 -> [w1333 w1334 w1337 w1341]
                      tunnel: [T32."Enabled" ("Disabled") T32."Disabled and Grayed Out" ("f") T32."Disabled and Grayed Out" ("f") T32."Disabled and Grayed Out" ("f")] -> w1316
                      frame "Persistant", Default {
                      }
                      frame "Switching" {
                      }
                      frame "Ramping" {
                      }
                      frame "Quenched" {
                        n701 = Format Into String(w1340) -> (resulting string=w1339:string)  [unwired: 3 in, 1 out]
                        n702 = call "Add actual date time to string.vi"("String in"=w1339) -> ("String out"=w1343:string)  [unwired: 4 in]
                        n703 = local read "loggersRef"() -> (w1344:refnum<file>)
                        n704 = call "simple Shift string array.vi"("Element in"=w1343, "Array in"=w1341) -> ("Array out"=w1342:string[])  [unwired: 8 in, 1 out]
                        n705 = call "Write in logger.vi"("String in"=w1343, "logger refnum"=w1344) -> ()  [unwired: 2 in, 2 out]
                      }
                    }
                    n706 = Select(t=T32."Enabled" ("Disabled"), s=w1310, f=T32."Disabled and Grayed Out") -> (s? t:f=w1322:T32)
                    n707 = property on="Mode switch" class="Bool (strict)"("DisabledEnum"=w1322) -> ()  [unwired: 2 in, 2 out]
                    n708 = property on="Equalize" class="Bool (strict)"("DisabledEnum"=w1316) -> ()  [unwired: 2 in, 2 out]
                    n709 = property on="Discharge" class="Bool (strict)"("DisabledEnum"=w1316) -> ()  [unwired: 2 in, 2 out]
                  }
                  frame "Update error" {
                    # "ReInitialize Magnet?"
                    n710 = Variant To Data(type=errorcluster {"status"=FALSE, "code"=0, "source"=""} ("error in (no error)"), Variant=w1360) -> (data=w1358:errorcluster)  [unwired: 1 in, 1 out]
                    n711 = Unbundle By Name(w1358) -> ("source"=w1355:string)
                    n712 = local read "Instr status"() -> (w1354:T1)
                    n713 = Bundle By Name(cluster=w1354, "Mag"=FALSE ("PSU")) -> (w1353:T1)
                    n714 = local write "Instr status"(w1353) -> ()
                    n715 = Concatenate Strings("Magnet Update error: " ("String in"), w1355) -> (w1356:string)
                    n716 = property on="Magnet controls" class="Clust (strict)"("DisabledEnum"=T32."Disabled and Grayed Out" ("Disabled")) -> ()  [unwired: 2 in, 2 out]
                    n717 = local read "loggersRef"() -> (w1346:refnum<file>)
                    n718 = call "Add actual date time to string.vi"("String in"=w1356) -> ("String out"=w1345:string)  [unwired: 4 in]
                    n719 = call "Write in logger.vi"("String in"=w1345, "logger refnum"=w1346) -> ()  [unwired: 2 in, 2 out]
                    n720 = call "simple Shift string array.vi"("Element in"=w1345, "Array in"=w1352) -> ("Array out"=w1351:string[])  [unwired: 8 in, 1 out]
                  }
                  frame "Switch mode acepted" {
                    n721 = Variant To Data(type=Magnet_mode_public."Ramping" ("Operation mode"), Variant=w1370) -> (data=w1368:T33)  [unwired: 1 in, 1 out]
                    n722 = case shown="\"Persistant\"" w1368 {
                      tunnel: ["Switching to ramping mode" "Switching to perzistant mode"] -> w1367
                      frame "Ramping", Default {
                      }
                      frame "Persistant" {
                      }
                    }
                    n723 = call "Add actual date time to string.vi"("String in"=w1367) -> ("String out"=w1361:string)  [unwired: 4 in]
                    n724 = local read "loggersRef"() -> (w1362:refnum<file>)
                    n725 = call "simple Shift string array.vi"("Element in"=w1361, "Array in"=w1365) -> ("Array out"=w1366:string[])  [unwired: 8 in, 1 out]
                    n726 = call "Write in logger.vi"("String in"=w1361, "logger refnum"=w1362) -> ()  [unwired: 2 in, 2 out]
                  }
                  frame "Ramping" {
                    n727 = Variant To Data(type=T34 {"Field [T]"=0.0, "Ramp [T/s]"=0.0, "Custom Ramp?"=TRUE, "Mode"=enum."Persistant"} ("Set Field"), Variant=w1389) -> (data=w1387:T34)  [unwired: 1 in, 1 out]
                    n728 = Unbundle By Name(w1387) -> ("Field [T]"=w1384:dbl, "Ramp [T/s]"=w1376:dbl)
                    n729 = Multiply(x=w1376, y=1000.0) -> (x*y=w1375:dbl)
                    n730 = Bundle By Name(cluster=w1379, "Ramp [mT/s]"=w1375) -> (w1378:T83)
                    n731 = Format Into String(format string=" B= %f [T] Ramp= %f [mT/s]", initial string=w1385, w1384, w1375) -> (resulting string=w1383:string)  [unwired: 1 in, 1 out]
                    n732 = call "Add actual date time to string.vi"("String in"=w1383) -> ("String out"=w1373:string)  [unwired: 4 in]
                    n733 = local read "loggersRef"() -> (w1374:refnum<file>)
                    n734 = call "simple Shift string array.vi"("Element in"=w1373, "Array in"=w1382) -> ("Array out"=w1381:string[])  [unwired: 8 in, 1 out]
                    n735 = call "Write in logger.vi"("String in"=w1373, "logger refnum"=w1374) -> ()  [unwired: 2 in, 2 out]
                  }
                  frame "Set field" {
                    n736 = Unbundle By Name(w1393) -> ("Experiment state"=w1406:T25)
                    n737 = Unbundle By Name(w1391) -> ("Data_Aq"=w1390:refnum<queue>)
                    n738 = local read "Magnet controls"() -> (w1422:T18)
                    n739 = Variant To Data(type=T34 {"Field [T]"=0.0, "Ramp [T/s]"=0.0, "Custom Ramp?"=TRUE, "Mode"=enum."Persistant"} ("Set Field"), Variant=w1424) -> (data=w1421:T34, error out=w1394:errorcluster)  [unwired: 1 in]
                    n740 = Unbundle By Name(w1403) -> ("Field [T]"=w1410:dbl)
                    n741 = case shown="\"Begin\"" w1406 {
                      selector: w1406 -> [w1426 _]
                      tunnel: [w1426 experiment_state."Acquisition" ("Value")] -> w1404
                      tunnel: w1399 -> [_ w1434]
                      tunnel: w1393 -> [w1425 w1432]
                      tunnel: [w1425 w1433] -> w1392
                      tunnel: w1390 -> [_ w1427]
                      frame "Setup", Default {
                      }
                      frame "Begin" {
                        n742 = Bundle By Name(cluster=w1432, "Started"=w1434) -> (w1433:T24)
                        n743 = Build Array(T44 {"parameter"=enum."scope_trigEn", "value"=1.0} ("Parameter to set")) -> (w1431:T44[])
                        n744 = Bundle By Name(cluster=T47 {"Command"=enum."Set individual parameters", "Data"=variant} ("MSG for  ACQ"), "Data"=w1431) -> (w1428:T47)
                        n745 = call "Put in mailbox.vi"("Message"=w1428, "Queue in"=w1427) -> ()  [unwired: 7 in, 3 out]
                      }
                    }
                    n746 = Unbundle By Name(w1421) -> ("Field [T]"=w1415:dbl, "Ramp [T/s]"=w1402:dbl, "Custom Ramp?"=w1420:bool)
                    n747 = Unbundle By Name(w1422) -> ("Desired ramp\nrate [mT/s]"=w1419:dbl)
                    n748 = Not(x=w1420) -> (.not. x?=w1418:bool)
                    n749 = call <userlib>:"MGI Approximately Equal.vi"("Numeric 2"=w1419, "Numeric 1"=w1402) -> ("approx = ?"=w1417:bool)
                    n750 = Multiply(x=w1402, y=1000.0 ("x")) -> (x*y=w1400:dbl)
                    n751 = Or(x=w1418, y=w1417) -> (x .or. y?=w1414:bool)
                    n752 = case shown="False" w1414 {
                      tunnel: ["Warning: Custom ramp was adjusted" ""] -> w1412
                      frame False {
                      }
                      frame True {
                      }
                    }
                    n753 = Format Into String(format string="Setting magnetic field from %f [T ] to %f [T] with ramp %f [mT/s]", error in=w1394, w1410, w1415, w1400) -> (resulting string=w1413:string, error out=w1395:errorcluster)  [unwired: 1 in]
                    n754 = Concatenate Strings(w1413, "\r", w1412) -> (w1396:string)
                    n755 = call "Add actual date time to string.vi"("String in"=w1396) -> ("String out"=w1409:string)  [unwired: 4 in]
                    n756 = local read "loggersRef"() -> (w1397:refnum<file>)
                    n757 = Bundle By Name(cluster=w1403, "Last update"=w1399, "Ramp [mT/s]"=w1400) -> (w1398:T83)
                    n758 = Bundle By Name(cluster=w1392, "Experiment state"=w1404) -> (w1405:T24)
                    n759 = call "simple Shift string array.vi"("Element in"=w1409, "Array in"=w1407) -> ("Array out"=w1408:string[])  [unwired: 8 in, 1 out]
                    n760 = call "Write in logger.vi"("error in"=w1395, "String in"=w1396, "logger refnum"=w1397) -> ()  [unwired: 1 in, 2 out]
                  }
                  frame "Temperatures" {
                    n761 = Variant To Data(type=T61 {"First stage A [K]"=0.0, "Second stage A [K]"=0.0, "Firs stage B [K]"=0.0, "Second stage B [K]"=0.0, "Inner magnet [K]"=0.0, "Outer Magnet [K]"=0.0, "Switch [K]"=0.0, "Support plate [K]"=0.0, "Time stamp"=0.0} ("LSC218 sensors"), Variant=w1455) -> (data=w1444:T61)  [unwired: 1 in, 1 out]
                    n762 = Unbundle By Name(w1440) -> ("Field [T]"=w1439:dbl)
                    n763 = property on="VTI" class="Clust (strict)"() -> ("Value"=w1450:T84)  [unwired: 2 in, 2 out]
                    n764 = local read "Temperature log ref"() -> (w1453:refnum<file>)
                    n765 = Cluster To Array(cluster=w1444) -> (array=w1447:dbl[])
                    n766 = Unbundle By Name(w1450) -> ("VTI [K]"=w1442:dbl, "Sample [K]"=w1441:dbl, "Trap[K]"=w1449:dbl, "HePot [K]"=w1448:dbl)
                    n767 = call "Bundle temperatures.vi"("Sample"=w1441, "VTI space"=w1442, "LSC218 sensors"=w1444) -> ("Tmp [K]"=→"Tmp [K]":T3)  [unwired: 8 in]
                    n768 = Build Array (concatenate)(w1447, w1442, w1441, w1449, w1448) -> (w1446:dbl[])
                    n769 = call "Log temperatures.vi"("LSC218 sensors"=w1444, "Time"=w1451, "Tmp logfile in"=w1453, "VTI"=w1442, "Sample"=w1441, "Trap"=w1449, "HePot"=w1448, "Field [T]"=w1439) -> ("Tmp logfile ref"=w1438:refnum<file>)  [unwired: 5 in, 2 out]
                    n770 = Array To Cluster(array=w1446) -> (cluster=→"Temperature monitor":T12)
                    n771 = local write "Temperature log ref"(w1438) -> ()
                  }
                  frame "End" {
                    n772 = local read "loggersRef"() -> (w1463:refnum<file>)
                    n773 = local read "Instr status"() -> (w1467:T1)
                    n774 = call "Add actual date time to string.vi"("String in"="Magnet dissconnected") -> ("String out"=w1460:string)  [unwired: 4 in]
                    n775 = Bundle By Name(cluster=w1467, "Mag"=FALSE ("PSU")) -> (w1468:T1)
                    n776 = call "Write in logger.vi"("String in"=w1460, "logger refnum"=w1463) -> ()  [unwired: 2 in, 2 out]
                    n777 = local write "Instr status"(w1468) -> ()
                    n778 = control-ref of="Magnet controls"() -> (w1465:refnum<vi>)
                    n779 = call "simple Shift string array.vi"("Element in"=w1460, "Array in"=w1459) -> ("Array out"=w1458:string[])  [unwired: 8 in, 1 out]
                    n780 = property class="Clust (strict)"(reference=w1465, "DisabledEnum"=T32."Disabled and Grayed Out" ("Disabled")) -> ()  [unwired: 1 in, 2 out]
                  }
                }
                n781 = Bundle By Name(cluster=w1217, "Magnet"=w1214) -> (w1215:T26)
              }
              frame "Excitation" {
                n782 = Unbundle By Name(w1472) -> ("THz"=w1471:T85)
                n783 = case shown="\"Set parameters\"" w1480 {
                  selector: w1480 -> [_ w1498 _ _ _]
                  tunnel: w1479 -> [w1483 w1513 w1516 w1544 w1550]
                  tunnel: [w1483 w1512 w1516 w1545 w1551] -> w1478
                  tunnel: w1477 -> [_ w1499 _ w1543 w1552]
                  tunnel: w1476 -> [_ _ _ w1521 w1554]
                  tunnel: w1474 -> [w1482 w1497 w1515 w1517 w1558]
                  tunnel: [w1482 w1497 w1515 w1517 w1558] -> w1475
                  tunnel: w1473 -> [_ _ _ _ _]
                  tunnel: w1471 -> [w1481 w1490 w1514 w1523 w1557]
                  tunnel: [w1481 w1489 w1514 w1522 w1556] -> w1469
                  frame "Ignore", Default {
                  }
                  frame "Initialize" {
                    w1485 = T32."Disabled and Grayed Out" ("Disabled")
                    w1484 = T32."Enabled" ("Disabled")
                    n784 = Variant To Data(type=w1498, Variant=w1499) -> (data=w1496:string, error out=w1486:errorcluster)  [unwired: 1 in]
                    n785 = Match Pattern(string=w1496, regular expression="VDI Synth") -> (after substring=w1488:string, offset past match=w1511:i32)  [unwired: 1 in, 2 out]
                    n786 = Match Pattern(string=w1496, regular expression="VDI Tracking") -> (after substring=w1487:string, offset past match=w1508:i32)  [unwired: 1 in, 2 out]
                    n787 = Greater Or Equal To 0?(x=w1508) -> (x >= 0?=w1494:bool)
                    n788 = Greater Or Equal To 0?(x=w1511) -> (x >= 0?=w1502:bool)
                    n789 = Bundle By Name(cluster=w1490, "Name"=w1488, "Description"=w1487) -> (w1489:T85)
                    n790 = Select(t=T32."Enabled", s=w1494, f=w1485) -> ()  [unwired: 1 out]
                    n791 = local read "Instr status"() -> (w1506:T1)
                    n792 = Bundle By Name(cluster=w1506, "THz"=w1502) -> (w1507:T1)
                    n793 = Unbundle By Name(w1506) -> ("Mag"=w1505:bool, "MFLI"=w1504:bool)
                    n794 = local write "Instr status"(w1507) -> ()
                    n795 = Compound Arithmetic op=AND(w1505, w1504, w1502) -> (w1503:bool)
                    n796 = Select(t=w1484, s=w1503, f=w1485) -> (s? t:f=w1500:T32)
                    n797 = local read "loggersRef"() -> (w1501:refnum<file>)
                    n798 = property on="VID control" class="Clust (strict)"("DisabledEnum"=w1484) -> ()  [unwired: 2 in, 2 out]
                    n799 = property on="Run MAP btn" class="Bool (strict)"(error in=w1486, "DisabledEnum"=w1500) -> (error out=w1492:errorcluster)  [unwired: 1 in, 1 out]
                    n800 = call "Add actual date time to string.vi"("String in"=w1496) -> ("String out"=w1495:string)  [unwired: 4 in]
                    n801 = call "Write in logger.vi"("error in"=w1492, "String in"=w1495, "logger refnum"=w1501) -> ("error out"=w1491:errorcluster)  [unwired: 1 in, 1 out]
                    n802 = call "simple Shift string array.vi"("Element in"=w1496, "Array in"=w1513) -> ("Array out"=w1512:string[])  [unwired: 8 in, 1 out]
                    n803 = call <vilib>:"Clear Errors.vi"("error in (no error)"=w1491) -> ()  [unwired: 5 in, 2 out]
                  }
                  frame "Update" {
                  }
                  frame "Set parameters" {
                    n804 = Variant To Data(type=T42 {"Start [GHz]"=8.0, "End [GHz] "=8.0, "Sweep up\ntime [ms]"=0.0, "Sweep down\ntime [ms]"=0.0, "Intermidiate [MHz]"=0.0, "Reset trigger"=FALSE} ("Sweep parameters"), Variant=w1543) -> (data=w1532:T42, error out=w1533:errorcluster)  [unwired: 1 in]
                    n805 = local read "VID control"() -> (w1539:T16)
                    n806 = Unbundle By Name(w1532) -> ("Start [GHz]"=w1529:dbl, "End [GHz]"=w1528:dbl, "Sweep up\ntime [ms]"=w1527:dbl, "Intermidiate [MHz]"=w1531:dbl)
                    n807 = Unbundle By Name(w1539) -> ("AMC"=w1540:u16, "Multip"=w1541:u16)
                    n808 = Multiply(x=w1540, y=w1541) -> (x*y=w1530:u16)
                    n809 = Multiply(x=w1529, y=w1530) -> (x*y=w1520:dbl)
                    n810 = Multiply(x=w1528, y=w1530) -> (x*y=w1519:dbl)
                    n811 = Multiply(x=w1527, y=w1530) -> (x*y=w1526:dbl)
                    n812 = Multiply(x=w1531, y=w1530) -> (x*y=w1518:dbl)
                    n813 = Equal To 0?(x=w1526) -> (x = 0?=w1537:bool)
                    n814 = Select(t="CW", s=w1537, f="Sweep") -> (s? t:f=w1534:string)
                    n815 = Format Into String(format string="VDI set to %s mode at %f GHz ", error in=w1533, w1534, w1520) -> (resulting string=w1525:string)  [unwired: 1 in, 1 out]
                    n816 = Bundle By Name(cluster=w1523, "Last update"=w1521, "Start [GHz]"=w1520, "End [GHz]"=w1519, "Im Freq[MHz]"=w1518) -> (w1522:T85)
                    n817 = call "Add actual date time to string.vi"("String in"=w1525) -> ("String out"=w1524:string)  [unwired: 4 in]
                    n818 = call "simple Shift string array.vi"("Element in"=w1524, "Array in"=w1544) -> ("Array out"=w1545:string[])  [unwired: 8 in, 1 out]
                  }
                  frame "End" {
                    w1555 = "None" ("Master")
                    n819 = Variant To Data(type="", Variant=w1552) -> (data=w1547:string)  [unwired: 1 in, 1 out]
                    n820 = Bundle By Name(cluster=w1557, "Name"=w1555, "Description"=w1555, "Last update"=w1554) -> (w1556:T85)
                    n821 = property on="THz" class="Bool (strict)"("Value"=FALSE) -> ()  [unwired: 2 in, 2 out]
                    n822 = call "Add actual date time to string.vi"("String in"="Excitation module (VDI) ended") -> ("String out"=w1549:string)  [unwired: 4 in]
                    n823 = Concatenate Strings(w1549, "\r\n", w1547) -> (w1548:string)
                    n824 = local read "loggersRef"() -> (w1560:refnum<file>)
                    n825 = call "Write in logger.vi"("String in"=w1548, "logger refnum"=w1560) -> ()  [unwired: 2 in, 2 out]
                    n826 = call "simple Shift string array.vi"("Element in"=w1548, "Array in"=w1550) -> ("Array out"=w1551:string[])  [unwired: 8 in, 1 out]
                  }
                }
                n827 = Bundle By Name(cluster=w1472, "THz"=w1469) -> (w1470:T26)
              }
              frame "Acquisition" {
                n828 = Unbundle By Name(w1562) -> ("ACQ"=w1565:T86)
                n829 = case shown="\"Get ModA\"" w1571 {
                  tunnel: w1570 -> [w1596 w1612 w1633 w1652 w1662 w1675 w1685 _]
                  tunnel: w1569 -> [w1575 w1604 w1627 w1649 w1657 _ _ _]
                  tunnel: [w1580 w1608 w1632 w1642 w1663 w1676 w1679 w1687] -> w1566
                  tunnel: w1567 -> [w1581 w1609 w1632 w1642 w1663 w1676 w1680 w1687]
                  tunnel: w1565 -> [w1576 w1605 w1630 w1640 w1659 w1671 w1677 w1686]
                  tunnel: [w1573 w1599 w1628 w1640 w1659 w1671 w1677 w1686] -> w1564
                  frame "Initialize" {
                    w1588 = TRUE ("PSU")
                    w1587 = T32."Enabled" ("Disabled")
                    n830 = Variant To Data(type="", Variant=w1596) -> (data=w1574:string)  [unwired: 1 in, 1 out]
                    n831 = Bundle By Name(cluster=w1576, "Last update"=w1575, "Lock-in"=w1574, "Multimeter"="Unknown") -> (w1573:T86)
                    n832 = local read "Instr status"() -> (w1591:T1)
                    n833 = Bundle By Name(cluster=w1591, "MFLI"=w1588) -> (w1593:T1)
                    n834 = Unbundle By Name(w1591) -> ("THz"=w1590:bool, "Mag"=w1589:bool)
                    n835 = local write "Instr status"(w1593) -> ()
                    n836 = control-ref of="Acquisition controls"() -> (w1592:refnum<vi>)
                    n837 = Compound Arithmetic op=AND(w1590, w1589, w1588) -> (w1586:bool)
                    n838 = Concatenate Strings(w1574, " connected as ACQ" ("String in")) -> (w1578:string)
                    n839 = Select(t=w1587, s=w1586, f=T32."Disabled and Grayed Out" ("Disabled")) -> (s? t:f=w1582:T32)
                    n840 = property class="Clust (strict)"(reference=w1592, "DisabledEnum"=w1587) -> ()  [unwired: 1 in, 2 out]
                    n841 = local read "loggersRef"() -> (w1585:refnum<file>)
                    n842 = control-ref of="Run MAP btn"() -> (w1584:refnum<vi>)
                    n843 = call "Add actual date time to string.vi"("String in"=w1578) -> ("String out"=w1577:string)  [unwired: 4 in]
                    n844 = Build Array(w1584) -> (w1583:refnum<vi>[])
                    n845 = call "Write in logger.vi"("String in"=w1577, "logger refnum"=w1585) -> ()  [unwired: 2 in, 2 out]
                    n846 = call "Dis- or en- able controls.vi"("Disabled"=w1582, "Control referencies"=w1583) -> ()  [unwired: 9 in, 1 out]
                    n847 = call "simple Shift string array.vi"("Element in"=w1577, "Array in"=w1581) -> ("Array out"=w1580:string[])  [unwired: 8 in, 1 out]
                  }
                  frame "Set parameters" {
                    n848 = Variant To Data(type=T14 {"Filter order"=1.0, "Filter tau [ms]"=1.0, "F_Mod [kHz]"=0.0, "Amp_Mod [mV]"=0.0, "Enable output"=0, "Phase [°]"=0.0} ("ACQ parameters"), Variant=w1612) -> (data=w1597:T14)  [unwired: 1 in, 1 out]
                    n849 = local read "Acquisition controls"() -> (w1598:T15)
                    n850 = Unbundle By Name(w1597) -> ("F_Mod [kHz]"=w1603:dbl, "Amp_Mod [mV]"=w1602:dbl, "Enable output"=w1601:u16)
                    n851 = property on="ACQ parameters" class="Clust (strict)"("Value"=w1597) -> ()  [unwired: 2 in, 2 out]
                    n852 = Bundle By Name(cluster=w1598, "ACQ parameters"=w1597) -> (w1610:T15)
                    n853 = Greater Or Equal To 0?(x=w1601) -> (x >= 0?=w1600:bool)
                    n854 = local write "Acquisition controls"(w1610) -> ()
                    n855 = call "Add actual date time to string.vi"("String in"="Lock-in: parameters set" ("Element in")) -> ("String out"=w1606:string)  [unwired: 4 in]
                    n856 = call "simple Shift string array.vi"("Element in"=w1606, "Array in"=w1609) -> ("Array out"=w1608:string[])  [unwired: 8 in, 1 out]
                    n857 = Bundle By Name(cluster=w1605, "Last update"=w1604, "Freq [kHz]"=w1603, "Ampl [mV]"=w1602, "OutEn"=w1600) -> (w1599:T86)
                  }
                  frame "Update" {
                    w1624 = 1000.0 ("x")
                    n858 = Variant To Data(type=T62 {"In50"=FALSE, "InAC"=FALSE, "InDiff"=FALSE, "Out50"=FALSE, "OutEN"=FALSE, "OutF[Hz]"=0.0, "OutA[V]"=0.0, "DemEN"=FALSE, "Const[ms]"=0.0, "Order[-]"=0, "Phase [°]"=0.0} ("Lock-in info"), Variant=w1633) -> (data=w1629:T62)  [unwired: 1 in, 1 out]
                    n859 = Unbundle By Name(w1629) -> ("OutF[Hz]"=w1626:dbl, "OutA[V]"=w1625:dbl, "OutEN"=w1620:bool, "Out50"=w1617:bool, "In50"=w1614:bool, "Order[-]"=w1616:i32, "Const[ms]"=w1615:dbl, "DemEN"=w1613:bool)
                    n860 = Divide(x=w1626, y=w1624) -> (x/y=w1619:dbl)
                    n861 = Multiply(x=w1625, y=w1624) -> (x*y=w1618:dbl)
                    n862 = Boolean To (0,1)(Boolean=w1620) -> (0, 1=w1621:i16)
                    n863 = local read "Acquisition controls"() -> (w1623:T15)
                    n864 = Bundle By Name(cluster=w1623, "ACQ parameters.Enable output"=w1621, "ACQ parameters.F_Mod [kHz]"=w1619, "ACQ parameters.Amp_Mod [mV]"=w1618, "Out50"=w1617, "In50"=w1614, "ACQ parameters.Filter order"=w1616, "ACQ parameters.Filter tau [ms]"=w1615, "DemEn"=w1613) -> (w1622:T15)
                    n865 = Bundle By Name(cluster=w1630, "Last update"=w1627, "Freq [kHz]"=w1619, "Ampl [mV]"=w1618, "OutEn"=w1620, "In50 Ohm"=w1614, "DemEn"=w1613) -> (w1628:T86)
                    n866 = local write "Acquisition controls"(w1622) -> ()
                  }
                  frame "Get point" {
                    n867 = local read "Acquisition controls"() -> (w1644:T15)
                    n868 = local read "Tab Control"() -> (w1647:T6)
                    n869 = Unbundle By Name(w1644) -> ("ACQ shot btn"=w1643:bool)
                    n870 = Variant To Data(type=T64 {"Timestamps (ticks)"=0, "X (Vrms)"=0.0, "Y (Vrms)"=0.0, "Osc Phase (deg)"=0.0, "Freq (Hz)"=0.0, "DIO"=0, "AuxIn0 (V)"=0.0, "AuxIn1 (V)"=0.0, "Trigger"=0} ("Update data"), Variant=w1652) -> (data=w1650:T64)  [unwired: 1 in, 1 out]
                    n871 = Unbundle By Name(w1650) -> ("X (Vrms)"=w1636:dbl, "Y (Vrms)"=w1637:dbl)
                    n872 = Equal?(x=w1647, y=T63."Adjustment" ("Tab Control")) -> (x = y?=w1646:bool)
                    n873 = And(x=w1646, y=w1643) -> (x .and. y?=w1645:bool)
                    n874 = case shown="True" w1645 {
                      tunnel: w1636 -> [_ w1655]
                      tunnel: w1637 -> [_ w1654]
                      frame False {
                      }
                      frame True {
                        n875 = Bundle("X (Vrms)"=w1655, "Y (Vrms)"=w1654) -> (→"lookup":cluster{"X (Vrms)":dbl, "Y (Vrms)":dbl})  [unwired: 1 in]
                      }
                    }
                    n876 = Build Array(w1636) -> (w1635:dbl[])
                    n877 = Build Array(w1637) -> (w1634:dbl[])
                    n878 = Bundle By Name(cluster=T5 {"X"=[], "Y"=[]} ("Data"), "X"=w1635, "Y"=w1634) -> (→"Data":T5)
                    "New data" <- TRUE ("New data")
                    "data time" <- w1649
                  }
                  frame "Get array" {
                    n879 = Variant To Data(type=T5 {"X"=[], "Y"=[]} ("Data"), Variant=w1662) -> (data=w1660:T5)  [unwired: 1 in, 1 out]
                    n880 = local write "New data"(TRUE ("New data")) -> ()
                    n881 = local write "Data"(w1660) -> ()
                    n882 = flat-sequence {
                      tunnel: w1657 -> [w1666]
                      tunnel: [w1666] -> w1656
                      tunnel: w1656 -> [w1667]
                      frame #0 {
                        n883 = local read "data time"() -> (w1665:timestamp)
                        n884 = Subtract(x=w1666, y=w1665) -> (x-y=→"data delay":dbl)
                      }
                      frame #1 {
                        n885 = local write "data time"(w1667) -> ()
                      }
                    }
                  }
                  frame "Get ModA" {
                    n886 = Variant To Data(type=0.0, Variant=w1675) -> (data=w1669:dbl)  [unwired: 1 in, 1 out]
                    n887 = local read "Sample holder"() -> (w1670:T13)
                    n888 = call "Modulation current to field conversion.vi"("Sample holder"=w1670, "Modulation current (mA)"=w1669) -> ("Modulation field (G)"=w1668:dbl)  [unwired: 9 in]
                    n889 = local read "Acquisition controls"() -> (w1673:T15)
                    n890 = Bundle By Name(cluster=w1673, "Modulation [A]"=w1669, "Mod_A [G]"=w1668) -> (w1672:T15)
                    n891 = local write "Acquisition controls"(w1672) -> ()
                  }
                  frame "End" {
                    n892 = Variant To Data(type=T65 {"handleValid"=FALSE, "Conn"=0, "Path Prefix"="", "Handle"=0, "Connected"=FALSE, "Clockbase(s)"=0.0} ("Handle Out"), Variant=w1685) -> ()  [unwired: 1 in, 2 out]
                    n893 = local read "loggersRef"() -> (w1682:refnum<file>)
                    n894 = property on="MFLI" class="Bool (strict)"("Value"=FALSE) -> ()  [unwired: 2 in, 2 out]
                    n895 = call "Add actual date time to string.vi"("String in"="ACQ disconnected") -> ("String out"=w1678:string)  [unwired: 4 in]
                    n896 = call "Write in logger.vi"("String in"=w1678, "logger refnum"=w1682) -> ()  [unwired: 2 in, 2 out]
                    n897 = call "simple Shift string array.vi"("Element in"=w1678, "Array in"=w1680) -> ("Array out"=w1679:string[])  [unwired: 8 in, 1 out]
                  }
                  frame "Ignore", Default {
                  }
                }
                n898 = Bundle By Name(cluster=w1562, "ACQ"=w1564) -> (w1563:T26)
              }
              frame "SMU2450" {
                n899 = Unbundle By Name(w1698) -> ("SMU"=w1695:T87)
                n900 = case shown="\"Set measurement\"" w1688 {
                  tunnel: w1693 -> [w1701 w1722 w1725 w1746 w1759 w1792 w1811]
                  tunnel: [w1701 w1721 w1725 w1747 w1759 w1793 w1812] -> w1692
                  tunnel: w1689 -> [_ w1717 _ w1745 w1776 w1794 w1813]
                  tunnel: w1694 -> [_ w1707 _ w1741 w1773 w1795 w1814]
                  tunnel: w1690 -> [w1700 w1716 w1724 w1740 w1772 w1799 w1818]
                  tunnel: [w1700 w1716 w1724 w1740 w1772 w1799 w1818] -> w1691
                  tunnel: w1695 -> [w1699 w1714 w1723 w1743 w1775 w1798 w1817]
                  tunnel: [w1699 w1713 w1723 w1742 w1774 w1797 w1816] -> w1696
                  frame "Ignore", Default {
                  }
                  frame "Connect" {
                    n901 = Variant To Data(type=T66 {"VISA name"="", "Connected"=FALSE, "Name"="", "Message"="", "Error message"="", "Min voltage"=0.0, "Max voltage"=0.0, "Min Current"=0.0, "Max Current"=0.0, "Measurement value"=0.0, "Source Voltage"=0.0, "Measurement"=FALSE, "Source Current"=0.0, "Source Mode"=0, "Measure Function"=0} ("output cluster"), Variant=w1717) -> (data=w1709:T66, error out=w1710:errorcluster)  [unwired: 1 in]
                    n902 = Unbundle By Name(w1709) -> ("Name"=w1702:string, "Message"=w1704:string, "Connected"=w1708:bool)  [unwired: 1 out]
                    n903 = local read "Instr status"() -> (w1719:T1)
                    n904 = Bundle By Name(cluster=w1719, "SMU"=w1708) -> (w1720:T1)
                    n905 = local write "Instr status"(w1720) -> ()
                    n906 = Concatenate Strings(w1702, " connected. " ("string"), w1704) -> (w1703:string)
                    n907 = Bundle By Name(cluster=w1714, "Name"=w1702, "Last update"=w1707) -> (w1713:T87)
                    n908 = property on="SMU controls" class="Clust (strict)"("DisabledEnum"=T32."Enabled" ("Disabled")) -> ()  [unwired: 2 in, 2 out]
                    n909 = local read "loggersRef"() -> (w1718:refnum<file>)
                    n910 = call "Add actual date time to string.vi"("String in"=w1703) -> ("String out"=w1706:string)  [unwired: 4 in]
                    n911 = call "Write in logger.vi"("error in"=w1710, "String in"=w1706, "logger refnum"=w1718) -> ("error out"=w1715:errorcluster)  [unwired: 1 in, 1 out]
                    n912 = call "simple Shift string array.vi"("Element in"=w1706, "Array in"=w1722) -> ("Array out"=w1721:string[])  [unwired: 8 in, 1 out]
                    n913 = call <vilib>:"Clear Errors.vi"("error in (no error)"=w1715) -> ()  [unwired: 5 in, 2 out]
                  }
                  frame "Update" {
                  }
                  frame "Set measurement" {
                    # "add surce funcion and value"
                    n914 = Variant To Data(type=T66 {"VISA name"="", "Connected"=FALSE, "Name"="", "Message"="", "Error message"="", "Min voltage"=0.0, "Max voltage"=0.0, "Min Current"=0.0, "Max Current"=0.0, "Measurement value"=0.0, "Source Voltage"=0.0, "Measurement"=FALSE, "Source Current"=0.0, "Source Mode"=0, "Measure Function"=0} ("SMU status out"), Variant=w1745) -> (data=w1739:T66)  [unwired: 1 in, 1 out]
                    n915 = Unbundle By Name(w1739) -> ("Measurement value"=w1727:dbl, "Measurement"=w1737:bool, "Source Voltage"=w1735:dbl, "Source Current"=w1736:dbl, "Source Mode"=w1729:u16, "Measure Function"=w1733:u16)
                    n916 = case shown="0, Default" w1729 {
                      tunnel: w1736 -> [_ w1753]
                      tunnel: w1735 -> [w1751 _]
                      tunnel: [w1751 w1753] -> w1728
                      tunnel: ["Voltage" "Current"] -> w1734
                      frame 0, Default {
                      }
                      frame 1 {
                      }
                    }
                    n917 = case shown="0, Default" w1733 {
                      tunnel: ["Voltage" "Current"] -> w1732
                      frame 0, Default {
                      }
                      frame 1 {
                      }
                    }
                    n918 = local read "SMU controls"() -> (w1731:T20)
                    n919 = Bundle By Name(cluster=w1731, "Measurement settings.Source Mode"=w1729, "Measurement settings.Source Level"=w1728, "Value"=w1727) -> (w1730:T20)
                    n920 = Bundle By Name(cluster=w1743, "Last update"=w1741, "Measure V"=w1727, "Output"=w1737, "Source F"=w1734, "Source V"=w1728, "Measure F"=w1732) -> (w1742:T87)
                    n921 = local write "SMU controls"(w1730) -> ()
                    n922 = call "Add actual date time to string.vi"("String in"="SMU set") -> ("String out"=w1744:string)  [unwired: 4 in]
                    n923 = call "simple Shift string array.vi"("Element in"=w1744, "Array in"=w1746) -> ("Array out"=w1747:string[])  [unwired: 8 in, 1 out]
                  }
                  frame "Get actual results" {
                    # "add surce funcion and value"
                    n924 = Variant To Data(type=T66 {"VISA name"="", "Connected"=FALSE, "Name"="", "Message"="", "Error message"="", "Min voltage"=0.0, "Max voltage"=0.0, "Min Current"=0.0, "Max Current"=0.0, "Measurement value"=0.0, "Source Voltage"=0.0, "Measurement"=FALSE, "Source Current"=0.0, "Source Mode"=0, "Measure Function"=0} ("SMU status out"), Variant=w1776) -> (data=w1771:T66)  [unwired: 1 in, 1 out]
                    n925 = Unbundle By Name(w1771) -> ("Measurement value"=w1757:dbl, "Measurement"=w1769:bool, "Source Voltage"=w1767:dbl, "Source Current"=w1768:dbl, "Source Mode"=w1761:u16, "Measure Function"=w1760:u16)
                    n926 = Add(x=w1757, y=3.7e-06) -> (x+y=w1755:dbl)
                    n927 = case shown="1" w1761 {
                      tunnel: w1768 -> [_ w1782]
                      tunnel: w1767 -> [w1780 _]
                      tunnel: [w1780 w1782] -> w1766
                      tunnel: ["Voltage" "Current"] -> w1765
                      frame 0, Default {
                      }
                      frame 1 {
                      }
                    }
                    n928 = case shown="0, Default" w1760 {
                      tunnel: ["Voltage" "Current"] -> w1764
                      frame 0, Default {
                      }
                      frame 1 {
                      }
                    }
                    n929 = Multiply(x=w1755, y=99.4) -> (x*y=w1758:dbl)
                    n930 = local read "SMU controls"() -> (w1763:T20)
                    n931 = Bundle By Name(cluster=w1763, "Value"=w1755, "B[T]"=w1758) -> (w1762:T20)
                    n932 = Bundle By Name(cluster=w1775, "Last update"=w1773, "Measure V"=w1757, "Output"=w1769, "Source F"=w1765, "Source V"=w1766, "Measure F"=w1764) -> (w1774:T87)
                    n933 = local write "SMU controls"(w1762) -> ()
                  }
                  frame "End" {
                    n934 = Variant To Data(type=T66 {"VISA name"="", "Connected"=FALSE, "Name"="", "Message"="", "Error message"="", "Min voltage"=0.0, "Max voltage"=0.0, "Min Current"=0.0, "Max Current"=0.0, "Measurement value"=0.0, "Source Voltage"=0.0, "Measurement"=FALSE, "Source Current"=0.0, "Source Mode"=0, "Measure Function"=0} ("SMU status out"), Variant=w1794) -> (data=w1787:T66)  [unwired: 1 in, 1 out]
                    n935 = Unbundle By Name(w1787) -> ("Name"=w1785:string, "Measurement"=w1783:bool)
                    n936 = Bundle By Name(cluster=w1798, "Name"="None" ("Master"), "Output"=w1783, "Last update"=w1795) -> (w1797:T87)
                    n937 = property on="SMU" class="Bool (strict)"("Value"=FALSE) -> ()  [unwired: 2 in, 2 out]
                    n938 = Concatenate Strings("SMU module " ("String in"), w1785, " ended." ("string")) -> (w1786:string)
                    n939 = call "Add actual date time to string.vi"("String in"=w1786) -> ("String out"=w1791:string)  [unwired: 4 in]
                    n940 = Concatenate Strings(w1791, "\r\n") -> (w1790:string)
                    n941 = local read "loggersRef"() -> (w1801:refnum<file>)
                    n942 = call "Write in logger.vi"("String in"=w1790, "logger refnum"=w1801) -> ()  [unwired: 2 in, 2 out]
                    n943 = call "simple Shift string array.vi"("Element in"=w1790, "Array in"=w1792) -> ("Array out"=w1793:string[])  [unwired: 8 in, 1 out]
                  }
                  frame "Disconnect" {
                    n944 = Variant To Data(type=T66 {"VISA name"="", "Connected"=FALSE, "Name"="", "Message"="", "Error message"="", "Min voltage"=0.0, "Max voltage"=0.0, "Min Current"=0.0, "Max Current"=0.0, "Measurement value"=0.0, "Source Voltage"=0.0, "Measurement"=FALSE, "Source Current"=0.0, "Source Mode"=0, "Measure Function"=0} ("SMU status out"), Variant=w1813) -> (data=w1808:T66)  [unwired: 1 in, 1 out]
                    n945 = Unbundle By Name(w1808) -> ("Name"=w1804:string, "Measurement"=w1803:bool)
                    n946 = Bundle By Name(cluster=w1817, "Name"="None" ("Master"), "Output"=w1803, "Last update"=w1814) -> (w1816:T87)
                    n947 = property on="SMU" class="Bool (strict)"("Value"=FALSE) -> ()  [unwired: 2 in, 2 out]
                    n948 = Concatenate Strings(w1804, " SMU disconnected." ("String in")) -> (w1805:string)
                    n949 = call "Add actual date time to string.vi"("String in"=w1805) -> ("String out"=w1810:string)  [unwired: 4 in]
                    n950 = Concatenate Strings(w1810, "\r\n") -> (w1809:string)
                    n951 = local read "loggersRef"() -> (w1820:refnum<file>)
                    n952 = call "Write in logger.vi"("String in"=w1809, "logger refnum"=w1820) -> ()  [unwired: 2 in, 2 out]
                    n953 = call "simple Shift string array.vi"("Element in"=w1809, "Array in"=w1811) -> ("Array out"=w1812:string[])  [unwired: 8 in, 1 out]
                  }
                }
                n954 = Bundle By Name(cluster=w1698, "SMU"=w1696) -> (w1697:T26)
              }
              frame "VTI" {
                n955 = Unbundle By Name(w1827) -> ("VTI"=w1825:T84)
                n956 = case shown="\"Update\"" w1832 {
                  tunnel: w1831 -> [_ w1852 w1872 w1888 _]
                  tunnel: w1830 -> [w1835 w1850 w1870 w1884 w1921]
                  tunnel: [w1835 w1849 w1870 w1883 w1920] -> w1829
                  tunnel: w1822 -> [w1834 w1840 w1868 w1886 w1916]
                  tunnel: [w1834 w1840 w1867 w1886 w1916] -> w1828
                  tunnel: w1825 -> [w1833 w1839 w1866 w1885 w1915]
                  tunnel: w1824 -> [_ _ w1856 _ _]
                  tunnel: [w1833 w1838 w1865 w1885 w1914] -> w1823
                  frame "Ignore", Default {
                  }
                  frame "Initialize" {
                    n957 = Variant To Data(type="", Variant=w1852) -> (data=w1837:string)  [unwired: 1 in, 1 out]
                    n958 = local read "Instr status"() -> (w1846:T1)
                    n959 = Bundle By Name(cluster=w1846, "VTI"=TRUE) -> (w1845:T1)
                    n960 = local write "Instr status"(w1845) -> ()
                    n961 = Concatenate Strings("Temperature controller " ("string"), w1837, " initialized" ("string")) -> (w1841:string)
                    n962 = local read "loggersRef"() -> (w1842:refnum<file>)
                    n963 = call "Add actual date time to string.vi"("String in"=w1841) -> ("String out"=w1843:string)  [unwired: 4 in]
                    n964 = call "Write in logger.vi"("String in"=w1843, "logger refnum"=w1842) -> ()  [unwired: 2 in, 2 out]
                    n965 = property on="VTI control" class="Clust (strict)"("DisabledEnum"=T32."Enabled" ("Disabled")) -> ()  [unwired: 2 in, 2 out]
                    n966 = Bundle By Name(cluster=w1839, "TC"=w1837) -> (w1838:T84)
                    n967 = call "simple Shift string array.vi"("Element in"=w1841, "Array in"=w1850) -> ("Array out"=w1849:string[])  [unwired: 8 in, 1 out]
                  }
                  frame "Update" {
                    n968 = Variant To Data(type=T67 {"VTI space"=0.0, "Sample"=0.0, "He pot"=0.0, "Trap"=0.0, "Ambient"=0.0, "SetP_VTI"=0.0, "SetP_Smp"=0.0, "SetP_Pot"=0.0, "SetP_Trap"=0.0, "Range out 1"=1, "Out 1 [%]"=0.0, "Out 2 [%]"=0.0} ("TC sensors [K]"), Variant=w1872) -> (data=w1869:T67)  [unwired: 1 in, 1 out]
                    n969 = Unbundle By Name(w1869) -> ("Ambient"=w1855:dbl, "VTI space"=w1854:dbl, "Sample"=w1853:dbl, "Trap"=w1864:dbl, "He pot"=w1863:dbl, "SetP_VTI"=w1860:dbl, "SetP_Smp"=w1859:dbl, "SetP_Pot"=w1858:dbl, "SetP_Trap"=w1857:dbl)
                    n970 = local read "VTI control"() -> (w1862:T21)
                    n971 = Bundle By Name(cluster=w1866, "Last update"=w1856, "Ambient [K]"=w1855, "VTI [K]"=w1854, "Sample [K]"=w1853, "Trap[K]"=w1864, "HePot [K]"=w1863) -> (w1865:T84)
                    n972 = Bundle By Name(cluster=w1862, "VTI space [K]"=w1860, "Sample [K]"=w1859, "Heater3 [K]"=w1858, "Heater4 [K]"=w1857) -> (w1861:T21)
                    n973 = Bundle By Name(cluster=w1868, "T_sample [K]"=w1853) -> (w1867:T24)
                    n974 = local write "VTI control"(w1861) -> ()
                  }
                  frame "Set point" {
                    n975 = Variant To Data(type=T48 {"Heater"="", "Tmp [K]"=0.0}, Variant=w1888) -> (data=w1887:T48)  [unwired: 1 in, 1 out]
                    n976 = Unbundle By Name(w1887) -> ("Heater"=w1877:string, "Tmp [K]"=w1874:dbl)
                    n977 = local read "VTI control"() -> (w1876:T21)
                    n978 = case shown="\"Heater3 [K]\"" w1877 {
                      selector: w1877 -> [_ w1892 w1897 w1905 w1910]
                      tunnel: [u16 0 ("Output's Control Loop (1:1)") w1896 w1901 w1906 w1911] -> _
                      tunnel: w1874 -> [_ w1893 w1898 w1902 w1907]
                      tunnel: w1876 -> [w1890 w1895 w1900 w1904 w1909]
                      tunnel: [w1890 w1894 w1899 w1903 w1908] -> w1875
                      tunnel: ["Unknown setpoint" w1892 w1897 w1905 w1910] -> w1873
                      frame "None", Default {
                      }
                      frame "VTI space [K]" {
                        w1896 = u16 1 items=["1"=1, "2"=2, "3"=3, "4"=4] ("Output's Control Loop (1:1)")
                        n979 = Bundle By Name(cluster=w1895, "VTI space [K]"=w1893) -> (w1894:T21)
                      }
                      frame "Sample [K]" {
                        w1901 = u16 2 items=["1"=1, "2"=2, "3"=3, "4"=4] ("Output's Control Loop (1:1)")
                        n980 = Bundle By Name(cluster=w1900, "Sample [K]"=w1898) -> (w1899:T21)
                      }
                      frame "Heater3 [K]" {
                        w1906 = u16 3 items=["1"=1, "2"=2, "3"=3, "4"=4] ("Output's Control Loop (1:1)")
                        n981 = Bundle By Name(cluster=w1904, "Heater3 [K]"=w1902) -> (w1903:T21)
                      }
                      frame "Heater4 [K]" {
                        w1911 = u16 4 items=["1"=1, "2"=2, "3"=3, "4"=4] ("Output's Control Loop (1:1)")
                        n982 = Bundle By Name(cluster=w1909, "Heater4 [K]"=w1907) -> (w1908:T21)
                      }
                    }
                    n983 = local write "VTI control"(w1875) -> ()
                    n984 = Format Into String(format string="%f K", initial string=w1873, w1874) -> (resulting string=w1881:string)  [unwired: 1 in, 1 out]
                    n985 = local read "loggersRef"() -> (w1882:refnum<file>)
                    n986 = call "Add actual date time to string.vi"("String in"=w1881) -> ("String out"=w1879:string)  [unwired: 4 in]
                    n987 = call "simple Shift string array.vi"("Element in"=w1879, "Array in"=w1884) -> ("Array out"=w1883:string[])  [unwired: 8 in, 1 out]
                    n988 = call "Write in logger.vi"("String in"=w1879, "logger refnum"=w1882) -> ()  [unwired: 2 in, 2 out]
                  }
                  frame "End" {
                    w1918 = "VTI closed" ("Element in")
                    n989 = local read "Instr status"() -> (w1924:T1)
                    n990 = Bundle By Name(cluster=w1915, "TC"="None") -> (w1914:T84)
                    n991 = Bundle By Name(cluster=w1924, "VTI"=FALSE) -> (w1922:T1)
                    n992 = local write "Instr status"(w1922) -> ()
                    n993 = property on="VTI control" class="Clust (strict)"("DisabledEnum"=T32."Disabled and Grayed Out" ("Disabled")) -> ()  [unwired: 2 in, 2 out]
                    n994 = call "Add actual date time to string.vi"("String in"=w1918) -> ("String out"=w1917:string)  [unwired: 4 in]
                    n995 = local read "loggersRef"() -> (w1919:refnum<file>)
                    n996 = call "simple Shift string array.vi"("Element in"=w1918, "Array in"=w1921) -> ("Array out"=w1920:string[])  [unwired: 8 in, 1 out]
                    n997 = call "Write in logger.vi"("String in"=w1917, "logger refnum"=w1919) -> ()  [unwired: 2 in, 2 out]
                  }
                }
                n998 = call "simple Shift string array.vi"() -> ()  [unwired: 10 in, 2 out]
                n999 = Bundle By Name(cluster=w1827, "VTI"=w1823) -> (w1826:T26)
              }
              frame "Servo" {
                n1000 = Unbundle By Name(w1929) -> ("Servo"=w1927:T10[])
                n1001 = case shown="\"Move by\"" w1931 {
                  selector: w1931 -> [w1951 w1999 w2052 _ w2125]
                  tunnel: w1934 -> [w1953 w2001 w2059 _ w2123]
                  tunnel: w1933 -> [w1949 w1997 w2055 w2110 w2128]
                  tunnel: [w1950 w1998 w2056 w2111 w2127] -> w1932
                  tunnel: w1927 -> [w1936 w1985 w2038 w2106 w2117]
                  tunnel: [w1935 w1987 w2037 w2105 w2117] -> w1926
                  tunnel: w1925 -> [w1937 _ w2035 _ _]
                  frame "Initialize" {
                    n1002 = Variant To Data(type=T68[] [] ("Servo status"), Variant=w1953) -> (data=w1939:T68[])  [unwired: 1 in, 1 out]
                    n1003 = Index Array(array=w1936) -> (element=w1938:T10)  [unwired: 1 in]
                    n1004 = for {
                      tunnel: w1939 -> [w1969] mode=indexing
                      tunnel: w1938 -> [w1965]
                      tunnel: w1937 -> [w1963]
                      tunnel: [w1957] -> w1935 mode=indexing
                      n1005 = Unbundle By Name(w1969) -> ("Servo constants.Name"=w1964:T11, "Servo variables.Actual position"=w1962:dbl, "Servo constants.Pos position limit [mm]"=w1959:dbl, "Servo constants.Neg position limit [mm]"=w1958:dbl, "Servo variables.Power ON"=w1960:bool, "Servo variables.Connected"=w1961:bool)
                      n1006 = Select(t=T32."Enabled" ("Disabled"), s=w1961, f=T32."Disabled and Grayed Out" ("Disabled")) -> (s? t:f=w1966:T32)
                      n1007 = Bundle By Name(cluster=w1965, "Name"=w1964, "Last update"=w1963, "Position"=w1962, "Pos limit"=w1959, "Neg limit"=w1958, "Power"=w1960) -> (w1957:T10)
                      n1008 = case shown="\"AxisX\", Default" w1964 {
                        tunnel: w1962 -> [w1971 w1973 w1975 w1977 w1979]
                        tunnel: w1961 -> [_ _ _ _ _]
                        tunnel: w1966 -> [w1970 w1972 w1974 w1976 w1978]
                        frame "AxisX", Default {
                          n1009 = property on="X backward" class="Bool (strict)"("DisabledEnum"=w1970) -> ()  [unwired: 2 in, 2 out]
                          n1010 = property on="X forward" class="Bool (strict)"("DisabledEnum"=w1970) -> ()  [unwired: 2 in, 2 out]
                          n1011 = property on="X" class="DigNum (strict)"("Value"=w1971) -> ()  [unwired: 2 in, 2 out]
                        }
                        frame "AxisY" {
                          n1012 = property on="Y left" class="Bool (strict)"("DisabledEnum"=w1972) -> ()  [unwired: 2 in, 2 out]
                          n1013 = property on="Y right" class="Bool (strict)"("DisabledEnum"=w1972) -> ()  [unwired: 2 in, 2 out]
                          n1014 = property on="Y" class="DigNum (strict)"("Value"=w1973) -> ()  [unwired: 2 in, 2 out]
                        }
                        frame "AxisZ_left" {
                          n1015 = property on="ZLup" class="Bool (strict)"("DisabledEnum"=w1974) -> ()  [unwired: 2 in, 2 out]
                          n1016 = property on="ZLdown" class="Bool (strict)"("DisabledEnum"=w1974) -> ()  [unwired: 2 in, 2 out]
                          n1017 = property on="ZL" class="DigNum (strict)"("Value"=w1975) -> ()  [unwired: 2 in, 2 out]
                        }
                        frame "AxisZ_middle" {
                          n1018 = property on="ZM" class="DigNum (strict)"("Value"=w1977) -> ()  [unwired: 2 in, 2 out]
                          n1019 = property on="ZMdown" class="Bool (strict)"("DisabledEnum"=w1976) -> ()  [unwired: 2 in, 2 out]
                          n1020 = property on="ZMup" class="Bool (strict)"("DisabledEnum"=w1976) -> ()  [unwired: 2 in, 2 out]
                        }
                        frame "AxisZ_right" {
                          n1021 = property on="ZRup" class="Bool (strict)"("DisabledEnum"=w1978) -> ()  [unwired: 2 in, 2 out]
                          n1022 = property on="ZRdown" class="Bool (strict)"("DisabledEnum"=w1978) -> ()  [unwired: 2 in, 2 out]
                          n1023 = property on="ZR" class="DigNum (strict)"("Value"=w1979) -> ()  [unwired: 2 in, 2 out]
                        }
                      }
                    }
                    n1024 = for {
                      tunnel: w1939 -> [w1981] mode=indexing
                      tunnel: [w1980] -> w1943 mode=indexing
                      n1025 = Unbundle By Name(w1981) -> ("Servo variables.Connected"=w1980:bool)
                    }
                    n1026 = And Array Elements(Boolean array=w1943) -> (logical AND=w1942:bool)
                    n1027 = call <vilib>:"Space Constant.vi"() -> ("String"=w1945:string)
                    n1028 = case shown="True" w1942 {
                      frame False {
                      }
                      frame True {
                        n1029 = control-ref of="Servo controls"() -> (w1956:refnum<vi>)
                        n1030 = Build Array(w1956) -> (w1955:refnum<vi>[])
                        n1031 = call "Dis- or en- able controls.vi"("Disabled"=T32."Enabled", "Control referencies"=w1955) -> ()  [unwired: 9 in, 1 out]
                      }
                    }
                    n1032 = local read "Instr status"() -> (w1948:T1)
                    n1033 = Concatenate Strings("Servo" ("string"), w1945, w1951, w1945) -> (w1952:string)
                    n1034 = local read "loggersRef"() -> (w1941:refnum<file>)
                    n1035 = Bundle By Name(cluster=w1948, "Serv"=w1942) -> (w1947:T1)
                    n1036 = call "Add actual date time to string.vi"("String in"=w1952) -> ("String out"=w1940:string)  [unwired: 4 in]
                    n1037 = local write "Instr status"(w1947) -> ()
                    n1038 = call "simple Shift string array.vi"("Element in"=w1940, "Array in"=w1949) -> ("Array out"=w1950:string[])  [unwired: 8 in, 1 out]
                    n1039 = call "Write in logger.vi"("String in"=w1940, "logger refnum"=w1941) -> ()  [unwired: 2 in, 2 out]
                  }
                  frame "Move by" {
                    n1040 = Variant To Data(type=T71 {"Property"="", "Value"=variant, "Name"=enum."AxisX"} ("Array"), Variant=w2001) -> (data=w1993:T71)  [unwired: 1 in, 1 out]
                    n1041 = Unbundle By Name(w1993) -> ("Property"=w1992:string, "Value"=w1991:variant, "Name"=w1990:T11)
                    n1042 = call "Extract axis properties.vi"("Name"=w1990, "All servo status"=w1985) -> ("Servo"=w1984:T10, "Index"=w1986:i32, "Found?"=w1988:bool)  [unwired: 6 in]
                    n1043 = case shown="True" w1988 {
                      tunnel: w1992 -> [w2003 w2012]
                      tunnel: w1991 -> [_ w2011]
                      tunnel: w1990 -> [_ w2010]
                      tunnel: w1984 -> [_ w2009]
                      tunnel: w1986 -> [_ w2008]
                      tunnel: w1985 -> [w2002 w2007]
                      tunnel: [w2003 w2005] -> w1989
                      tunnel: [w2002 w2004] -> w1987
                      frame False {
                      }
                      frame True {
                        n1044 = case shown="\"Power ON\"" w2012 {
                          selector: w2012 -> [w2013 w2016 w2028]
                          tunnel: w2011 -> [_ w2015 w2034]
                          tunnel: w2010 -> [_ w2018 _]
                          tunnel: w2009 -> [w2014 w2021 w2032]
                          tunnel: [w2014 w2020 w2031] -> w2006
                          tunnel: [w2013 w2019 w2030] -> w2005
                          frame "Nothing", Default {
                          }
                          frame "Actual position" {
                            n1045 = Variant To Data(type=0.0, Variant=w2015) -> (data=w2017:dbl)  [unwired: 1 in, 1 out]
                            n1046 = case shown="\"AxisZ_right\"" w2018 {
                              tunnel: w2017 -> [w2023 w2024 w2025 w2026 w2027]
                              frame "AxisX", Default {
                                n1047 = property on="X" class="DigNum (strict)"("Val(Sgnl)"=w2023) -> ()  [unwired: 2 in, 2 out]
                              }
                              frame "AxisY" {
                                n1048 = property on="Y" class="DigNum (strict)"("Value"=w2024) -> ()  [unwired: 2 in, 2 out]
                              }
                              frame "AxisZ_left" {
                                n1049 = property on="ZL" class="DigNum (strict)"("Value"=w2025) -> ()  [unwired: 2 in, 2 out]
                              }
                              frame "AxisZ_middle" {
                                n1050 = property on="ZM" class="DigNum (strict)"("Value"=w2026) -> ()  [unwired: 2 in, 2 out]
                              }
                              frame "AxisZ_right" {
                                n1051 = property on="ZR" class="DigNum (strict)"("Value"=w2027) -> ()  [unwired: 2 in, 2 out]
                              }
                            }
                            n1052 = Bundle By Name(cluster=w2021, "Position"=w2017) -> (w2020:T10)
                            n1053 = Format Into String(initial string=w2016, w2017) -> (resulting string=w2019:string)  [unwired: 2 in, 1 out]
                          }
                          frame "Power ON" {
                            n1054 = Variant To Data(type=FALSE ("Connected"), Variant=w2034) -> (data=w2029:bool)  [unwired: 1 in, 1 out]
                            n1055 = Bundle By Name(cluster=w2032, "Power"=w2029) -> (w2031:T10)
                            n1056 = Format Into String(initial string=w2028, w2029) -> (resulting string=w2030:string)  [unwired: 2 in, 1 out]
                          }
                        }
                        n1057 = Replace Array Subset(array=w2007, new element=w2006, index=w2008) -> (w2004:T10[])
                      }
                    }
                    n1058 = call <vilib>:"Space Constant.vi"() -> ("String"=w1995:string)
                    n1059 = local read "loggersRef"() -> (w1982:refnum<file>)
                    n1060 = Concatenate Strings("Servo" ("string"), w1995, w1999, w1995, w1989) -> (w2000:string)
                    n1061 = call "Add actual date time to string.vi"("String in"=w2000) -> ("String out"=w1983:string)  [unwired: 4 in]
                    n1062 = call "Write in logger.vi"("String in"=w1983, "logger refnum"=w1982) -> ()  [unwired: 2 in, 2 out]
                    n1063 = call "simple Shift string array.vi"("Element in"=w1983, "Array in"=w1997) -> ("Array out"=w1998:string[])  [unwired: 8 in, 1 out]
                  }
                  frame "Update" {
                    n1064 = Variant To Data(type=T71 {"Property"="", "Value"=variant, "Name"=enum."AxisX"} ("Array"), Variant=w2059) -> (data=w2051:T71)  [unwired: 1 in, 1 out]
                    n1065 = Unbundle By Name(w2051) -> ("Property"=w2045:string, "Value"=w2050:variant, "Name"=w2047:T11)
                    n1066 = call "Extract axis properties.vi"("Name"=w2047, "All servo status"=w2038) -> ("Servo"=w2049:T10, "Index"=w2048:i32, "Found?"=w2040:bool)  [unwired: 6 in]
                    n1067 = Format Into String(w2047) -> (resulting string=w2046:string)  [unwired: 3 in, 1 out]
                    n1068 = Bundle By Name(cluster=w2049, "Last update"=w2035) -> (w2036:T10)
                    n1069 = call <vilib>:"Space Constant.vi"() -> ("String"=w2042:string)
                    n1070 = Concatenate Strings(w2045, w2042, w2046, ":" ("string"), w2042) -> (w2044:string)
                    n1071 = case shown="False" w2040 {
                      tunnel: w2050 -> [_ w2076]
                      tunnel: w2036 -> [_ w2075]
                      tunnel: w2038 -> [w2060 w2074]
                      tunnel: w2048 -> [_ w2072]
                      tunnel: w2047 -> [w2066 w2071]
                      tunnel: w2045 -> [w2062 w2070]
                      tunnel: w2044 -> [_ w2069]
                      tunnel: [w2064 w2068] -> w2041
                      tunnel: [w2060 w2067] -> w2037
                      frame False {
                        n1072 = call <vilib>:"Space Constant.vi"() -> ("String"=w2061:string)
                        n1073 = Concatenate Strings(w2062, w2061, "Unknown driver" ("initial string")) -> (w2063:string)
                        n1074 = Format Into String(initial string=w2063, w2066) -> (resulting string=w2064:string)  [unwired: 2 in, 1 out]
                      }
                      frame True {
                        n1075 = case shown="\"Target position\"" w2070 {
                          tunnel: w2076 -> [_ w2086 w2097 w2104]
                          tunnel: w2071 -> [_ w2080 _ _]
                          tunnel: w2075 -> [w2078 w2084 w2095 w2102]
                          tunnel: [w2078 w2083 w2095 w2101] -> w2073
                          tunnel: w2069 -> [w2077 w2082 w2092 w2099]
                          tunnel: [w2077 w2081 w2094 w2100] -> w2068
                          frame "Nothing", Default {
                          }
                          frame "Actual position" {
                            n1076 = Variant To Data(type=0.0, Variant=w2086) -> (data=w2079:dbl)  [unwired: 1 in, 1 out]
                            n1077 = case shown="\"AxisZ_left\"" w2080 {
                              tunnel: w2079 -> [w2087 w2088 w2089 w2090 w2091]
                              frame "AxisX", Default {
                                n1078 = property on="X" class="DigNum (strict)"("Val(Sgnl)"=w2087) -> ()  [unwired: 2 in, 2 out]
                              }
                              frame "AxisY" {
                                n1079 = property on="Y" class="DigNum (strict)"("Value"=w2088) -> ()  [unwired: 2 in, 2 out]
                              }
                              frame "AxisZ_left" {
                                n1080 = property on="ZL" class="DigNum (strict)"("Value"=w2089) -> ()  [unwired: 2 in, 2 out]
                              }
                              frame "AxisZ_middle" {
                                n1081 = property on="ZM" class="DigNum (strict)"("Value"=w2090) -> ()  [unwired: 2 in, 2 out]
                              }
                              frame "AxisZ_right" {
                                n1082 = property on="ZR" class="DigNum (strict)"("Value"=w2091) -> ()  [unwired: 2 in, 2 out]
                              }
                            }
                            n1083 = Bundle By Name(cluster=w2084, "Position"=w2079) -> (w2083:T10)
                            n1084 = Format Into String(initial string=w2082, w2079) -> (resulting string=w2081:string)  [unwired: 2 in, 1 out]
                          }
                          frame "Target position" {
                            n1085 = Variant To Data(type=0.0, Variant=w2097) -> (data=w2093:dbl)  [unwired: 1 in, 1 out]
                            n1086 = Format Into String(initial string=w2092, w2093) -> (resulting string=w2094:string)  [unwired: 2 in, 1 out]
                          }
                          frame "Power ON" {
                            n1087 = Variant To Data(type=FALSE ("Connected"), Variant=w2104) -> (data=w2098:bool)  [unwired: 1 in, 1 out]
                            n1088 = Bundle By Name(cluster=w2102, "Power"=w2098) -> (w2101:T10)
                            n1089 = Format Into String(initial string=w2099, w2098) -> (resulting string=w2100:string)  [unwired: 2 in, 1 out]
                          }
                        }
                        n1090 = Replace Array Subset(array=w2074, new element=w2073, index=w2072) -> (w2067:T10[])
                      }
                    }
                    n1091 = call <vilib>:"Space Constant.vi"() -> ("String"=w2039:string)
                    n1092 = Concatenate Strings("Servo" ("string"), w2039, w2052, w2039, w2039, w2039, w2041, w2039) -> (w2053:string)
                    n1093 = call "Add actual date time to string.vi"("String in"=w2053) -> ("String out"=w2057:string)  [unwired: 4 in]
                    n1094 = call "simple Shift string array.vi"("Element in"=w2057, "Array in"=w2055) -> ("Array out"=w2056:string[])  [unwired: 8 in, 1 out]
                  }
                  frame "End" {
                    w2108 = "Servo disconnected" ("Element in")
                    n1095 = Array Size(array=w2106) -> (size(s)=w2107:i32)
                    n1096 = local read "Instr status"() -> (w2115:T1)
                    n1097 = control-ref of="Servo controls"() -> (w2113:refnum<vi>)
                    n1098 = Delete From Array(array=w2106, length=w2107) -> (array with subset deleted=w2105:T10[])  [unwired: 1 in, 1 out]
                    n1099 = Bundle By Name(cluster=w2115, "Serv"=FALSE ("PSU")) -> (w2116:T1)
                    n1100 = local write "Instr status"(w2116) -> ()
                    n1101 = property class="Clust"(reference=w2113, "DisabledEnum"=T32."Disabled and Grayed Out" ("Disabled")) -> ()  [unwired: 1 in, 2 out]
                    n1102 = local read "loggersRef"() -> (w2109:refnum<file>)
                    n1103 = call "simple Shift string array.vi"("Element in"=w2108, "Array in"=w2110) -> ("Array out"=w2111:string[])  [unwired: 8 in, 1 out]
                    n1104 = call "Write in logger.vi"("String in"=w2108, "logger refnum"=w2109) -> ()  [unwired: 2 in, 2 out]
                  }
                  frame "Error", Default {
                    n1105 = Variant To Data(type=errorcluster {"status"=FALSE, "code"=0, "source"=""} ("error constant"), Variant=w2123) -> (data=w2121:errorcluster)  [unwired: 1 in, 1 out]
                    n1106 = Unbundle By Name(w2121) -> ("source"=w2120:string)
                    n1107 = call <vilib>:"Space Constant.vi"() -> ("String"=w2126:string)
                    n1108 = Concatenate Strings(w2125, w2126, w2120) -> (w2124:string)
                    n1109 = local read "loggersRef"() -> (w2119:refnum<file>)
                    n1110 = call "Add actual date time to string.vi"("String in"=w2124) -> ("String out"=w2118:string)  [unwired: 4 in]
                    n1111 = call "simple Shift string array.vi"("Element in"=w2118, "Array in"=w2128) -> ("Array out"=w2127:string[])  [unwired: 8 in, 1 out]
                    n1112 = call "Write in logger.vi"("String in"=w2118, "logger refnum"=w2119) -> ()  [unwired: 2 in, 2 out]
                  }
                }
                n1113 = Bundle By Name(cluster=w1929, "Servo"=w1926) -> (w1928:T26)
              }
              frame "Rotator" {
                n1114 = Format Into String(w2136) -> (resulting string=w2134:string)  [unwired: 3 in, 1 out]
                n1115 = Unbundle By Name(w2133) -> ("Rot"=w2132:T88)
                n1116 = case shown="\"End\"" w2140 {
                  selector: w2140 -> [_ _ _ _ w2186 _]
                  tunnel: w2139 -> [_ w2153 w2173 w2176 w2190 _]
                  tunnel: w2138 -> [w2142 w2151 w2169 w2177 w2181 w2200]
                  tunnel: [w2142 w2150 w2169 w2177 w2180 w2200] -> w2137
                  tunnel: w2134 -> [_ w2143 _ _ w2188 _]
                  tunnel: w2132 -> [w2141 w2144 w2167 w2174 w2178 w2193]
                  tunnel: [w2141 w2144 w2166 w2174 w2178 w2192] -> w2130
                  tunnel: w2129 -> [_ _ w2165 _ _ _]
                  frame "Ignore", Default {
                  }
                  frame "Initialize" {
                    n1117 = Variant To Data(type=T72 {"deviceNumber"=0, "DeviceType"=0, "ID"=0, "Serial"="", "Address"="", "connected"=FALSE} ("controller info"), Variant=w2153) -> (data=w2147:T72)  [unwired: 1 in, 1 out]
                    n1118 = Unbundle By Name(w2147) -> ("DeviceType"=w2149:i32, "connected"=w2146:bool)
                    n1119 = Format Into String(w2149) -> (resulting string=w2148:string)  [unwired: 3 in, 1 out]
                    n1120 = property on="Rot" class="Bool (strict)"("Value"=w2146) -> ()  [unwired: 2 in, 2 out]
                    n1121 = case shown="True" w2146 {
                      tunnel: w2151 -> [w2154 w2161]
                      tunnel: [w2154 w2160] -> w2150
                      tunnel: w2148 -> [_ _]
                      tunnel: w2143 -> [_ w2156]
                      tunnel: " connected: " ("string") -> [_ w2155]
                      frame False {
                      }
                      frame True {
                        n1122 = Concatenate Strings(w2156, w2155) -> (w2159:string)
                        n1123 = local read "loggersRef"() -> (w2158:refnum<file>)
                        n1124 = call "Add actual date time to string.vi"("String in"=w2159) -> ("String out"=w2157:string)  [unwired: 4 in]
                        n1125 = call "simple Shift string array.vi"("Array in"=w2161) -> ("Array out"=w2160:string[])  [unwired: 9 in, 1 out]
                        n1126 = call "Write in logger.vi"("String in"=w2157, "logger refnum"=w2158) -> ()  [unwired: 2 in, 2 out]
                      }
                    }
                  }
                  frame "Update" {
                    n1127 = Variant To Data(type=T73 {"Axis status"={"Connected"=FALSE, "Enabled"=FALSE, "Moving"=FALSE, "Target"=FALSE, "EndForward"=FALSE, "EndBackarwd"=FALSE, "Error"=FALSE}, "Position [°]"=0.0, "Frequency [Hz]"=0.0, "Voltage [V]"=0.0, "Capacitance[uF]"=0.0, "Name"="", "ActuatorType"=0, "DC offset [V]"=0.0, "Tolerance [m°]"=0.0, "Index"=0} ("Axis status"), Variant=w2173) -> (data=w2168:T73)  [unwired: 1 in, 1 out]
                    n1128 = Unbundle By Name(w2168) -> ("Axis status.Connected"=w2162:bool, "Position [°]"=w2164:dbl, "Axis status.Target"=w2163:bool)  [unwired: 3 out]
                    n1129 = Select(t=T32."Enabled" ("Disabled"), s=w2162, f=T32."Disabled and Grayed Out" ("Disabled")) -> ()  [unwired: 1 out]
                    n1130 = Bundle By Name(cluster=w2167, "Last update"=w2165, "Position [°]"=w2164, "Connected"=w2162, "Target"=w2163) -> (w2166:T88)
                  }
                  frame "Set parameters" {
                    n1131 = Variant To Data(type=T74 {"Frequency [Hz]"=1000.0, "MaxErr [µm|m°]"=10.0, "DC voltage [V]"=1.0, "Amplitude [V]"=6.0, "Position [mm|°]"=0.0, "EoF"=FALSE, "EoB"=FALSE, "Error"=FALSE, "Target [mm|°]"=0.0} ("Motion parameters"), Variant=w2176) -> ()  [unwired: 1 in, 2 out]
                  }
                  frame "Set position" {
                    n1132 = Variant To Data(type=T75 {"Relative?"=FALSE, "Position [°]"=0.0, "Safe to move?"=FALSE} ("Set position"), Variant=w2190) -> (data=w2184:T75)  [unwired: 1 in, 1 out]
                    n1133 = Unbundle By Name(w2184) -> ("Position [°]"=w2183:dbl)
                    n1134 = Format Into String(w2183) -> (resulting string=w2182:string)  [unwired: 3 in, 1 out]
                    n1135 = Concatenate Strings(w2188, ": " ("string"), w2186, " " ("string"), w2182) -> (w2179:string)
                    n1136 = call "simple Shift string array.vi"("Element in"=w2179, "Array in"=w2181) -> ("Array out"=w2180:string[])  [unwired: 8 in, 1 out]
                  }
                  frame "End" {
                    n1137 = local read "Instr status"() -> (w2198:T1)
                    n1138 = Bundle By Name(cluster=w2198, "Rot"=FALSE ("PSU")) -> (w2199:T1)
                    n1139 = call "Add actual date time to string.vi"("String in"="Rotator module ended") -> ("String out"=w2196:string)  [unwired: 4 in]
                    n1140 = local write "Instr status"(w2199) -> ()
                    n1141 = local read "loggersRef"() -> (w2195:refnum<file>)
                    n1142 = call "Write in logger.vi"("String in"=w2196, "logger refnum"=w2195) -> ()  [unwired: 2 in, 2 out]
                    n1143 = Bundle By Name(cluster=w2193, "Name"=u16 3) -> (w2192:T88)
                  }
                }
                n1144 = Bundle By Name(cluster=w2133, "Rot"=w2130) -> (w2131:T26)
              }
              frame "Emty", Default {
                n1145 = Format Into String(w2206) -> (resulting string=w2205:string)  [unwired: 3 in, 1 out]
                n1146 = call <vilib>:"Space Constant.vi"() -> ("String"=w2207:string)
                n1147 = Concatenate Strings(w2205, w2207, w2204) -> (w2203:string)
                n1148 = call "simple Shift string array.vi"("Element in"=w2203, "Array in"=w2209) -> ("Array out"=w2208:string[])  [unwired: 8 in, 1 out]
              }
            }
          }
          frame True {
          }
        }
        "Instr info" <- w1171
        n1149 = local read "Busy"() -> (w1179:bool)
        n1150 = Unbundle By Name(w1170) -> ("Experiment state"=w1169:T25)
        n1151 = Not(x=w1179) -> (.not. x?=w1177:bool)
        n1152 = Greater?(x=w1182, y=2) -> (0:w1180:bool)
        n1153 = And(x=w1180, y=w1177) -> (x .and. y?=w1178:bool)
        n1154 = case shown="False" w1178 {
          selector: w1178 -> [w1197 w1198]
          tunnel: [w1195 TopStates."Check message" ("State")] -> w1176
          tunnel: w1169 -> [w1191 _]
          frame False {
            n1155 = local write "Busy"(w1197) -> ()
            n1156 = Equal?(x=w1191, y=experiment_state."Setup" ("Value")) -> (x = y?=w1193:bool)
            n1157 = Select(t=TopStates."Wait for Event" ("State"), s=w1193, f=TopStates."Check measurement") -> (s? t:f=w1195:T28)
          }
          frame True {
            "Busy" <- w1198
          }
        }
      }
      frame "Check measurement" {
        n1158 = Unbundle By Name(w2214) -> ("Experiment state"=w2216:T25, "Remains"=w2213:dbl)
        n1159 = case shown="\"Acquisition\"" w2216 {
          tunnel: w2222 -> [_ w2264 w2300 _ _ w2461]
          tunnel: w2218 -> [w2224 w2259 w2294 w2347 w2354 w2467]
          tunnel: w2221 -> [w2226 w2279 w2299 w2349 w2360 w2471]
          tunnel: [w2226 w2277 w2298 w2349 w2360 w2470] -> w2220
          tunnel: [w2225 w2276 w2296 w2348 w2356 w2468] -> w2219
          tunnel: w2214 -> [w2225 w2275 w2297 w2348 w2357 w2469]
          tunnel: [w2224 w2259 w2293 w2347 w2354 w2467] -> w2217
          tunnel: w2215 -> [_ _ w2292 _ w2352 _]
          tunnel: w2214 -> [_ _ _ _ w2351 _]
          tunnel: w2213 -> [_ _ _ _ _ _]
          frame "Setup", Default {
            # "here can be implemented check of input parameters before measurement"
          }
          frame "Preparation" {
            w2250 = u8 1 ("X Scale.Scale Fit")
            n1160 = local read "Acquisition controls"() -> (w2263:T15)
            n1161 = Unbundle By Name(w2263) -> ("ACQ parameters"=w2260:T14)
            n1162 = local read "Folder path"() -> (w2267:path)
            n1163 = call "Create TDMS map file.vi"("Sample name"="Sample name", "Description"="Description", "Folder path"=w2267, "Operator"="Operator", "Sample holder"="Sample holder", "Map parameters"=w2259, "ACQ parameters"=w2260) -> ("error out"=w2262:errorcluster, "tdms map file out"=→"tdms map file out":refnum<k34>)  [unwired: 3 in]
            n1164 = call "Prepare map measurement.vi"("error in (no error)"=w2262, "Map parameters"=w2259, "ACQ parameters"=w2260, "Referencies in"=w2264) -> ("error out"=w2261:errorcluster)  [unwired: 7 in]
            n1165 = Unbundle By Name(w2259) -> ("F_start[GHz]"=w2255:dbl, "F_end[GHz]"=w2254:dbl, "Points"=w2232:u32, "B_start[T]"=w2248:dbl, "B_End[T]"=w2247:dbl, "B_rate [mT/s]"=w2258:dbl, "Sweep [s]"=w2230:dbl)
            n1166 = Quotient & Remainder(x=w2232, y=u32 4096) -> (floor(x/y)=w2235:u32)  [unwired: 1 out]
            n1167 = Less Or Equal To 0?(x=w2235) -> (x <= 0?=w2234:bool)
            n1168 = Add(x=w2230, y="MW trig low [s]") -> (x+y=w2238:dbl)
            n1169 = case shown="False" w2234 {
              tunnel: w2235 -> [w2283 _]
              tunnel: w2232 -> [w2282 w2284]
              tunnel: [w2281 w2284] -> w2231
              frame False {
                n1170 = Divide(x=w2282, y=w2283) -> (x/y=w2281:dbl)
              }
              frame True {
              }
            }
            n1171 = Compound Arithmetic op=MULTIPLY(w2238, w2258, 0.001 ("y")) -> (w2245:dbl)
            n1172 = Subtract(x=w2255, y=w2254) -> (x-y=w2257:dbl)
            n1173 = Absolute Value(x=w2257) -> (abs(x)=w2256:dbl)
            n1174 = Initialize Array(sgl 0.0 ("element"), w2231) -> (w2239:sgl[])
            n1175 = Divide(x=w2256, y=w2231) -> (x/y=w2253:dbl)
            n1176 = Subtract(x=w2248, y=w2247) -> (x-y=w2249:dbl)
            n1177 = Absolute Value(x=w2249) -> (abs(x)=w2246:dbl)
            n1178 = Divide(x=w2246, y=w2245) -> (x/y=w2244:dbl)
            n1179 = property on="Spectrum" class="WFGraph (strict)"("Value"=w2239, "XScale.Offset"=w2255, "XScale.Multiplier"=w2253, "XScale.ScaleFit"=u8 1 ("X Scale.Scale Fit")) -> ()  [unwired: 2 in, 2 out]
            n1180 = Add(x=w2244, y=10.0) -> (x+y=w2229:dbl)
            n1181 = Round Toward +Infinity(x=w2229) -> (ceil(x): smallest int >= x=w2243:dbl)
            n1182 = call "Add actual date time to string.vi"("String in"="Preparing for measurement") -> ("String out"=w2280:string)  [unwired: 4 in]
            n1183 = Initialize Array(sgl 0.0 ("element"), w2243, w2231) -> (w2241:sgl[][])
            n1184 = call "Add line to map.vi"("Initial"=w2241, "reset(f)"=TRUE ("reset")) -> ()  [unwired: 7 in, 3 out]
            n1185 = call "simple Shift string array.vi"("Element in"=w2280, "Array in"=w2279) -> ("Array out"=w2277:string[])  [unwired: 8 in, 1 out]
            n1186 = Select(t=experiment_state."Setup", s=w2261, f=experiment_state."Stabilization" ("Value")) -> (s? t:f=w2270:T25)
            n1187 = property on="EPR map" class="IntGraph (strict)"("Value"=w2241, "XScale.Multiplier"=w2253, "XScale.Offset"=w2255, "YScale.Multiplier"=w2245, "YScale.Offset"=w2248, "XScale.ScaleFit"=w2250, "YScale.ScaleFit"=w2250) -> ()  [unwired: 2 in, 2 out]
            n1188 = Bundle By Name(cluster=w2275, "Experiment state"=w2270) -> (w2276:T24)
            "VTI tmp reached" <- FALSE ("VTI tmp reached")
            "Tmp reched time" <- u32 0 ("Tmp reched time")
          }
          frame "Stabilization" {
            n1189 = local read "VTI tmp reached"() -> (w2306:bool)
            n1190 = Unbundle By Name(w2292) -> ("Magnet.Field [T]"=w2287:dbl, "VTI.VTI [K]"=w2291:dbl)
            n1191 = Unbundle By Name(w2294) -> ("B_start[T]"=w2288:dbl, "Tmp [K]"=w2308:dbl, "Wait[min]"=w2290:dbl)
            n1192 = Not(x=w2306) -> (.not. x?=w2304:bool)
            n1193 = call "Is equal in tolerance.vi"("Absolut tolerance"=0.5, "Reference value"=w2308, "Input value"=w2291) -> ("Is in range"=w2303:bool)  [unwired: 1 in]
            n1194 = And(x=w2303, y=w2304) -> (x .and. y?=w2305:bool)
            n1195 = case shown="False" w2305 {
              tunnel: w2303 -> [w2330 _]
              tunnel: w2290 -> [w2329 w2342]
              tunnel: [w2328 FALSE] -> w2302
              tunnel: [w2327 w2342] -> w2289
              frame False {
                n1196 = case shown="True" w2330 {
                  selector: w2330 -> [w2332 _]
                  tunnel: w2329 -> [w2331 w2337]
                  tunnel: [w2332 w2335] -> w2328
                  tunnel: [w2331 w2333] -> w2327
                  frame False {
                    n1197 = local write "VTI tmp reached"(w2332) -> ()
                  }
                  frame True {
                    n1198 = local read "Tmp reched time"() -> (w2341:dbl)
                    n1199 = Get Date/Time In Seconds() -> (seconds since 1Jan1904=w2334:timestamp)
                    n1200 = To Double Precision Float(number=w2334) -> (double precision float=w2339:dbl)
                    n1201 = Multiply(x=w2337, y=60.0) -> (x*y=w2336:dbl)
                    n1202 = Subtract(x=w2339, y=w2341) -> (x-y=w2338:dbl)
                    n1203 = Subtract(x=w2336, y=w2338) -> (x-y=w2333:dbl)
                    n1204 = Less Or Equal To 0?(x=w2333) -> (x <= 0?=w2335:bool)
                  }
                }
              }
              frame True {
                n1205 = Get Date/Time In Seconds() -> (seconds since 1Jan1904=w2344:timestamp)
                n1206 = To Double Precision Float(number=w2344) -> (double precision float=w2343:dbl)
                n1207 = local write "VTI tmp reached"(TRUE ("VTI tmp reached")) -> ()
                n1208 = local write "Tmp reched time"(w2343) -> ()
              }
            }
            n1209 = call "Is equal in tolerance.vi"("Absolut tolerance"=0.001, "Reference value"=w2288, "Input value"=w2287) -> ("Is in range"=w2286:bool)  [unwired: 1 in]
            n1210 = Compound Arithmetic op=AND(w2286, w2302) -> (w2301:bool)
            n1211 = case shown="True" w2301 {
              tunnel: w2294 -> [w2309 w2317]
              tunnel: w2300 -> [_ w2318]
              tunnel: w2299 -> [w2311 w2324]
              tunnel: [w2311 w2323] -> w2298
              tunnel: [experiment_state."Stabilization" ("Value") w2321] -> w2295
              tunnel: [w2309 w2317] -> w2293
              frame False {
              }
              frame True {
                n1212 = local read "MW trig low [s]"() -> (w2314:dbl)
                n1213 = local read "VID control"() -> (w2316:T16)
                n1214 = Multiply(x=w2314, y=1000.0) -> (x*y=w2313:dbl)
                n1215 = call "Add actual date time to string.vi"("String in"="Starting measurement") -> ("String out"=w2325:string)  [unwired: 4 in]
                n1216 = call "simple Shift string array.vi"("Element in"=w2325, "Array in"=w2324) -> ("Array out"=w2323:string[])  [unwired: 8 in, 1 out]
                n1217 = call "Begin map measurement.vi"("Sweep down\ntime [ms]"=w2313, "VID control"=w2316, "Map parameters"=w2317, "Referencies in"=w2318) -> ("error out"=w2315:errorcluster)  [unwired: 7 in]
                n1218 = Select(t=experiment_state."Save" ("Value"), s=w2315, f=experiment_state."Begin" ("Value")) -> (s? t:f=w2321:T25)
                "Running experiment" <- TRUE ("Running experiment")
              }
            }
            n1219 = Bundle By Name(cluster=w2297, "Remains"=w2289, "Experiment state"=w2295) -> (w2296:T24)
          }
          frame "Begin" {
          }
          frame "Acquisition" {
            n1220 = local read "New data"() -> (w2353:bool)
            n1221 = case shown="True" w2353 {
              selector: w2353 -> [_ w2437]
              tunnel: [FALSE w2445] -> w2361
              tunnel: w2354 -> [_ w2444]
              tunnel: w2352 -> [_ w2441]
              tunnel: w2351 -> [w2363 w2440]
              tunnel: [w2362 w2412] -> w2350
              frame False {
                n1222 = Unbundle By Name(w2363) -> ("Remains"=w2362:dbl)
              }
              frame True {
                n1223 = Not(x=w2437) -> (.not. x?=w2436:bool)
                n1224 = Unbundle By Name(w2444) -> ("Points"=w2389:u32, "Display signal"=w2391:enum16{"X", "Y", "R", "Phi"}, "Signal treat"=w2414:T89, "B_start[T]"=w2418:dbl, "B_End[T]"=w2379:dbl)
                n1225 = local read "Data"() -> (w2392:T5)
                n1226 = Unbundle By Name(w2441) -> ("VTI.VTI [K]"=w2403:dbl, "VTI.Sample [K]"=w2367:dbl, "Magnet.Field [T]"=w2417:dbl, "Magnet.Ramp state"=w2424:T9, "Magnet.Ramp [mT/s]"=w2416:dbl)
                n1227 = local write "New data"(w2436) -> ()
                n1228 = Unbundle By Name(w2440) -> ("Started"=w2439:timestamp)
                n1229 = Unbundle(w2392) -> ("X"=w2370:sgl[], "Y"=w2369:sgl[])
                n1230 = case shown="\"X\", Default" w2391 {
                  tunnel: w2370 -> [w2446 w2449 _]
                  tunnel: w2369 -> [_ w2448 w2450]
                  tunnel: [w2446 w2447 w2450] -> w2385
                  frame "X", Default {
                  }
                  frame "R" {
                    n1231 = Re/Im To Polar(2:w2448, 3:w2449) -> (1:w2447:sgl[])  [unwired: 1 out]
                  }
                  frame "Y" {
                  }
                }
                n1232 = local read "SMU controls"() -> (w2366:T20)
                n1233 = Less?(x=w2418, y=w2379) -> (x < y?=w2427:bool)
                n1234 = local read "data time"() -> (w2443:timestamp)
                n1235 = Quotient & Remainder(x=w2389, y=u32 4096) -> (floor(x/y)=w2386:u32)  [unwired: 1 out]
                n1236 = Less Or Equal To 0?(x=w2386) -> (x <= 0?=w2387:bool)
                n1237 = Select(t=u32 1, s=w2387, f=w2386) -> (s? t:f=w2383:u32)
                n1238 = Select(t=0.001 ("x"), s=w2427, f=-0.001) -> (s? t:f=w2429:dbl)
                n1239 = To Double Precision Float(number=w2439) -> (double precision float=w2438:dbl)
                n1240 = To Double Precision Float(number=w2443) -> (double precision float=w2442:dbl)
                n1241 = call-poly <vilib>:"Decimate (single shot).vi"("averaging"=TRUE, "decimating factor"=w2383, "X"=w2385) -> ("Decimated Array"=w2384:dbl[])  [unwired: 7 in, 1 out]
                n1242 = Unbundle By Name(w2366) -> ("B[T]"=w2365:dbl)
                n1243 = Subtract(x=w2442, y=w2438) -> (x-y=w2433:dbl)
                n1244 = Multiply(x=w2429, y=w2416) -> (x*y=w2431:dbl)
                n1245 = property on="EPR map" class="IntGraph (strict)"() -> ("YScale.Multiplier"=w2394:dbl)  [unwired: 2 in, 2 out]
                n1246 = Equal?(x=w2424, y=RampingOutput."At Target" ("Magnet.Ramp state")) -> (x = y?=w2425:bool)
                n1247 = Multiply(x=w2433, y=w2431) -> (x*y=w2395:dbl)
                n1248 = call "Normalize 1D float array.vi"("Signal treat"=w2414, "Data in"=w2384) -> ("Data out"=w2413:sgl[])  [unwired: 9 in]
                n1249 = Add(x=w2395, y=w2418) -> (x+y=w2396:dbl)
                n1250 = local read "tdms map file out"() -> (w2409:refnum<k34>)
                n1251 = Subtract(x=w2396, y=w2379) -> (x-y=w2421:dbl)
                n1252 = local read "Counter"() -> (w2380:u32)
                n1253 = Divide(x=w2395, y=w2394) -> (x/y=w2393:dbl)
                n1254 = local read "Acquisition controls"() -> (w2430:T15)
                n1255 = Unbundle By Name(w2430) -> ("Modulation [A]"=w2402:dbl)
                n1256 = Absolute Value(x=w2421) -> (abs(x)=w2422:dbl)
                n1257 = Build Array(w2396) -> (w2411:dbl[])
                n1258 = Divide(x=w2422, y=w2416) -> (x/y=w2420:dbl)
                n1259 = call "Is equal in tolerance.vi"("Absolut tolerance"=0.01, "Reference value"=w2379, "Input value"=w2417) -> ("Is in range"=w2435:bool)  [unwired: 1 in]
                n1260 = Format Into String(w2380) -> (resulting string=w2371:string)  [unwired: 3 in, 1 out]
                n1261 = call "Add line to map.vi"("Field index"=w2393, "FDMR array"=w2413) -> ("cols"=w2397:i32, "rows"=w2398:i32, "Map"=w2415:sgl[][])  [unwired: 7 in]
                n1262 = TDMS Write(0:w2409, 5:"Aux data" ("group name in (Untitled)"), 7:"Bexp[T]", 9:w2411) -> (4:w2406:refnum<k34>, 6:w2368:string, 15:w2407:errorcluster)  [unwired: 2 in, 1 out]
                n1263 = And(x=w2425, y=w2435) -> (x .and. y?=w2445:bool)
                n1264 = Increment(x=w2380) -> (x+1=w2381:u32)
                n1265 = local read "Tab Control"() -> (w2432:T6)
                n1266 = Build Array(w2402, w2403, w2367, w2417, w2365) -> (w2404:dbl[])
                n1267 = local write "Counter"(w2381) -> ()
                n1268 = Multiply(x=w2420, y=1000.0) -> (x*y=w2412:dbl)
                n1269 = To Single Precision Float(number=w2404) -> (single precision float=w2399:sgl[])
                n1270 = TDMS Write(0:w2406, 5:"X" ("string"), 7:w2371, 9:w2370, 11:w2407) -> (4:w2401:refnum<k34>, 8:w2372:string, 15:w2375:errorcluster)  [unwired: 1 in, 1 out]
                n1271 = case shown="\"MAP measurement\"" w2432 {
                  tunnel: w2384 -> [_ w2452]
                  tunnel: w2415 -> [_ w2451]
                  tunnel: w2398 -> [_ _]
                  tunnel: w2397 -> [_ _]
                  frame "Page Status", Default {
                  }
                  frame "MAP measurement" {
                    "Spectrum" <- w2452
                    "EPR map" <- w2451
                  }
                }
                n1272 = TDMS Write(0:w2401, 5:"Y" ("string"), 7:w2372, 9:w2369, 11:w2375) -> (4:w2376:refnum<k34>, 15:w2374:errorcluster)  [unwired: 1 in, 2 out]
                n1273 = TDMS Write(0:w2376, 1:enum16{"decimated", "interleaved"}."interleaved" ("data layout (0:decimated)"), 5:w2368, 7:string[] ["Modulation", "VTI [K]", "Sample [K]", "Field sweep", "B meas [T]"] ("group name in (Untitled)"), 9:w2399, 11:w2374) -> (4:w2400:refnum<k34>)  [unwired: 3 out]
                n1274 = local write "tdms map file out"(w2400) -> ()
              }
            }
            n1275 = Select(t=experiment_state."Save" ("Value"), s=w2361, f=experiment_state."Acquisition" ("Value")) -> (s? t:f=w2355:T25)
            n1276 = Bundle By Name(cluster=w2357, "Experiment state"=w2355, "Remains"=w2350) -> (w2356:T24)
          }
          frame "Save" {
            n1277 = Unbundle By Name(w2461) -> ("Data_Aq"=w2460:refnum<queue>)
            n1278 = local read "Instr control refs"() -> (w2456:refnum<vi>[])
            n1279 = control-ref of="Map parameters"() -> (w2454:refnum<vi>)
            n1280 = control-ref of="Run MAP btn"() -> (w2455:refnum<vi>)
            n1281 = Bundle By Name(cluster=T47 {"Command"=enum."Set individual parameters", "Data"=variant} ("MSG for  ACQ"), "Data"=T44 {"parameter"=enum."scope_trigEn", "value"=0.0} ("Parameter to set")) -> (w2458:T47)
            n1282 = Build Array (concatenate)(w2455, w2454, w2456) -> (w2457:refnum<vi>[])
            n1283 = call "Put in mailbox.vi"("Message"=w2458, "Queue in"=w2460) -> ()  [unwired: 7 in, 3 out]
            n1284 = call "Dis- or en- able controls.vi"("Disabled"=T32."Enabled", "Control referencies"=w2457) -> ()  [unwired: 9 in, 1 out]
            n1285 = local read "tdms map file out"() -> (w2474:refnum<k34>)
            n1286 = TDMS Close(11:w2474) -> (3:w2465:path)  [unwired: 1 in, 1 out]
            n1287 = flat-sequence {
              frame #0 {
                n1288 = call "Add line to map.vi"("Read? (F)"=TRUE) -> ("cols"=→"cols":i32, "rows"=→"rows":i32)  [unwired: 8 in, 1 out]
              }
              frame #1 {
                n1289 = call "Add line to map.vi"("Initial"=sgl[][] [], "Read? (F)"=FALSE, "reset(f)"=TRUE ("Read? (F)")) -> ()  [unwired: 6 in, 3 out]
              }
            }
            n1290 = Path To String(path=w2465) -> (string=w2464:string)
            n1291 = Bundle By Name(cluster=w2469, "Experiment state"=experiment_state."Setup" ("Value")) -> (w2468:T24)
            n1292 = Concatenate Strings("Measurrement finished " ("String in"), w2464) -> (w2466:string)
            n1293 = call "Add actual date time to string.vi"("String in"=w2466) -> ("String out"=w2473:string)  [unwired: 4 in]
            n1294 = call "simple Shift string array.vi"("Element in"=w2473, "Array in"=w2471) -> ("Array out"=w2470:string[])  [unwired: 8 in, 1 out]
          }
        }
      }
      frame "Stop" {
        n1295 = call "simple Shift string array.vi"("Element in"="Program stopped", "Array in"=w2486) -> ("Array out"=w2485:string[])  [unwired: 8 in, 1 out]
      }
      frame "Restart" {
        n1296 = Build Array("Program restarted") -> (w2491:string[])
      }
    }
    n1297 = Tick Count (ms)() -> (millisecond timer value=w20:u32)
    n1298 = Subtract(x=w20, y=w19) -> (x-y=→"1 round\ntime":u32)
  }
  n1299 = case shown="False" "Real instruments" {
    tunnel: w10 -> [w2502 w2510]
    frame True {
      n1300 = Unbundle By Name(w2502) -> ("Field_M"=w2495:refnum<queue>, "Field_C"=w2497:refnum<queue>, "MW_C"=w2499:refnum<queue>, "Angle_C"=w2500:refnum<queue>, "Table_C"=w2501:refnum<queue>, "Data_Aq"=w2496:refnum<queue>, "Tmp_C"=w2498:refnum<queue>, "TOP"=w2494:refnum<queue>)
      n1301 = call "TemperatureController main.vi"("Supervising module"=w2494, "Controller module"=w2498) -> ()  [unwired: 10 in]
      n1302 = call "Main ACQ module2.vi"("Master mailbox"=w2494, "Module mailbox"=w2496) -> ()  [unwired: 10 in]
      n1303 = call "Servo main.vi"("Queue to UI"=w2494, "Module queue servo"=w2501) -> ()  [unwired: 10 in]
      n1304 = call "PiezoController main.vi"("Top"=w2494, "Rotator"=w2500) -> ()  [unwired: 9 in, 1 out]
      n1305 = call "Module for RF and LO synthesizer.vi"("Main controller mailbox"=w2494, "THz module mailbox"=w2499) -> ()  [unwired: 10 in]
      n1306 = call "MagnetTop.vi"("Queue to UI"=w2494, "Module queue"=w2497) -> ()  [unwired: 10 in]
      n1307 = call "SMU 2450 main.vi"("Mailbox address Top"=w2494, "Module mailbox"=w2495) -> ()  [unwired: 8 in, 2 out]
    }
    frame False {
      n1308 = Unbundle By Name(w2510) -> ("Field_C"=w2505:refnum<queue>, "MW_C"=w2507:refnum<queue>, "Angle_C"=w2508:refnum<queue>, "Table_C"=w2509:refnum<queue>, "Data_Aq"=w2504:refnum<queue>, "Tmp_C"=w2506:refnum<queue>, "TOP"=w2503:refnum<queue>)
      n1309 = call "Fake VTI module.vi"("Top address in"=w2503, "VTI Module ref"=w2506) -> ()  [unwired: 10 in]
      n1310 = call "fake lock-in module.vi"("Master mailbox"=w2503, "Module mailbox"=w2504) -> ()  [unwired: 10 in]
      n1311 = call "fake Servo modue.vi"("Queue to UI"=w2503, "Module queue servo"=w2509) -> ()  [unwired: 10 in]
      n1312 = call "fake SampleRotator module.vi"("Top"=w2503, "Rotator"=w2508) -> ()  [unwired: 8 in, 2 out]
      n1313 = call "fake THz module.vi"("Main controller mailbox"=w2503, "THz module mailbox"=w2507) -> ()  [unwired: 10 in]
      n1314 = call "fake main magnet module.vi"("Queue to UI"=w2503, "Module queue"=w2505) -> ()  [unwired: 10 in]
    }
  }
  n1315 = flat-sequence {
    tunnel: w5 -> [_]
    frame #0 {
      n1316 = Stop(stop? (T)=TRUE) -> ()
    }
  }
